vi "DL-SMART-MS-MOTOR-TEST.vi"() -> ()   [LabVIEW 2013]
uses:
  <userlib>/caLab/Private/Put_DBL-1D_PV.vi
  <resource>/objmgr/imaqdx.rc
  <vilib>/Utility/file.llb/Write To Spreadsheet File (DBL).vi
  <userlib>/caLab/Private/Put_I32_PV.vi
  <userlib>/caLab/Private/Get_PV.vi
  <vilib>/Analysis/NI_AALPro.lvlib
  cal_p.vi
  <vilib>/Utility/file.llb/Read From Spreadsheet File (DBL).vi
  <vilib>/Utility/config.llb/NI_LVConfig.lvlib
  <vilib>/Utility/config.llb/Write Key (Double).vi
  <vilib>/Utility/config.llb/Read Key (Double).vi
  <vilib>/Utility/config.llb/Write Key (U32).vi
  <vilib>/Utility/config.llb/Read Key (U32).vi
  <vilib>/Utility/config.llb/Config Data RefNum.ctl
panel:
  out "config":T1 caption="引用句柄"
  in  "stop":bool=TRUE
  out "idn status":string
  out "std sample":T2(array[cluster])
  out "Image":T3(plugin-control)
  out "selected id":i32
  out "selected row":i32
  out "currentNO":string
  out "commet":string
  out "sampleID":string
  in  "chamber in":bool caption="TakeMS"
  in  "chamber out":bool caption="TakeMS"
  in  "ShutDownSystem":bool
  in  "ADC reference":refnum<vi>
  out "Pul.HV-Real":dbl
  out "Identify Spcetrum":cluster{"ID1:X":dbl[], "ID1:Y":dbl[]}[](graph)
  in  "测试记录":i32(listbox)=6
  in  "Identification Results (单靶鉴定结果)":i32(listbox)=2
  in  "HVEnable":bool
  out "GateClose":bool
  out "LaserOK":bool
  out "HV-OK":bool
  out "Vacuum-OK":bool
  in  "Tab Control":T4(tab)
  in  "MCPHV-Set":dbl=1400.0 min=0.0 max=1600.0
  in  "LensHV-Set":dbl=8000.0 min=0.0 max=10000.0
  in  "Tar.HV-Set":dbl=18010.0 min=0.0 max=20000.0
  in  "Pul.HV-Set":dbl=1400.0 min=0.0 max=2000.0
  in  "PulseDelay":dbl
  in  "ADCFreq":dbl
  in  "CH1_Coupling":u64(ring)=2 items=["Volt DC"=1, "Volt AC"=2, "Ampere DC"=4, "Ampere AC"=8, "Ohm"=16]
  in  "Channel 1_Range":dbl(ring)=4.0 items=["80 V"=80.0, "40 V"=40.0, "20 V"=20.0, "8 V"=8.0, "4 V"=4.0, "2 V"=2.0, "800 mV"=0.8, "400 mV"=0.4, "200 mV"=0.2]
  in  "Anal. Setting File":string="High Mass"
  in  "SettingFileSave":bool caption="TakeMS"
  in  "SettingFileAppl":bool caption="TakeMS"
  in  "SettingDel":bool caption="TakeMS"
  in  "RunADC":bool caption="TakeMS"
  in  "Vac_Prot.":bool
  in  "Turbo_Fore":bool
  in  "Main_Samp":bool
  in  "Samp_Atmos":bool
  in  "Fore_Samp":bool
  in  "StartPump":bool
  in  "SopPump":bool
  in  "laser OFF":bool
  in  "laser ON":bool
  in  "laser Deactive":bool
  out "A1-position-Y":dbl=45.0 caption="Y" min=0.0 max=55.0
  out "A1-position-X":dbl=53.4 caption="X" min=0.0 max=55.0
  in  "GO":bool
  in  "Y":dbl min=0.0 max=55.0
  in  "X":dbl min=0.0 max=55.0
  in  "A1-Position":bool caption="X-"
  in  "Plat_To_Zero":bool caption="TakeMS"
  in  "Plat_Cal":bool caption="TakeMS"
  out "Y当前":dbl
  out "X当前":dbl
  out "移动":bool
  out "Y满":bool
  out "Y标":bool
  out "X满":bool
  out "Y0":bool
  out "X0":bool
  out "靶位In/Out":bool
  out "仓门":bool
  out "Y过热":bool
  out "X过热":bool
  out "通讯":bool
  in  "Operation Record":i32(listbox)
  in  "OptionRecordLoad 2":bool caption="TakeMS"
  in  "OptionRecordClear":bool caption="TakeMS"
  out "c:":dbl
  out "b:":dbl
  out "a:":dbl
  in  "cancel cal":bool
  in  "cal save":bool
  in  "peak cal":bool
  in  "peak detect":bool
  in  "标准样品":u16(ring) items=["肺炎克雷伯菌", "铜绿假单胞菌"]
  in  "定标参数":i32(listbox)
  out "Tar.HV-Real":dbl
  out "LensHV-Real":dbl
  out "MCPHV-Real":dbl
  out "Lvaccum":dbl=0.83 format="%#_2e"
  out "Hvaccum":dbl=3.4e-05 format="%#_2e"
  in  "H12":bool
  in  "G12":bool
  in  "F12":bool
  in  "E12":bool
  in  "D12":bool
  in  "C12":bool
  in  "B12":bool
  in  "A12":bool
  in  "H11":bool
  in  "G11":bool
  in  "F11":bool
  in  "E11":bool
  in  "D11":bool
  in  "C11":bool
  in  "B11":bool
  in  "A11":bool
  in  "H10":bool
  in  "G10":bool
  in  "F10":bool
  in  "E10":bool
  in  "D10":bool
  in  "C10":bool
  in  "B10":bool
  in  "A10":bool
  in  "H9":bool
  in  "G9":bool
  in  "F9":bool
  in  "E9":bool
  in  "D9":bool
  in  "C9":bool
  in  "B9":bool
  in  "A9":bool
  in  "H8":bool
  in  "G8":bool
  in  "F8":bool
  in  "E8":bool
  in  "D8":bool
  in  "C8":bool
  in  "B8":bool
  in  "A8":bool
  in  "H7":bool
  in  "G7":bool
  in  "F7":bool
  in  "E7":bool
  in  "D7":bool
  in  "C7":bool
  in  "B7":bool
  in  "A7":bool
  in  "H6":bool
  in  "G6":bool
  in  "F6":bool
  in  "E6":bool
  in  "D6":bool
  in  "C6":bool
  in  "B6":bool
  in  "A6":bool
  in  "H5":bool
  in  "G5":bool
  in  "F5":bool
  in  "E5":bool
  in  "D5":bool
  in  "C5":bool
  in  "B5":bool
  in  "A5":bool
  in  "H4":bool
  in  "G4":bool
  in  "F4":bool
  in  "E4":bool
  in  "D4":bool
  in  "C4":bool
  in  "B4":bool
  in  "A4":bool
  in  "H3":bool
  in  "G3":bool
  in  "F3":bool
  in  "E3":bool
  in  "D3":bool
  in  "C3":bool
  in  "B3":bool
  in  "A3":bool
  in  "H2":bool
  in  "G2":bool
  in  "F2":bool
  in  "E2":bool
  in  "D2":bool
  in  "C2":bool
  in  "B2":bool
  in  "A2":bool
  in  "H1":bool
  in  "G1":bool
  in  "F1":bool
  in  "E1":bool
  in  "D1":bool
  in  "C1":bool
  in  "B1":bool
  in  "A1":bool
  in  "Clear":bool caption="TakeMS"
  in  "Add":bool caption="TakeMS"
  in  "TakeMS-Stop":bool caption="TakeMS"
  in  "TakeMS-Run":bool caption="TakeMS"
  # "Laser (激光)"
  # "光栅"
  # "uJ"
  # "Acq.(采谱)"
  # "Vacuum(真空)"
  # "1"
  # "2"
  # "3"
  # "4"
  # "5"
  # "6"
  # "7"
  # "8"
  # "9"
  # "10"
  # "11"
  # "12"
  # "A"
  # "Pa"
  # "High"
  # "B"
  # "Low"
  # "Pa"
  # "C"
  # "H.V.(高压)"
  # "D"
  # "MCP"
  # "V"
  # "E"
  # "Tar."
  # "V"
  # "F"
  # "Pul."
  # "V"
  # "G"
  # "Lens"
  # "V"
  # "H"
  # "Vauum (真空)"
  # "H.V. (高压)"
  # "Laser (激光)"
  # "Gate (仓门)"
  # "mm"
  # "Radian"
  # "H.V. (高压参数)"
  # "ADC(采集卡设置)"
  # "ADCFreq(采样)"
  # "MCP (探测器)"
  # "V"
  # "Hz"
  # "Tar. (靶)"
  # "V"
  # "Setting File(设置文件)"
  # "Coupling"
  # "Pulse (脉冲)"
  # "V"
  # "IntRange"
  # "V"
  # "Lens (透镜)"
  # "Delay (延时)"
  # "ns"
  # "Sole. Valves"
  # "Turbo Pump"
  # "自锁保护"
  # "机械/分子"
  # "主仓/样仓"
  # "样仓/大气"
  # "机械/样仓"
  # "激光器状态"
  # "mm"
  # "mm"
  # "mm"
  # "mm"
  # "mm"
  # "mm"
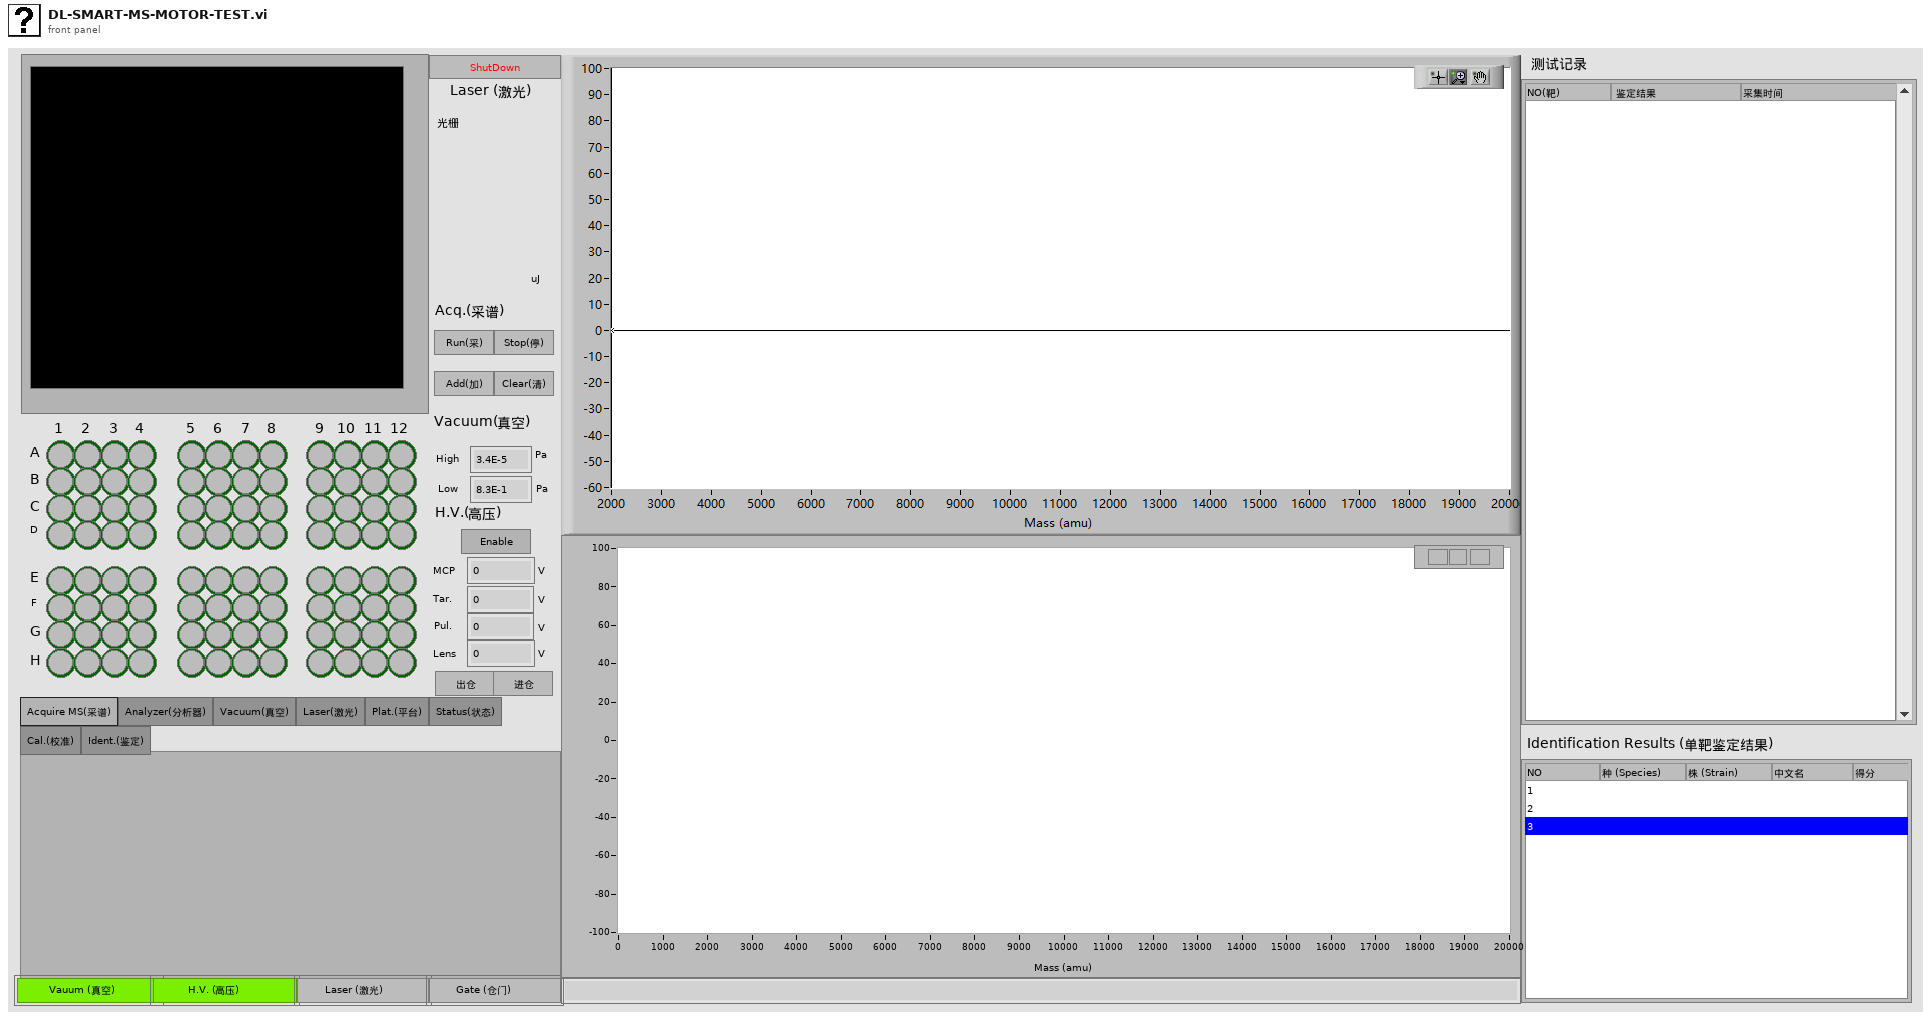
[diagram p1: front panel]
types:
  T1 = typedef "NI_LVConfig.lvlib/Config Data RefNum.ctl" = refnum<k1>
  T2 = cluster{"name":string, "mz":dbl[], "time":dbl[]}[]
  T3 = typedef "IMAQ Image.ctl" = refnum<image>
  T4 = enum32{"Acquire MS(采谱)", "Analyzer(分析器)", "Vacuum(真空)", "Laser(激光)", "Plat.(平台)", "Status(状态)", "Cal.(校准)", "Ident.(鉴定)"}
  T5 = cluster{"tag1":string, "tag2":string, "x":dbl[], "y":dbl[], "ID1:X":dbl[], "ID1:Y":dbl[], "ID1:REF:X":dbl[], "ID1:REF:Y":dbl[], "ID2:X":dbl[], "ID2:Y":dbl[], "ID2:REF:X":dbl[], "ID2:REF:Y":dbl[], "ID3:X":dbl[], "ID3:Y":dbl[], "ID3:REF:X":dbl[], "ID3:REF:Y":dbl[], "ID1:TAG1":string, "ID1:TAG2":string, "ID2:TAG1":string, "ID2:TAG2":string, "ID3:TAG1":string, "ID3:TAG2":string, "ID1:NAME":string, "ID2:NAME":string, "ID3:NAME":string, "ID1:SCORE":string, "ID2:SCORE":string, "ID3:SCORE":string, "NO":string}[]
  T6 = enum8{"Enabled", "Disabled", "Disabled and Grayed Out"}
  T7 = typedef "Semaphore RefNum" = refnum<k1>
  T8 = cluster{"monitor":refnum<user-event>, "motor status":refnum<user-event>, "motor":refnum<user-event>, "notifier out":refnum<notifier>, "queue out":refnum<queue>, "AI":T7, "DI":T7, "CX":T7, "CY":T7}
  T9 = cluster{"AI Task":refnum<k21>, "AO Task":refnum<k21>, "DO Task":refnum<k21>, "DI Task":refnum<k21>, "PWM x":refnum<k21>, "PWM y":refnum<k21>, "counter x":refnum<k21>, "counter y":refnum<k21>}
  T10 = cluster{"tasks":cluster{"AI Task":refnum<k21>, "AO Task":refnum<k21>, "DO Task":refnum<k21>, "DI Task":refnum<k21>, "PWM x":refnum<k21>, "PWM y":refnum<k21>, "counter x":refnum<k21>, "counter y":refnum<k21>}, "interface":cluster{"monitor":refnum<user-event>, "motor status":refnum<user-event>, "motor":refnum<user-event>, "notifier out":refnum<notifier>, "queue out":refnum<queue>, "AI":T7, "DI":T7, "CX":T7, "CY":T7}, "error out":errorcluster}
  T11 = typedef "LVPoint32TypeDef.ctl" = cluster{"Horizontal":i32, "Vertical":i32}
  T12 = cluster{"tag1":string, "tag2":string, "x":dbl[], "y":dbl[], "ID1:X":dbl[], "ID1:Y":dbl[], "ID1:REF:X":dbl[], "ID1:REF:Y":dbl[], "ID2:X":dbl[], "ID2:Y":dbl[], "ID2:REF:X":dbl[], "ID2:REF:Y":dbl[], "ID3:X":dbl[], "ID3:Y":dbl[], "ID3:REF:X":dbl[], "ID3:REF:Y":dbl[], "ID1:TAG1":string, "ID1:TAG2":string, "ID2:TAG1":string, "ID2:TAG2":string, "ID3:TAG1":string, "ID3:TAG2":string, "ID1:NAME":string, "ID2:NAME":string, "ID3:NAME":string, "ID1:SCORE":string, "ID2:SCORE":string, "ID3:SCORE":string, "NO":string}
  T13 = typedef "LVRowAndColumnTypeDef.ctl" = cluster{"Row":i32, "Column":i32}
  T14 = cluster{"Type":u32, "Version":u32, "Flags":u32, "SerialNumberHigh":u32, "SerialNumberLow":u32, "BusType":u32, "InterfaceName":string, "VendorName":string, "ModelName":string, "CameraFileName":string, "CameraAttributeURL":string}[]
  T15 = cluster{"Type":u32, "Version":u32, "Flags":u32, "SerialNumberHigh":u32, "SerialNumberLow":u32, "BusType":u32, "InterfaceName":string, "VendorName":string, "ModelName":string, "CameraFileName":string, "CameraAttributeURL":string}
  T16 = typedef "IMAQdx.ctl" = refnum<k21>
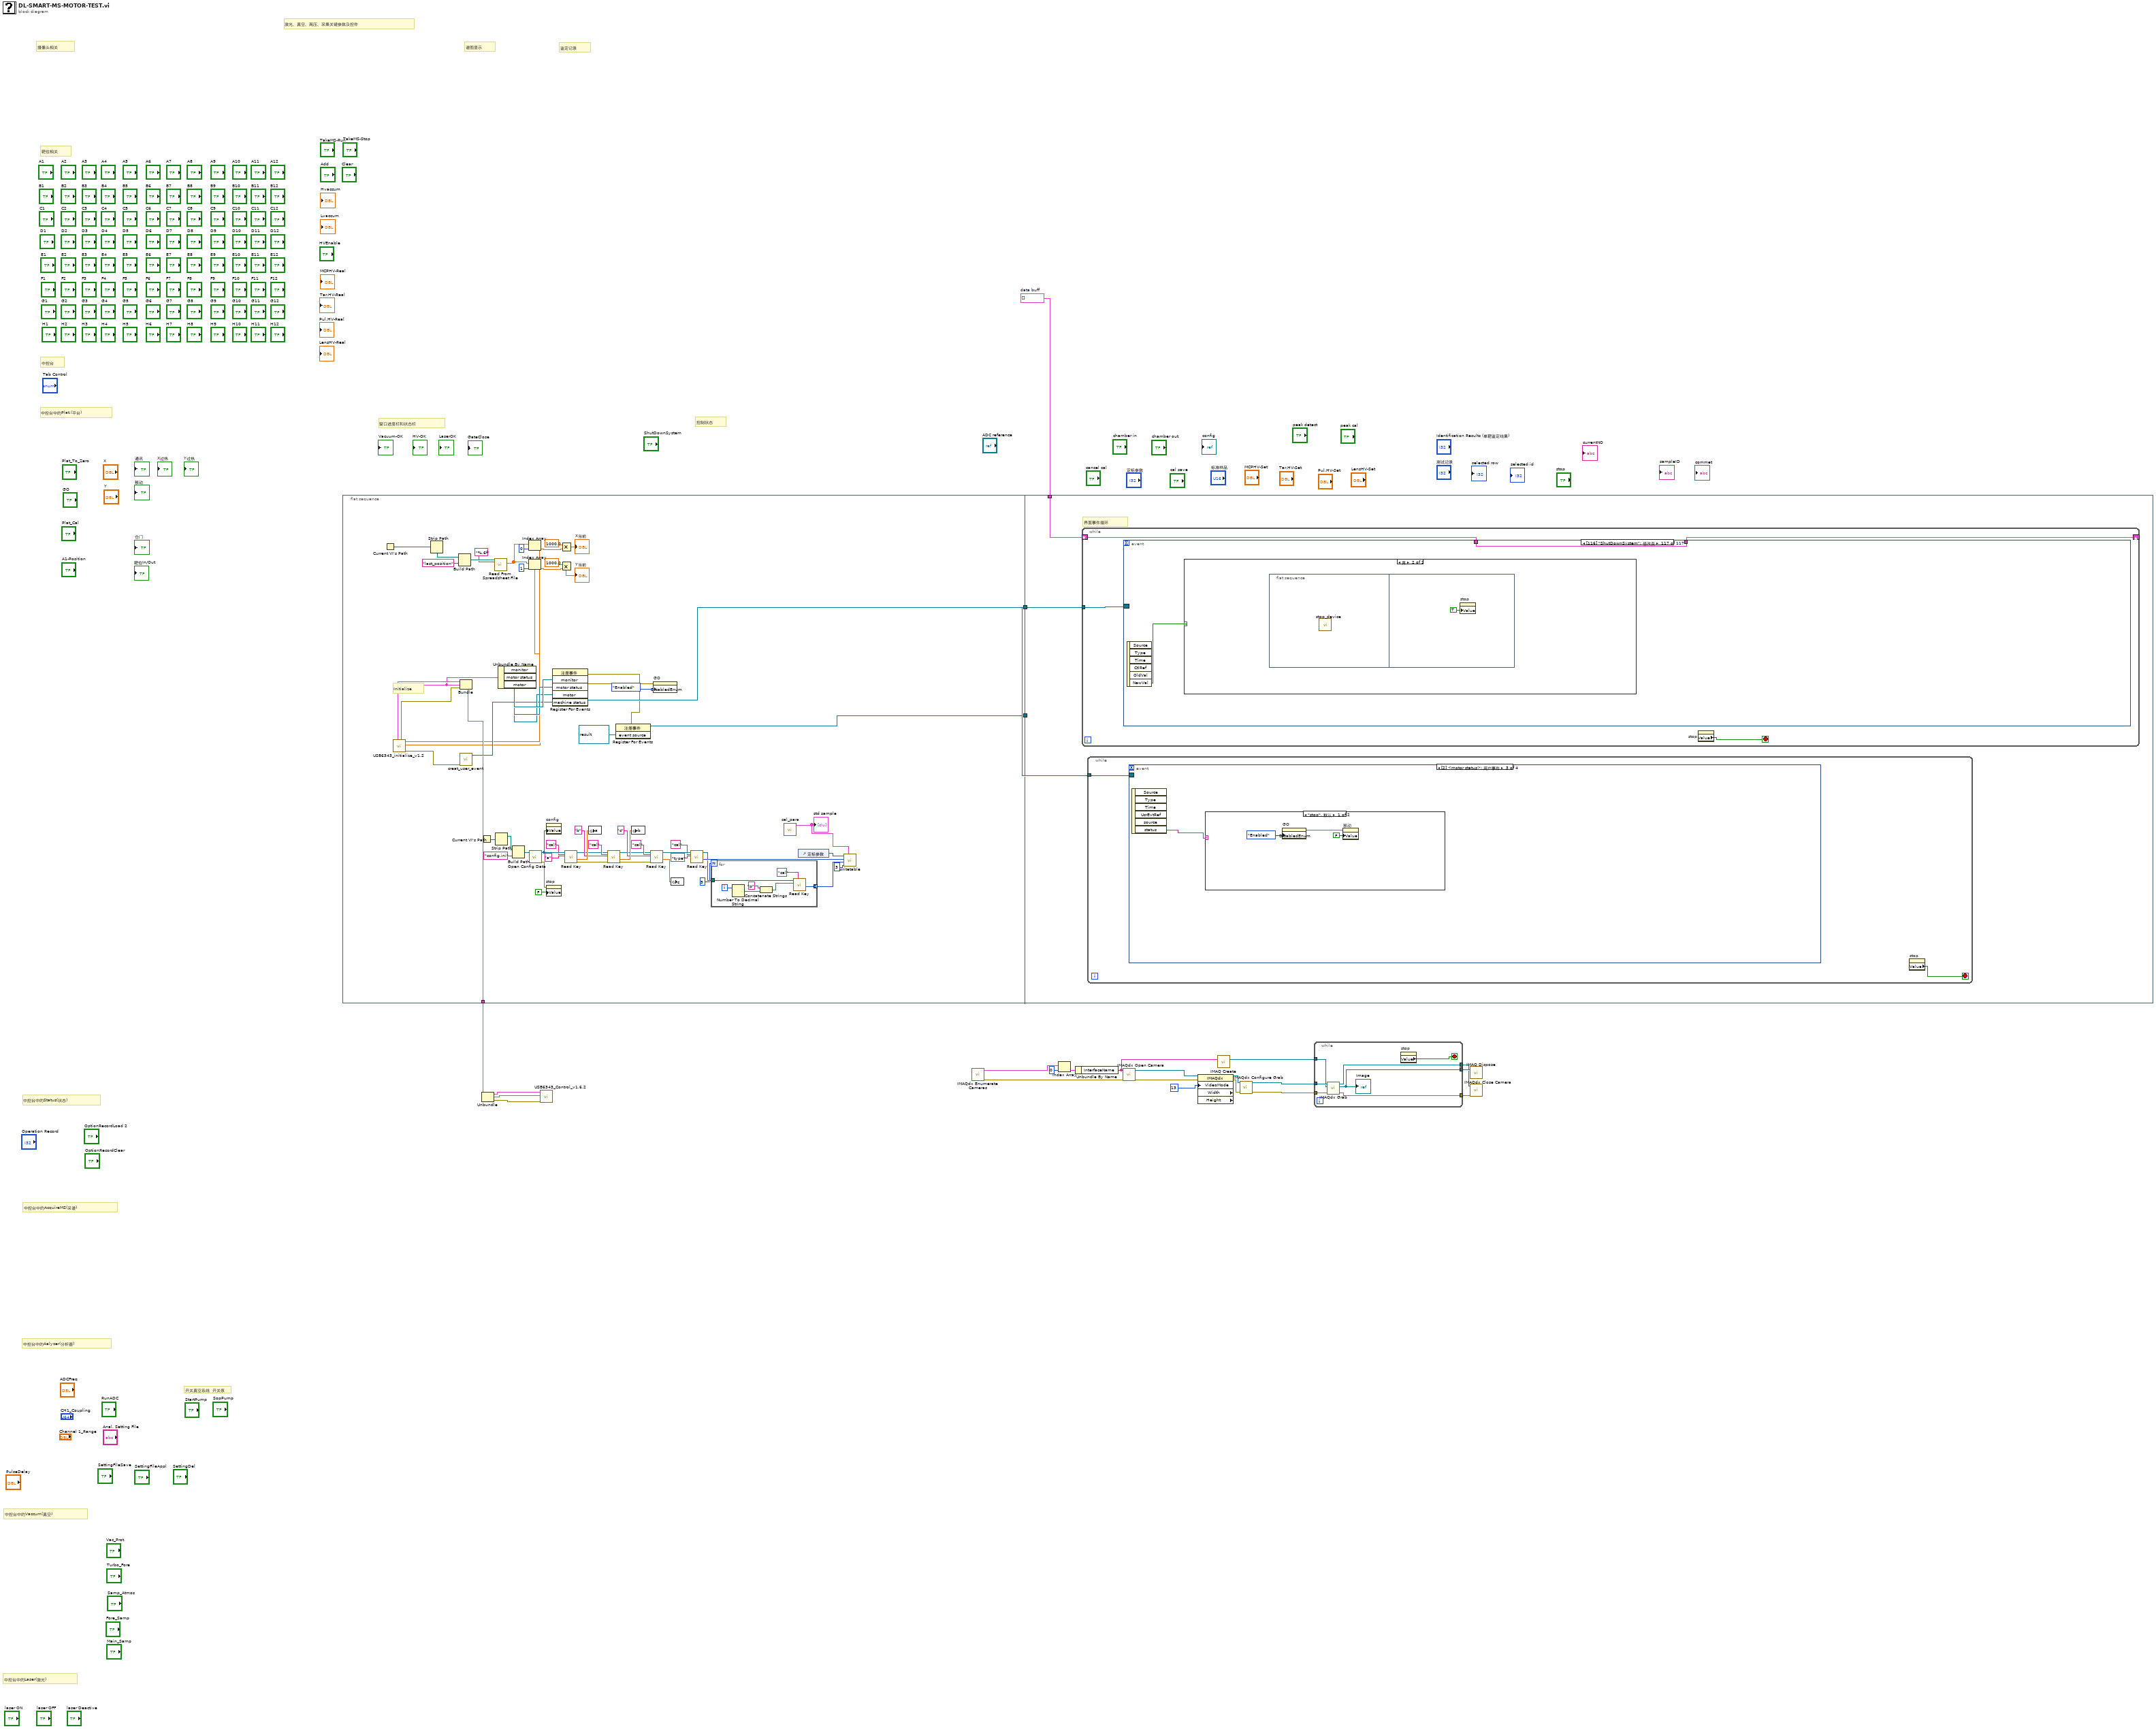
[diagram p0: block diagram]
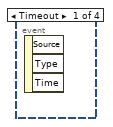
[diagram p2: hidden frame]
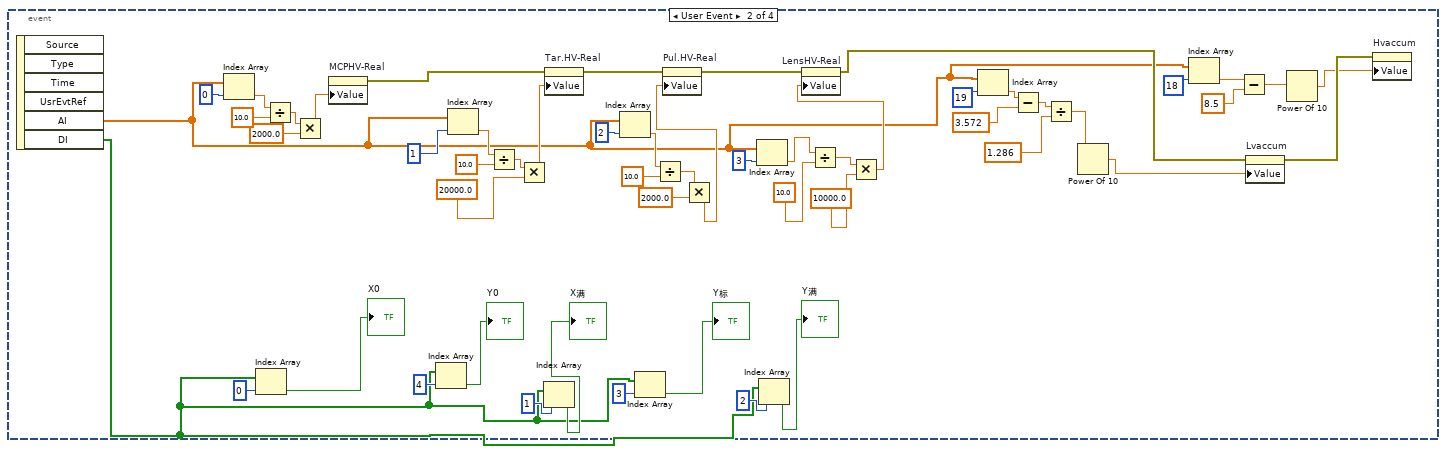
[diagram p3: hidden frame]
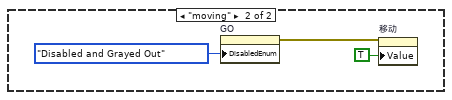
[diagram p4: hidden frame]
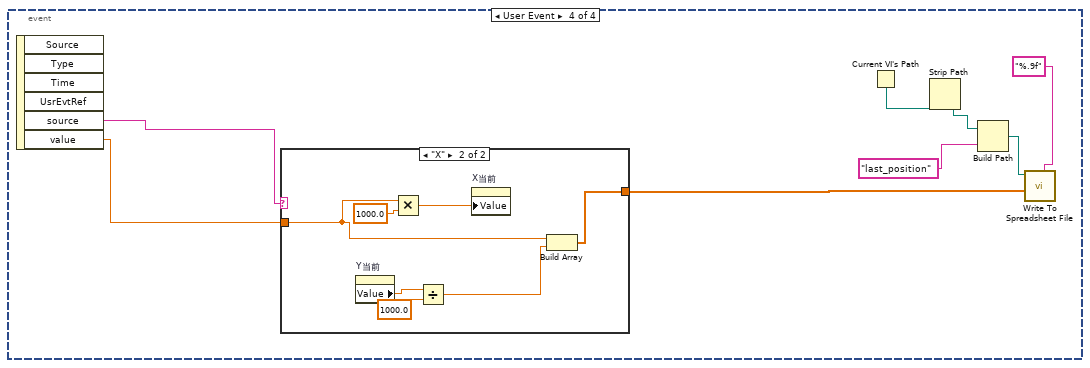
[diagram p5: hidden frame]
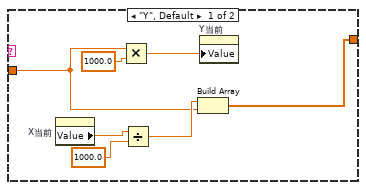
[diagram p6: hidden frame]
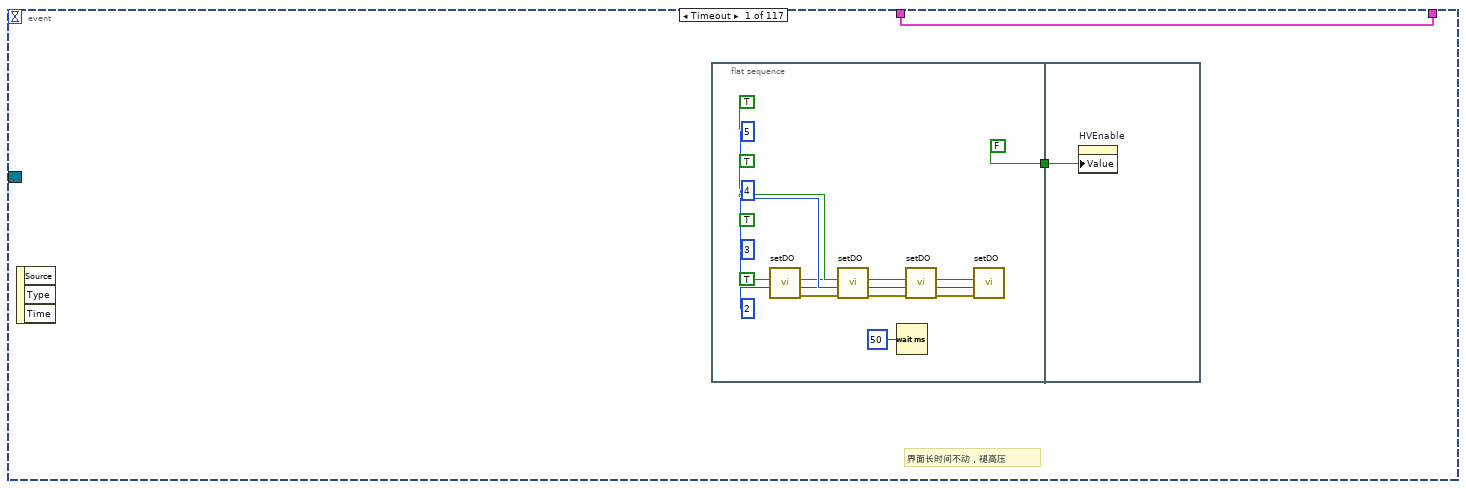
[diagram p7: hidden frame]
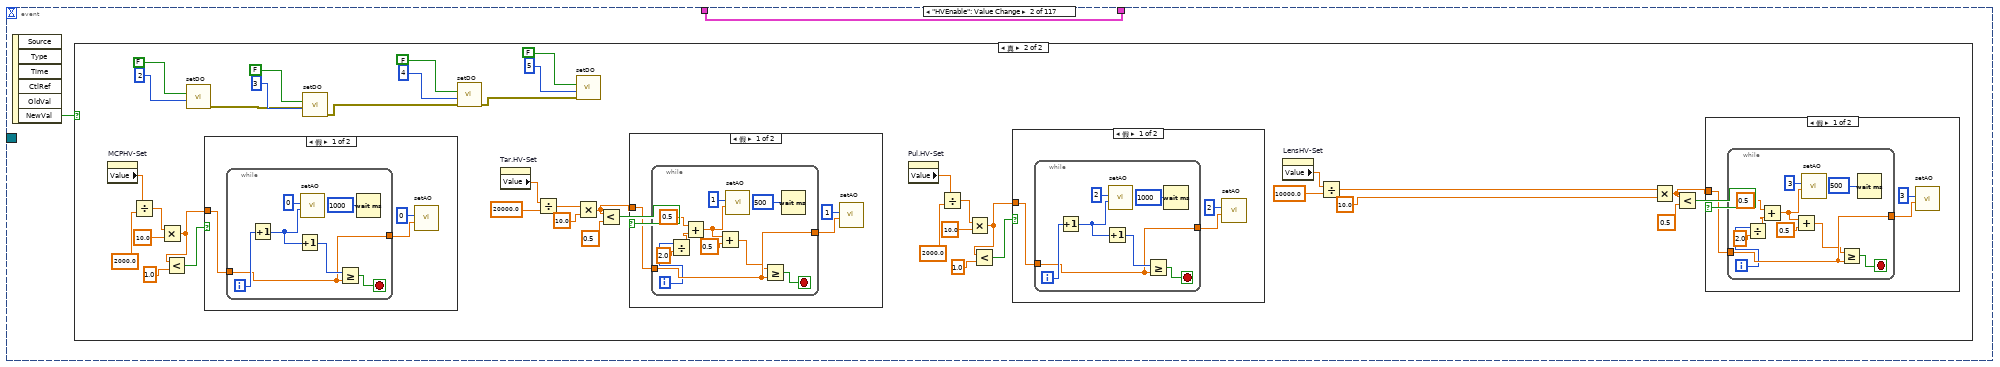
[diagram p8: hidden frame]
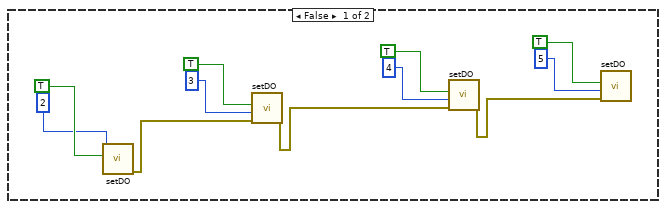
[diagram p9: hidden frame]
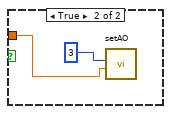
[diagram p10: hidden frame]
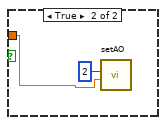
[diagram p11: hidden frame]
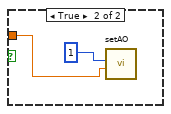
[diagram p12: hidden frame]
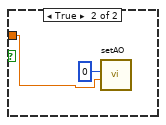
[diagram p13: hidden frame]
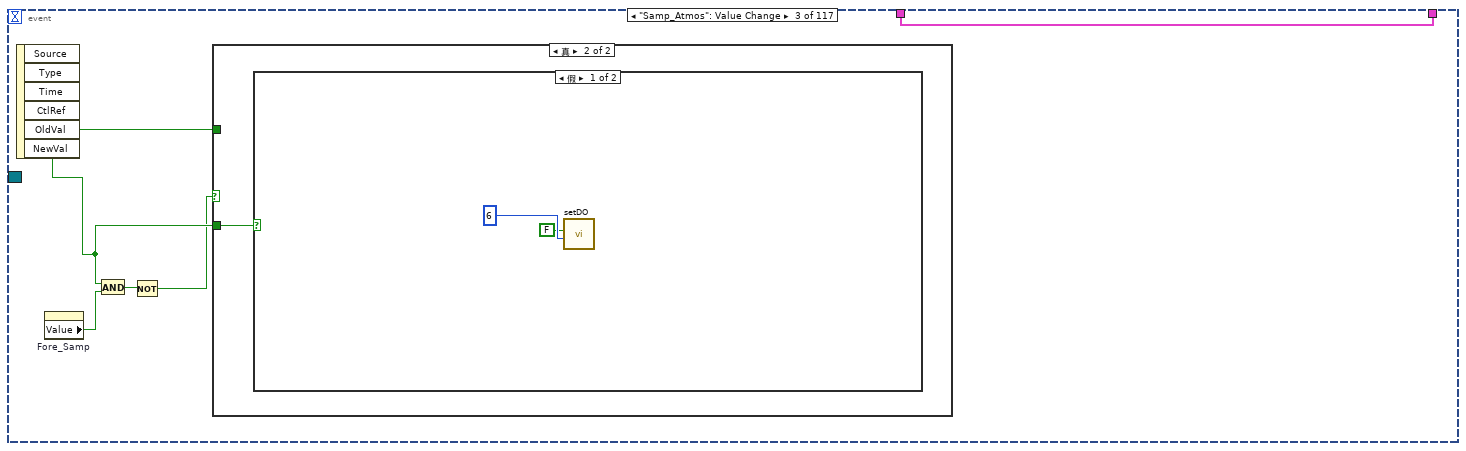
[diagram p14: hidden frame]
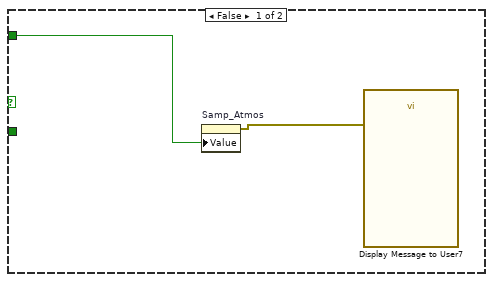
[diagram p15: hidden frame]
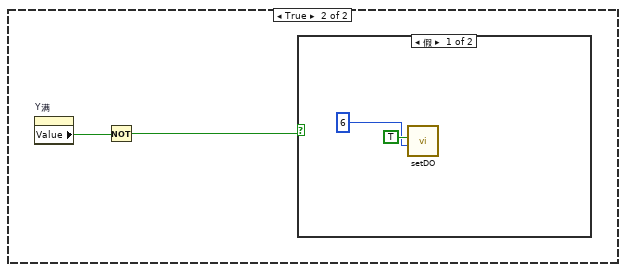
[diagram p16: hidden frame]
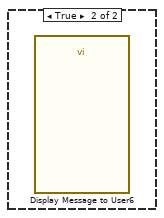
[diagram p17: hidden frame]
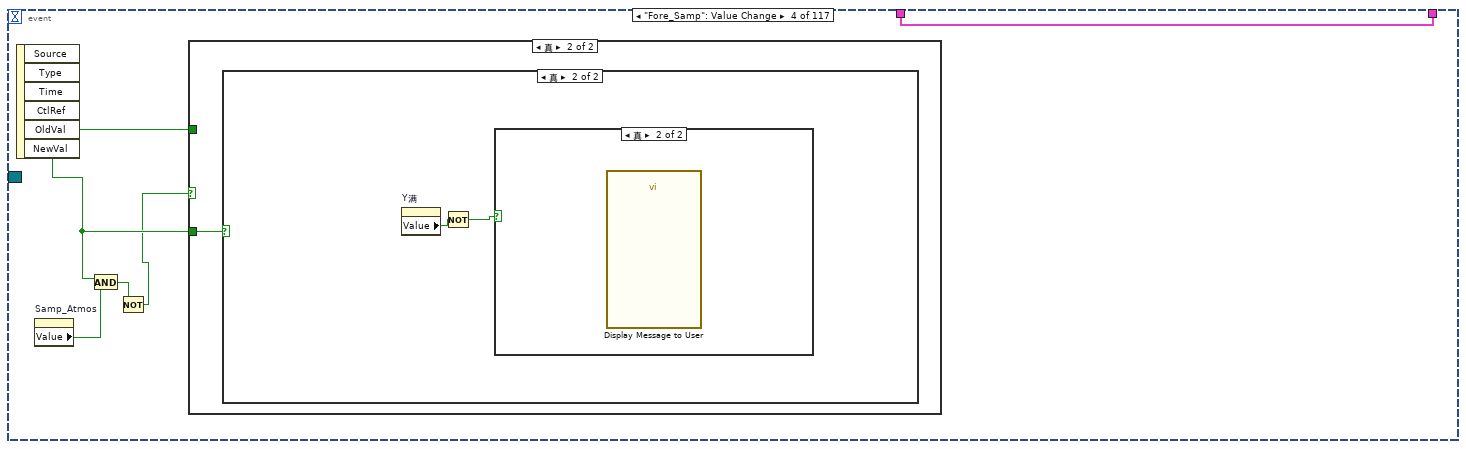
[diagram p18: hidden frame]
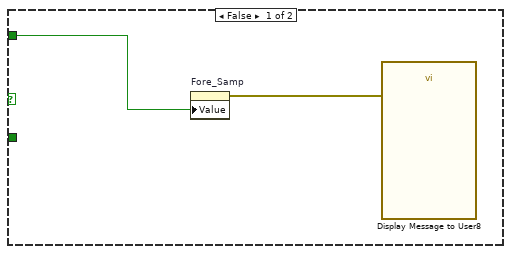
[diagram p19: hidden frame]
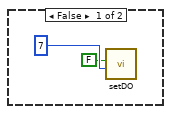
[diagram p20: hidden frame]
diagram:
  w21 = T5 []  # data buff
  # "开关真空系统  开关泵"
  # "控制状态"
  # "鉴定记录"
  # "谱图显示"
  # "激光、真空、高压、采集关键参数及控件"
  # "窗口进度栏和状态栏"
  # "中控台中的Laser(激光)"
  # "中控台中的Vaccum(真空)"
  # "中控台中的Aalyzer(分析器)"
  # "中控台中的AcquireMS(采谱)"
  # "中控台中的Status(状态)"
  # "中控台中的Plat.(平台)"
  # "中控台"
  # "靶位相关"
  # "摄像头相关"
  n1 = flat-sequence {
    tunnel: [w58] -> w23
    tunnel: [w73] -> w22
    tunnel: [w53] -> w1
    tunnel: w23 -> [w90]
    tunnel: w21 -> [w91]
    tunnel: w1 -> [w89]
    frame #0 {
      # "Initialize"
      n2 = Current VI's Path() -> (path=w72:path)
      n3 = Strip Path(path=w72) -> (stripped path=w71:path)  [unwired: 1 out]
      n4 = Build Path(base path=w71, name or relative path="last_position") -> (appended path=w69:path)
      n5 = Current VI's Path() -> (path=w50:path)
      n6 = call-poly <vilib>:"Read From Spreadsheet File.vi"("format (%.3f)"="%.6f", "file path (dialog if empty)"=w69) -> ("first row"=w67:dbl[])  [unwired: 5 in, 4 out]
      n7 = Strip Path(path=w50) -> (stripped path=w49:path)  [unwired: 1 out]
      n8 = Build Path(base path=w49, name or relative path="config.ini" ("名称或相对路径")) -> (appended path=w47:path)
      n9 = Index Array(array=w67, index=0) -> (element=w64:dbl)
      n10 = Index Array(array=w67, index=1) -> (element=w61:dbl)
      n11 = call "USB6343_initialize_v1.2.vi"("Y initial position"=w61, "X initial position"=w64) -> ("error out"=w74:errorcluster, "interface"=w75:T8, "tasks"=w76:T9)  [unwired: 7 in]
      n12 = Bundle("tasks"=w76, "interface"=w75, "error out"=w74) -> (w73:T10)  [unwired: 1 in]
      n13 = call "creat_user_event.vi"("error in (no error)"=w74) -> ("machine status"=w77:refnum<user-event>)  [unwired: 9 in, 1 out]
      n14 = Unbundle By Name(w75) -> ("monitor"=w81:refnum<user-event>, "motor status"=w80:refnum<user-event>, "motor"=w79:refnum<user-event>)
      n15 = call <vilib>:"Open Config Data.vi"("configuration file path"=w47) -> ("error out"=w46:errorcluster, "refnum"=w45:T1)  [unwired: 8 in, 1 out]
      n16 = property on="config" class="TypRef (严格)"("Value"=w45) -> ()  [unwired: 2 in, 2 out]
      n17 = property on="stop" class="Bool (严格)"(error in=w46, "Value"=FALSE ("ShutDownSystem")) -> ()  [unwired: 1 in, 2 out]
      n18 = Multiply(x=1000.0, y=w64) -> (x*y=→"X当前":dbl)
      n19 = Multiply(x=1000.0, y=w61) -> (x*y=→"Y当前":dbl)
      n20 = call-poly <vilib>:"Read Key.vi"("section"="cal", "key"="a", "refnum"=w45) -> ("error out"=w37:errorcluster, "value"=w42:dbl, "refnum out"=w38:T1)  [unwired: 5 in, 1 out]
      n21 = global write "cal_p.vi" "a"(w42) -> ()
      n22 = call-poly <vilib>:"Read Key.vi"("section"="cal", "error in (no error)"=w37, "key"="b", "refnum"=w38) -> ("error out"=w33:errorcluster, "value"=w39:dbl, "refnum out"=w32:T1)  [unwired: 4 in, 1 out]
      n23 = register-events(refnum<user-event> refnum ("event source")) -> (reference out=w53:refnum<event-registration>, error out=w52:errorcluster)  [unwired: 2 in]
      n24 = register-events(error in=w52, w81, w80, w79, w77) -> (reference out=w58:refnum<event-registration>, error out=w57:errorcluster)  [unwired: 1 in]
      n25 = global write "cal_p.vi" "b"(w39) -> ()
      n26 = call-poly <vilib>:"Read Key.vi"("section"="cal", "error in (no error)"=w33, "key"="c", "refnum"=w32) -> ("value"=w34:dbl, "refnum out"=w31:T1)  [unwired: 4 in, 2 out]
      n27 = property on="GO" class="Bool (严格)"(error in=w57, "DisabledEnum"=T6."Enabled" ("Disabled")) -> ()  [unwired: 1 in, 2 out]
      n28 = global write "cal_p.vi" "c"(w34) -> ()
      n29 = call-poly <vilib>:"Read Key.vi"("section"="cal", "key"="type", "refnum"=w31) -> ("value"=w28:u32, "refnum out"=w27:T1)  [unwired: 5 in, 2 out]
      n30 = for {
        N: 5 -> [_]
        tunnel: w27 -> [w88]
        tunnel: [w82] -> w25 mode=indexing
        i -> [w86]
        n31 = Number To Decimal String(number=w86) -> (decimal integer string=w85:string)  [unwired: 1 in]
        n32 = Concatenate Strings("p", w85) -> (w83:string)
        n33 = call-poly <vilib>:"Read Key.vi"("section"="cal", "key"=w83, "refnum"=w88) -> ("value"=w82:u32)  [unwired: 5 in, 3 out]
      }
      n34 = call "cal_para.vi"() -> ("std sample"=w55:T2)  [unwired: 11 in]
      "std sample" <- w55
      n35 = control-ref of="定标参数"() -> (w56:refnum<vi>)
      n36 = call "writetable.vi"("std sample"=w55, "col"=3, "Array in"=w25, "type"=w28, "reference"=w56) -> ()  [unwired: 7 in]
    }
    frame #1 {
      # "界面事件循环"
      n37 = while {
        tunnel: w89 -> [w179]
        shift-right: [w177] -> _
        shift-left: w91 -> [w178]
        stop <- w176 stop-if-true
        n38 = event shown="[116] \"ShutDownSystem\": 值改变" {
          selector: w179 -> [_ _ _ _ _ _ _ _ _ _ _ _ _ _ _ _ _ _ _ _ _ _ _ _ _ _ _ _ _ _ _ _ _ _ _ _ _ _ _ _ _ _ _ _ _ _ _ _ _ _ _ _ _ _ _ _ _ _ _ _ _ _ _ _ _ _ _ _ _ _ _ _ _ _ _ _ _ _ _ _ _ _ _ _ _ _ _ _ _ _ _ _ _ _ _ _ _ _ _ _ _ _ _ _ _ _ _ _ _ _ _ _ _ _ _ _ _]
          dyn-events: _ -> [_ _ _ _ _ _ _ _ _ _ _ _ _ _ _ _ _ _ _ _ _ _ _ _ _ _ _ _ _ _ _ _ _ _ _ _ _ _ _ _ _ _ _ _ _ _ _ _ _ _ _ _ _ _ _ _ _ _ _ _ _ _ _ _ _ _ _ _ _ _ _ _ _ _ _ _ _ _ _ _ _ _ _ _ _ _ _ _ _ _ _ _ _ _ _ _ _ _ _ _ _ _ _ _ _ _ _ _ _ _ _ _ _ _ _ _ _]
          timeout: _ -> [_ _ _ _ _ _ _ _ _ _ _ _ _ _ _ _ _ _ _ _ _ _ _ _ _ _ _ _ _ _ _ _ _ _ _ _ _ _ _ _ _ _ _ _ _ _ _ _ _ _ _ _ _ _ _ _ _ _ _ _ _ _ _ _ _ _ _ _ _ _ _ _ _ _ _ _ _ _ _ _ _ _ _ _ _ _ _ _ _ _ _ _ _ _ _ _ _ _ _ _ _ _ _ _ _ _ _ _ _ _ _ _ _ _ _ _ _]
          tunnel: w178 -> [w180 w196 w304 w319 w334 w341 w348 w355 w364 w380 w410 w445 w484 w486 w493 w528 w566 w568 w618 w623 w639 w657 w674 w691 w708 w725 w744 w769 w786 w803 w820 w837 w854 w873 w892 w911 w930 w949 w968 w987 w1006 w1025 w1044 w1063 w1082 w1101 w1120 w1139 w1158 w1177 w1196 w1215 w1234 w1253 w1272 w1291 w1310 w1329 w1348 w1367 w1386 w1405 w1424 w1447 w1466 w1485 w1504 w1523 w1542 w1561 w1580 w1599 w1618 w1637 w1656 w1675 w1694 w1713 w1732 w1751 w1770 w1789 w1808 w1827 w1846 w1865 w1884 w1903 w1922 w1941 w1960 w1979 w1998 w2017 w2036 w2055 w2074 w2093 w2112 w2131 w2150 w2169 w2188 w2207 w2226 w2245 w2264 w2283 w2302 w2321 w2340 w2359 w2378 w2397 w2416 w2435 w2449]
          tunnel: [w180 w196 w304 w319 w334 w341 w348 w355 w364 w379 w410 w445 w484 w486 w493 w528 w566 w568 w618 w623 w639 w657 w674 w691 w708 w725 w743 w769 w786 w803 w820 w837 w854 w873 w892 w911 w930 w949 w968 w987 w1006 w1025 w1044 w1063 w1082 w1101 w1120 w1139 w1158 w1177 w1196 w1215 w1234 w1253 w1272 w1291 w1310 w1329 w1348 w1367 w1386 w1405 w1424 w1447 w1466 w1485 w1504 w1523 w1542 w1561 w1580 w1599 w1618 w1637 w1656 w1675 w1694 w1713 w1732 w1751 w1770 w1789 w1808 w1827 w1846 w1865 w1884 w1903 w1922 w1941 w1960 w1979 w1998 w2017 w2036 w2055 w2074 w2093 w2112 w2131 w2150 w2169 w2188 w2207 w2226 w2245 w2264 w2283 w2302 w2321 w2340 w2359 w2378 w2397 w2416 w2435 w2449] -> w177
          event Timeout {
            # "界面长时间不动，褪高压"
            n39 = event-data() -> ()  [unwired: 1 in, 3 out]
            n40 = flat-sequence {
              tunnel: [FALSE ("HVEnable")] -> w181
              tunnel: w181 -> [w195]
              frame #0 {
                n41 = call "setDO.vi"("channel"=2, "on/off"=TRUE) -> ("错误输出"=w192:errorcluster)  [unwired: 9 in]
                n42 = call "setDO.vi"("错误输入（无错误）"=w192, "channel"=3, "on/off"=TRUE) -> ("错误输出"=w193:errorcluster)  [unwired: 8 in]
                n43 = Wait (ms)(milliseconds to wait=u32 50) -> ()  [unwired: 1 out]
                n44 = call "setDO.vi"("错误输入（无错误）"=w193, "channel"=4, "on/off"=TRUE) -> ("错误输出"=w194:errorcluster)  [unwired: 8 in]
                n45 = call "setDO.vi"("错误输入（无错误）"=w194, "channel"=5, "on/off"=TRUE) -> ()  [unwired: 8 in, 1 out]
              }
              frame #1 {
                n46 = property on="HVEnable" class="Bool (严格)"("Value"=w195) -> ()  [unwired: 2 in, 2 out]
              }
            }
          }
          event "HVEnable": Value Change {
            n47 = event-data() -> ("NewVal"=w197:bool)  [unwired: 1 in, 5 out]
            n48 = case shown="真" w197 {
              frame False {
                n49 = call "setDO.vi"("channel"=2, "on/off"=TRUE) -> ("错误输出"=w200:errorcluster)  [unwired: 9 in]
                n50 = call "setDO.vi"("错误输入（无错误）"=w200, "channel"=3, "on/off"=TRUE) -> ("错误输出"=w199:errorcluster)  [unwired: 8 in]
                n51 = call "setDO.vi"("错误输入（无错误）"=w199, "channel"=4, "on/off"=TRUE) -> ("错误输出"=w198:errorcluster)  [unwired: 8 in]
                n52 = call "setDO.vi"("错误输入（无错误）"=w198, "channel"=5, "on/off"=TRUE) -> ()  [unwired: 8 in, 1 out]
              }
              frame True {
                n53 = property on="MCPHV-Set" class="DigNum (严格)"() -> ("Value"=w233:dbl)  [unwired: 2 in, 2 out]
                n54 = Divide(x=w233, y=2000.0) -> (x/y=w235:dbl)
                n55 = Multiply(x=w235, y=10.0) -> (x*y=w226:dbl)
                n56 = Less?(x=w226, y=1.0) -> (x < y?=w227:bool)
                n57 = call "setDO.vi"("channel"=2, "on/off"=FALSE) -> ("错误输出"=w239:errorcluster)  [unwired: 9 in]
                n58 = case shown="假" w227 {
                  tunnel: w226 -> [w294 w302]
                  frame False {
                    n59 = while {
                      tunnel: w294 -> [w296]
                      tunnel: [w296] -> w292
                      i -> [w300]
                      stop <- w297 stop-if-true
                      n60 = Increment(x=w300) -> (x+1=w299:i32)
                      n61 = Increment(x=w299) -> (x+1=w298:i32)
                      n62 = call "setAO.vi"("value"=w299, "channel"=0) -> ()  [unwired: 9 in, 1 out]
                      n63 = Greater Or Equal?(x=w298, y=w296) -> (x >= y?=w297:bool)
                      n64 = Wait (ms)(milliseconds to wait=1000) -> ()  [unwired: 1 out]
                    }
                    n65 = call "setAO.vi"("value"=w292, "channel"=0) -> ()  [unwired: 9 in, 1 out]
                  }
                  frame True {
                    n66 = call "setAO.vi"("value"=w302, "channel"=0) -> ()  [unwired: 9 in, 1 out]
                  }
                }
                n67 = call "setDO.vi"("错误输入（无错误）"=w239, "channel"=3, "on/off"=FALSE) -> ("错误输出"=w238:errorcluster)  [unwired: 8 in]
                n68 = call "setDO.vi"("错误输入（无错误）"=w238, "channel"=4, "on/off"=FALSE) -> ("错误输出"=w237:errorcluster)  [unwired: 8 in]
                n69 = property on="Tar.HV-Set" class="DigNum (严格)"() -> ("Value"=w229:dbl)  [unwired: 2 in, 2 out]
                n70 = Divide(x=w229, y=20000.0) -> (x/y=w231:dbl)
                n71 = call "setDO.vi"("错误输入（无错误）"=w237, "channel"=5, "on/off"=FALSE) -> ()  [unwired: 8 in, 1 out]
                n72 = Multiply(x=w231, y=10.0) -> (x*y=w223:dbl)
                n73 = Less?(x=w223, y=0.5) -> (x < y?=w224:bool)
                n74 = case shown="假" w224 {
                  tunnel: w223 -> [w278 w290]
                  frame False {
                    n75 = while {
                      tunnel: w278 -> [w287]
                      tunnel: [w287] -> w276
                      i -> [w283]
                      stop <- w288 stop-if-true
                      n76 = Divide(x=w283, y=2.0) -> (x/y=w284:dbl)
                      n77 = Add(x=0.5, y=w284) -> (x+y=w281:dbl)
                      n78 = Add(x=w281, y=0.5) -> (x+y=w279:dbl)
                      n79 = call "setAO.vi"("value"=w281, "channel"=1) -> ()  [unwired: 9 in, 1 out]
                      n80 = Greater Or Equal?(x=w279, y=w287) -> (x >= y?=w288:bool)
                      n81 = Wait (ms)(milliseconds to wait=500) -> ()  [unwired: 1 out]
                    }
                    n82 = call "setAO.vi"("value"=w276, "channel"=1) -> ()  [unwired: 9 in, 1 out]
                  }
                  frame True {
                    n83 = call "setAO.vi"("value"=w290, "channel"=1) -> ()  [unwired: 9 in, 1 out]
                  }
                }
                n84 = property on="Pul.HV-Set" class="DigNum (严格)"() -> ("Value"=w222:dbl)  [unwired: 2 in, 2 out]
                n85 = Divide(x=w222, y=2000.0) -> (x/y=w217:dbl)
                n86 = Multiply(x=w217, y=10.0) -> (x*y=w221:dbl)
                n87 = Less?(x=w221, y=1.0) -> (x < y?=w220:bool)
                n88 = case shown="假" w220 {
                  tunnel: w221 -> [w266 w274]
                  frame False {
                    n89 = while {
                      tunnel: w266 -> [w268]
                      tunnel: [w268] -> w264
                      i -> [w272]
                      stop <- w269 stop-if-true
                      n90 = Increment(x=w272) -> (x+1=w271:i32)
                      n91 = Increment(x=w271) -> (x+1=w270:i32)
                      n92 = call "setAO.vi"("value"=w271, "channel"=2) -> ()  [unwired: 9 in, 1 out]
                      n93 = Greater Or Equal?(x=w270, y=w268) -> (x >= y?=w269:bool)
                      n94 = Wait (ms)(milliseconds to wait=1000) -> ()  [unwired: 1 out]
                    }
                    n95 = call "setAO.vi"("value"=w264, "channel"=2) -> ()  [unwired: 9 in, 1 out]
                  }
                  frame True {
                    n96 = call "setAO.vi"("value"=w274, "channel"=2) -> ()  [unwired: 9 in, 1 out]
                  }
                }
                n97 = property on="LensHV-Set" class="DigNum (严格)"() -> ("Value"=w215:dbl)  [unwired: 2 in, 2 out]
                n98 = Divide(x=w215, y=10000.0) -> (x/y=w210:dbl)
                n99 = Multiply(x=w210, y=10.0) -> (x*y=w214:dbl)
                n100 = Less?(x=w214, y=0.5) -> (x < y?=w213:bool)
                n101 = case shown="假" w213 {
                  tunnel: w214 -> [w250 w262]
                  frame False {
                    n102 = while {
                      tunnel: w250 -> [w259]
                      tunnel: [w259] -> w248
                      i -> [w255]
                      stop <- w260 stop-if-true
                      n103 = Divide(x=w255, y=2.0) -> (x/y=w256:dbl)
                      n104 = Add(x=0.5, y=w256) -> (x+y=w253:dbl)
                      n105 = Add(x=w253, y=0.5) -> (x+y=w251:dbl)
                      n106 = call "setAO.vi"("value"=w253, "channel"=3) -> ()  [unwired: 9 in, 1 out]
                      n107 = Greater Or Equal?(x=w251, y=w259) -> (x >= y?=w260:bool)
                      n108 = Wait (ms)(milliseconds to wait=500) -> ()  [unwired: 1 out]
                    }
                    n109 = call "setAO.vi"("value"=w248, "channel"=3) -> ()  [unwired: 9 in, 1 out]
                  }
                  frame True {
                    n110 = call "setAO.vi"("value"=w262, "channel"=3) -> ()  [unwired: 9 in, 1 out]
                  }
                }
              }
            }
          }
          event "Samp_Atmos": Value Change {
            n111 = event-data() -> ("OldVal"=w305:bool, "NewVal"=w309:bool)  [unwired: 1 in, 4 out]
            n112 = property on="Fore_Samp" class="Bool (严格)"() -> ("Value"=w308:bool)  [unwired: 2 in, 2 out]
            n113 = And(x=w309, y=w308) -> (x .and. y?=w307:bool)
            n114 = Not(x=w307) -> (.not. x?=w306:bool)
            n115 = case shown="真" w306 {
              tunnel: w309 -> [_ w312]
              tunnel: w305 -> [w311 _]
              frame False {
                n116 = property on="Samp_Atmos" class="Bool (严格)"("Value"=w311) -> (error out=w310:errorcluster)  [unwired: 2 in, 1 out]
                n117 = call "Display Message to User7"("error in (no error)"=w310) -> ()  [unwired: 9 in, 2 out]
              }
              frame True {
                n118 = case shown="假" w312 {
                  frame False {
                    n119 = call "setDO.vi"("channel"=6, "on/off"=FALSE) -> ()  [unwired: 9 in, 1 out]
                  }
                  frame True {
                    n120 = property on="Y满" class="Bool (严格)"() -> ("Value"=w316:bool)  [unwired: 2 in, 2 out]
                    n121 = Not(x=w316) -> (.not. x?=w315:bool)
                    n122 = case shown="假" w315 {
                      frame False {
                        n123 = call "setDO.vi"("channel"=6, "on/off"=TRUE) -> ()  [unwired: 9 in, 1 out]
                      }
                      frame True {
                        n124 = call "Display Message to User6"() -> ()  [unwired: 10 in, 2 out]
                      }
                    }
                  }
                }
              }
            }
          }
          event "Fore_Samp": Value Change {
            n125 = event-data() -> ("OldVal"=w320:bool, "NewVal"=w324:bool)  [unwired: 1 in, 4 out]
            n126 = property on="Samp_Atmos" class="Bool (严格)"() -> ("Value"=w323:bool)  [unwired: 2 in, 2 out]
            n127 = And(x=w324, y=w323) -> (x .and. y?=w322:bool)
            n128 = Not(x=w322) -> (.not. x?=w321:bool)
            n129 = case shown="真" w321 {
              tunnel: w324 -> [_ w327]
              tunnel: w320 -> [w326 _]
              frame False {
                n130 = property on="Fore_Samp" class="Bool (严格)"("Value"=w326) -> (error out=w325:errorcluster)  [unwired: 2 in, 1 out]
                n131 = call "Display Message to User8"("error in (no error)"=w325) -> ()  [unwired: 9 in, 2 out]
              }
              frame True {
                n132 = case shown="真" w327 {
                  frame False {
                    n133 = call "setDO.vi"("channel"=7, "on/off"=FALSE) -> ()  [unwired: 9 in, 1 out]
                  }
                  frame True {
                    n134 = property on="Y满" class="Bool (严格)"() -> ("Value"=w331:bool)  [unwired: 2 in, 2 out]
                    n135 = Not(x=w331) -> (.not. x?=w330:bool)
                    n136 = case shown="真" w330 {
                      frame False {
                        n137 = call "setDO.vi"("channel"=7, "on/off"=TRUE) -> ()  [unwired: 9 in, 1 out]
                      }
                      frame True {
                        n138 = call "Display Message to User"() -> ()  [unwired: 10 in, 2 out]
                      }
                    }
                  }
                }
              }
            }
          }
          event "MCPHV-Set": Value Change {
            n139 = event-data() -> ("NewVal"=w335:dbl)  [unwired: 1 in, 5 out]
            n140 = Divide(x=w335, y=2000.0) -> (x/y=w338:dbl)
            n141 = Multiply(x=w338, y=10.0) -> (x*y=w336:dbl)
            n142 = call "setAO.vi"("value"=w336, "channel"=0) -> ()  [unwired: 9 in, 1 out]
          }
          event "Tar.HV-Set": Value Change {
            n143 = event-data() -> ("NewVal"=w347:dbl)  [unwired: 1 in, 5 out]
            n144 = Divide(x=w347, y=20000.0) -> (x/y=w344:dbl)
            n145 = Multiply(x=w344, y=10.0) -> (x*y=w342:dbl)
            n146 = call "setAO.vi"("value"=w342, "channel"=1) -> ()  [unwired: 9 in, 1 out]
          }
          event "Pul.HV-Set": Value Change {
            n147 = event-data() -> ("NewVal"=w354:dbl)  [unwired: 1 in, 5 out]
            n148 = Divide(x=w354, y=2000.0) -> (x/y=w351:dbl)
            n149 = Multiply(x=w351, y=10.0) -> (x*y=w349:dbl)
            n150 = call "setAO.vi"("value"=w349, "channel"=2) -> ()  [unwired: 9 in, 1 out]
          }
          event "LensHV-Set": Value Change {
            n151 = event-data() -> ("NewVal"=w361:dbl)  [unwired: 1 in, 5 out]
            n152 = Divide(x=w361, y=10000.0) -> (x/y=w358:dbl)
            n153 = Multiply(x=w358, y=10.0) -> (x*y=w357:dbl)
            n154 = call "setAO.vi"("value"=w357, "channel"=3) -> ()  [unwired: 9 in, 1 out]
          }
          event "Image": Mouse Down {
            n155 = event-data() -> ("Coords"=w362:T11)  [unwired: 1 in, 7 out]
            n156 = property on="移动" class="Bool (严格)"() -> ("Value"=w363:bool)  [unwired: 2 in, 2 out]
            n157 = case shown="假" w363 {
              tunnel: w362 -> [w374 _]
              frame False {
                w371 = -0.005 ("x")
                n158 = Unbundle(w374) -> ("Horizontal"=w373:i32, "Vertical"=w372:i32)
                n159 = property on="X当前" class="DigNum (严格)"() -> ("Value"=w370:dbl)  [unwired: 2 in, 2 out]
                n160 = property on="Y当前" class="DigNum (严格)"() -> ("Value"=w366:dbl)  [unwired: 2 in, 2 out]
                n161 = Subtract(x=w373, y=252.0) -> (x-y=w376:dbl)
                n162 = Subtract(x=w372, y=191.0) -> (x-y=w375:dbl)
                n163 = Multiply(x=w371, y=w376) -> (x*y=w369:dbl)
                n164 = Multiply(x=w371, y=w375) -> (x*y=w367:dbl)
                n165 = Add(x=w370, y=w369) -> (x+y=w368:dbl)
                n166 = Add(x=w367, y=w366) -> (x+y=w365:dbl)
                n167 = call "goto.vi"("Y(mm)"=w365, "X(mm)"=w368) -> ()  [unwired: 9 in, 1 out]
              }
              frame True {
              }
            }
          }
          event "测试记录": Shortcut Menu Selection (User) {
            n168 = event-data() -> ("ItemTag"=w381:string)  [unwired: 1 in, 7 out]
            n169 = case shown="\"鉴定\"" w381 {
              tunnel: w380 -> [w382 w389 w396 w401]
              tunnel: [w382 w389 w396 w397] -> w379
              frame "假", Default {
              }
              frame "鉴定" {
                n170 = property on="selected row" class="DigNum (严格)"() -> ("Value"=w385:i32)  [unwired: 2 in, 2 out]
                n171 = Index Array(array=w389, index=w385) -> (element=w395:T12)
                n172 = Unbundle By Name(w395) -> ("x"=w394:dbl[], "y"=w390:dbl[])
                n173 = call-poly <userlib>:"CaLabPut.vi"("Values"=w394, "PV Names"="MS:X") -> ("Error out"=w392:errorcluster)  [unwired: 6 in, 3 out]
                n174 = call-poly <userlib>:"CaLabPut.vi"("Error in (no error)"=w392, "Values"=w390, "PV Names"="MS:Y") -> ("Error out"=w388:errorcluster)  [unwired: 5 in, 3 out]
                n175 = call-poly <userlib>:"CaLabPut.vi"("Error in (no error)"=w388, "Value"=w385, "PV Name"="MS:NUM") -> ("Error out"=w387:errorcluster)  [unwired: 5 in, 3 out]
                n176 = call-poly <userlib>:"CaLabPut.vi"("Error in (no error)"=w387, "Value"=1, "PV Name"="MS:START") -> ()  [unwired: 5 in, 4 out]
              }
              frame "参数" {
              }
              frame "删除" {
                n177 = property on="selected row" class="DigNum (严格)"() -> ("Value"=w400:i32)  [unwired: 2 in, 2 out]
                n178 = Delete From Array "Delete From Array"(array=w401, index=w400) -> (array with subset deleted=w397:T5)  [unwired: 1 in, 1 out]
                n179 = for {
                  tunnel: w397 -> [w409] mode=indexing
                  shift-right: [w402] -> w398
                  shift-left: string[][] [] ("Item Names") -> [w404]
                  i -> [w405]
                  n180 = Unbundle By Name(w409) -> ("NO"=w408:string, "tag1"=w407:string, "tag2"=w406:string)
                  n181 = Build Array(w408, w407, w406) -> (w403:string[])
                  n182 = Insert Into Array "Insert Into Array"(array=w404, index (row)=w405, new element=w403) -> (w402:string[][])  [unwired: 1 in]
                }
                n183 = property on="测试记录" class="MCListbox (严格)"("ItemNames"=w398) -> ()  [unwired: 2 in, 2 out]
              }
            }
          }
          event "测试记录": Mouse Down {
            n184 = event-data() -> ("Coords"=w415:T11)  [unwired: 1 in, 7 out]
            n185 = invoke on="测试记录" class="MCListbox (严格)" method="Point To Row Column"("Point"=w415) -> ("CellPosition"=w414:T13)  [unwired: 6 in, 6 out]
            n186 = Unbundle By Name(w414) -> ("Row"=w411:i32)
            n187 = Array Size(array=w410) -> (size(s)=w413:i32)
            n188 = Greater Or Equal?(x=w413, y=w411) -> (x >= y?=w412:bool)
            n189 = case shown="真" w412 {
              tunnel: w411 -> [_ w442]
              tunnel: w410 -> [_ w443]
              frame False {
              }
              frame True {
                n190 = property on="selected row" class="DigNum (严格)"("Value"=w442) -> ()  [unwired: 2 in, 2 out]
                n191 = Index Array(array=w443, index=w442) -> (element=w441:T12)
                n192 = Unbundle By Name(w441) -> ("ID1:TAG1"=w424:string, "ID1:TAG2"=w438:string, "ID1:NAME"=w437:string, "ID1:SCORE"=w428:string, "ID2:TAG1"=w422:string, "ID2:TAG2"=w435:string, "ID2:NAME"=w434:string, "ID2:SCORE"=w427:string, "ID3:TAG1"=w420:string, "ID3:TAG2"=w419:string, "ID3:NAME"=w418:string, "ID3:SCORE"=w417:string)
                n193 = Build Array("1" ("element"), w424, w438, w437, w428) -> (w436:string[])
                n194 = Build Array("2" ("element"), w422, w435, w434, w427) -> (w431:string[])
                n195 = Build Array("3" ("element"), w420, w419, w418, w417) -> (w426:string[])
                n196 = Insert Into Array(array=string[][] [] ("项名"), index (row)=0 ("索引 (行)"), new element=w436) -> (w433:string[][])  [unwired: 1 in]
                n197 = Insert Into Array(array=w433, index (row)=1 ("索引 (行)"), new element=w431) -> (w430:string[][])  [unwired: 1 in]
                n198 = Insert Into Array(array=w430, index (row)=2 ("索引 (行)"), new element=w426) -> (w425:string[][])  [unwired: 1 in]
                n199 = property on="Identification Results (单靶鉴定结果)" class="MCListbox (严格)"("ItemNames"=w425) -> ()  [unwired: 2 in, 2 out]
              }
            }
          }
          event "Identification Results (单靶鉴定结果)": Mouse Down {
            n200 = event-data() -> ("Coords"=w449:T11)  [unwired: 1 in, 7 out]
            n201 = invoke on="Identification Results (单靶鉴定结果)" class="MCListbox (严格)" method="Point To Row Column"("Point"=w449) -> ("CellPosition"=w448:T13)  [unwired: 6 in, 6 out]
            n202 = Unbundle By Name(w448) -> ("Row"=w444:i32)
            n203 = Less Or Equal?(x=w444, y=2) -> (x <= y?=w446:bool)
            n204 = case shown="真" w446 {
              tunnel: w445 -> [_ w456]
              tunnel: w444 -> [_ w450]
              frame False {
              }
              frame True {
                n205 = property on="selected row" class="DigNum (严格)"() -> ("Value"=w455:i32)  [unwired: 2 in, 2 out]
                n206 = Index Array(array=w456, index=w455) -> (element=w454:T12)
                n207 = case shown="2" w450 {
                  tunnel: w454 -> [w462 w474 w483]
                  tunnel: [w461 w470 w479] -> w453
                  tunnel: [w460 w469 w478] -> w451
                  frame 0, Default {
                    n208 = Unbundle By Name(w462) -> ("x"=w464:dbl[], "y"=w463:dbl[], "ID1:REF:X"=w465:dbl[], "ID1:REF:Y"=w459:dbl[])
                    n209 = Multiply(x=w459, y=-1.0) -> (x*y=w457:dbl[])
                    n210 = Bundle("x"=w464, "y"=w463) -> (w461:cluster{"x":dbl[], "y":dbl[]})  [unwired: 1 in]
                    n211 = Bundle("ID1:REF:X"=w465, w457) -> (w460:cluster{"ID1:REF:X":dbl[], dbl[]})  [unwired: 1 in]
                  }
                  frame 1 {
                    n212 = Unbundle By Name(w474) -> ("x"=w472:dbl[], "y"=w471:dbl[], "ID2:REF:X"=w473:dbl[], "ID2:REF:Y"=w468:dbl[])
                    n213 = Multiply(x=w468, y=-1.0) -> (x*y=w466:dbl[])
                    n214 = Bundle("x"=w472, "y"=w471) -> (w470:cluster{"x":dbl[], "y":dbl[]})  [unwired: 1 in]
                    n215 = Bundle("ID2:REF:X"=w473, w466) -> (w469:cluster{"ID2:REF:X":dbl[], dbl[]})  [unwired: 1 in]
                  }
                  frame 2 {
                    n216 = Unbundle By Name(w483) -> ("x"=w481:dbl[], "y"=w480:dbl[], "ID3:REF:X"=w482:dbl[], "ID3:REF:Y"=w477:dbl[])
                    n217 = Multiply(x=w477, y=-1.0) -> (x*y=w475:dbl[])
                    n218 = Bundle("x"=w481, "y"=w480) -> (w479:cluster{"x":dbl[], "y":dbl[]})  [unwired: 1 in]
                    n219 = Bundle("ID3:REF:X"=w482, w475) -> (w478:cluster{"ID3:REF:X":dbl[], dbl[]})  [unwired: 1 in]
                  }
                }
                n220 = Build Array(w453, w451) -> (→"Identify Spcetrum":cluster{"ID3:REF:X":dbl[], "y":dbl[]}[])
              }
            }
          }
          event "Plat_To_Zero": Value Change {
            n221 = event-data() -> ("NewVal"=w485:bool)  [unwired: 1 in, 5 out]
            n222 = case shown="假" w485 {
              frame False {
              }
              frame True {
                (unwired) TRUE ("plat zeroed")
                n223 = call "plate_cal.vi"() -> ()  [unwired: 11 in, 1 out]
              }
            }
          }
          event "GO": Value Change {
            n224 = event-data() -> ("NewVal"=w488:bool)  [unwired: 1 in, 5 out]
            n225 = property on="移动" class="Bool (严格)"() -> ("Value"=w490:bool)  [unwired: 2 in, 2 out]
            n226 = Not(x=w490) -> (.not. x?=w489:bool)
            n227 = And(x=w489, y=w488) -> (x .and. y?=w487:bool)
            n228 = case shown="真" w487 {
              frame False {
              }
              frame True {
                n229 = property on="X" class="DigNum (严格)"() -> ("Value"=w492:dbl)  [unwired: 2 in, 2 out]
                n230 = property on="Y" class="DigNum (严格)"() -> ("Value"=w491:dbl)  [unwired: 2 in, 2 out]
                n231 = call "goto.vi"("Y(mm)"=w491, "X(mm)"=w492) -> ()  [unwired: 9 in, 1 out]
              }
            }
          }
          event "chamber in": Value Change {
            n232 = event-data() -> ("NewVal"=w495:bool)  [unwired: 1 in, 5 out]
            n233 = property on="HVEnable" class="Bool (严格)"() -> ("Value"=w500:bool)  [unwired: 2 in, 2 out]
            n234 = property on="Y满" class="Bool (严格)"() -> ("Value"=w496:bool)  [unwired: 2 in, 2 out]
            n235 = property on="移动" class="Bool (严格)"() -> ("Value"=w499:bool)  [unwired: 2 in, 2 out]
            n236 = Not(x=w500) -> (.not. x?=w497:bool)
            n237 = Not(x=w499) -> (.not. x?=w498:bool)
            n238 = Compound Arithmetic op=AND(w497, w496, w498, w495) -> (w494:bool)
            n239 = case shown="真" w494 {
              frame False {
              }
              frame True {
                n240 = flat-sequence {
                  tunnel: [w505] -> w501
                  tunnel: w501 -> [w515]
                  frame #0 {
                    n241 = call "样品标识与备注"() -> ("备注"=w502:string, "样品名称"=w503:string)  [unwired: 16 in, 2 out]
                    n242 = property on="sampleID" class="Str"("Value"=w503) -> ()  [unwired: 2 in, 2 out]
                    n243 = property on="commet" class="Str"("Value"=w502) -> ()  [unwired: 2 in, 2 out]
                  }
                  frame #1 {
                    w506 = FALSE ("on/off")
                    # "关样仓/大气"
                    n244 = Wait (ms)(milliseconds to wait=1500) -> ()  [unwired: 1 out]
                    n245 = call "setDO.vi"("channel"=6, "on/off"=w506) -> ("错误输出"=w504:errorcluster)  [unwired: 9 in]
                    n246 = property on="Samp_Atmos" class="Bool (严格)"(error in=w504, "Value"=w506) -> (error out=w505:errorcluster)  [unwired: 1 in, 1 out]
                  }
                  frame #2 {
                    # "开前泵/样仓"
                    n247 = call "setDO.vi"("错误输入（无错误）"=w515, "channel"=7, "on/off"=TRUE) -> ("错误输出"=w514:errorcluster)  [unwired: 8 in]
                    n248 = flat-sequence {
                      tunnel: w514 -> [w525]
                      tunnel: [w525] -> w510
                      frame #0 {
                        n249 = Wait (ms)(milliseconds to wait=10000) -> ()  [unwired: 1 out]
                      }
                    }
                    n250 = property on="Lvaccum" class="DigNum (严格)"(error in=w510) -> (error out=w509:errorcluster, "Value"=w513:dbl)  [unwired: 1 in, 1 out]
                    n251 = Less?(x=w513, y=10) -> (x < y?=w511:bool)
                    n252 = case shown="假" w511 {
                      tunnel: w509 -> [w519 w521]
                      frame False {
                        (unwired) 7
                        n253 = call "setDO.vi"("错误输入（无错误）"=w519, "on/off"=FALSE) -> ("错误输出"=w518:errorcluster)  [unwired: 9 in]
                        n254 = call "Display Message to User4"("error in (no error)"=w518) -> ()  [unwired: 9 in, 2 out]
                      }
                      frame True {
                        n255 = flat-sequence {
                          tunnel: w521 -> [w522]
                          frame #0 {
                            n256 = call "setDO.vi"("错误输入（无错误）"=w522, "channel"=7, "on/off"=FALSE) -> ()  [unwired: 8 in, 1 out]
                          }
                          frame #1 {
                            n257 = call "chamber_in.vi"() -> ()  [unwired: 12 in]
                          }
                        }
                      }
                    }
                  }
                }
              }
            }
          }
          event "chamber out": Value Change {
            n258 = event-data() -> ("NewVal"=w527:bool)  [unwired: 1 in, 5 out]
            n259 = case shown="真" w527 {
              frame False {
              }
              frame True {
                n260 = property on="移动" class="Bool (严格)"() -> ("Value"=w533:bool)  [unwired: 2 in, 2 out]
                n261 = property on="Y满" class="Bool (严格)"() -> ("Value"=w534:bool)  [unwired: 2 in, 2 out]
                n262 = property on="HVEnable" class="Bool (严格)"() -> ("Value"=w535:bool)  [unwired: 2 in, 2 out]
                n263 = Not "非"(x=w533) -> (.not. x?=w531:bool)
                n264 = Not "非"(x=w534) -> (.not. x?=w532:bool)
                n265 = Not "非"(x=w535) -> (.not. x?=w529:bool)
                n266 = Compound Arithmetic op=AND "复合运算"(w529, w532, w531) -> (w530:bool)
                n267 = case shown="真" w530 {
                  frame False {
                    n268 = call "Display Message to User3"() -> ()  [unwired: 10 in, 2 out]
                  }
                  frame True {
                    n269 = flat-sequence {
                      tunnel: [w539] -> w537
                      tunnel: w537 -> [w545]
                      tunnel: [w546] -> w536
                      tunnel: w536 -> [w557]
                      frame #0 {
                        n270 = call "chamber_out.vi"() -> ()  [unwired: 12 in]
                      }
                      frame #1 {
                        w540 = FALSE ("on/off")
                        # "关前泵/样仓"
                        n271 = Wait (ms)(milliseconds to wait=1500) -> ()  [unwired: 1 out]
                        n272 = call "setDO.vi"("channel"=7, "on/off"=w540) -> ("错误输出"=w538:errorcluster)  [unwired: 9 in]
                        n273 = property on="Fore_Samp" class="Bool (严格)"(error in=w538, "Value"=w540) -> (error out=w539:errorcluster)  [unwired: 1 in, 1 out]
                      }
                      frame #2 {
                        # "开样仓/大气"
                        n274 = call "Time Delay4"("error in (no error)"=w545, "Delay Time (s)"=3.0) -> ("error out"=w544:errorcluster)  [unwired: 9 in]
                        n275 = property on="Y满" class="Bool (严格)"(error in=w544) -> (error out=w547:errorcluster, "Value"=w548:bool)  [unwired: 1 in, 1 out]
                        n276 = case shown="真" w548 {
                          tunnel: w547 -> [w550 w552]
                          tunnel: [w549 w551] -> w546
                          frame False {
                            n277 = call "Display Message to User2"("error in (no error)"=w550) -> ("error out"=w549:errorcluster)  [unwired: 9 in, 1 out]
                          }
                          frame True {
                            n278 = call "setDO.vi"("错误输入（无错误）"=w552, "channel"=6, "on/off"=TRUE) -> ("错误输出"=w551:errorcluster)  [unwired: 8 in]
                          }
                        }
                      }
                      frame #3 {
                        n279 = call "Time Delay5"("error in (no error)"=w557, "Delay Time (s)"=3.0) -> ("error out"=w556:errorcluster)  [unwired: 9 in]
                        n280 = call "setDO.vi"("错误输入（无错误）"=w556, "channel"=6, "on/off"=FALSE) -> ()  [unwired: 8 in, 1 out]
                      }
                    }
                  }
                }
              }
            }
          }
          event "标准样品": Value Change {
            n281 = event-data() -> ("NewVal"=w560:u16)  [unwired: 1 in, 5 out]
            n282 = local read "std sample"() -> (w564:T2)
            n283 = control-ref of="定标参数"() -> (w565:refnum<vi>)
            n284 = property on="config" class="TypRef (严格)"() -> ("Value"=w563:T1)  [unwired: 2 in, 2 out]
            n285 = call-poly <vilib>:"Write Key.vi"("section"="cal", "value"=w560, "key"="type", "refnum"=w563) -> ()  [unwired: 5 in, 3 out]
            n286 = call "writetable.vi"("std sample"=w564, "type"=w560, "reference"=w565) -> ()  [unwired: 9 in]
          }
          event "peak cal": Value Change {
            n287 = event-data() -> ("NewVal"=w567:bool)  [unwired: 1 in, 5 out]
            n288 = case shown="真" w567 {
              frame False {
              }
              frame True {
                w579 = "cal" ("section")
                n289 = property on="定标参数" class="MCListbox (严格)"() -> ("ItemNames"=w598:string[][])  [unwired: 2 in, 2 out]
                n290 = Index Array(array=w598, index (col)=1 ("disabled index (col)")) -> (element=w599:string[])  [unwired: 1 in]
                n291 = Index Array(array=w598, index (col)=3 ("disabled index (col)")) -> (element=w596:string[])  [unwired: 1 in]
                n292 = property on="config" class="TypRef (严格)"() -> ("Value"=w573:T1)  [unwired: 2 in, 2 out]
                n293 = Fract/Exp String To Number(string=w596) -> (number=w574:dbl[])  [unwired: 3 in, 1 out]
                n294 = Fract/Exp String To Number(string=w599) -> (number=w589:dbl[])  [unwired: 3 in, 1 out]
                n295 = call "write_peak_data.vi"("array in"=w574, "refnum"=w573) -> ("error out"=w571:errorcluster, "refnum out"=w572:T1)  [unwired: 8 in]
                n296 = call <vilib>:"General Polynomial Fit.vi"("Y"=w589, "polynomial order"=2, "X"=w574) -> ("Polynomial Coefficients"=w592:dbl[])  [unwired: 9 in, 3 out]
                n297 = Index Array(array=w592, index=2) -> (element=w582:dbl)
                "a:" <- w582
                n298 = Index Array(array=w592, index=1) -> (element=w577:dbl)
                "b:" <- w577
                n299 = Index Array(array=w592, index=0) -> (element=w576:dbl)
                "c:" <- w576
                n300 = global write "cal_p.vi" "a"(w582) -> ()
                n301 = global write "cal_p.vi" "b"(w577) -> ()
                n302 = for {
                  tunnel: w574 -> [w613] mode=indexing
                  tunnel: [w617] -> w590 mode=indexing
                  tunnel: w576 -> [w614]
                  tunnel: w577 -> [w615]
                  tunnel: w582 -> [w616]
                  n303 = formula code="m=a*x*x+b*x+c;"("a"=w616, "b"=w615, "c"=w614, "x"=w613) -> ("m"=w617:dbl)
                }
                n304 = global write "cal_p.vi" "c"(w576) -> ()
                n305 = call-poly <vilib>:"Write Key.vi"("section"=w579, "error in (no error)"=w571, "value"=w582, "key"="a", "refnum"=w572) -> ("error out"=w570:errorcluster, "refnum out"=w581:T1)  [unwired: 4 in, 1 out]
                n306 = for {
                  tunnel: w590 -> [w611] mode=indexing
                  tunnel: w589 -> [w612] mode=indexing
                  tunnel: [w610] -> w584 mode=indexing
                  n307 = formula code="delta=100*(m-m0)/m0;"("m0"=w612, "m"=w611) -> ("delta"=w610:dbl)
                }
                n308 = call-poly <vilib>:"Write Key.vi"("section"=w579, "error in (no error)"=w570, "value"=w577, "key"="b", "refnum"=w581) -> ("error out"=w569:errorcluster, "refnum out"=w575:T1)  [unwired: 4 in, 1 out]
                n309 = call-poly <vilib>:"Write Key.vi"("section"=w579, "error in (no error)"=w569, "value"=w576, "key"="c", "refnum"=w575) -> ()  [unwired: 4 in, 3 out]
                n310 = control-ref of="定标参数"() -> (w588:refnum<vi>)
                n311 = property on="Property Node" class="MCListbox (严格)"(reference=w588) -> (reference out=w587:refnum<vi>, "ItemNames"=w586:string[][])  [unwired: 1 in, 1 out]
                n312 = for {
                  shift-right: [w606] -> w585
                  shift-left: w586 -> [w609]
                  tunnel: w584 -> [w607] mode=indexing
                  i -> [w608]
                  n313 = Number To Fractional String(number=w607, precision (6)=i16 2) -> (F-format string=w604:string)  [unwired: 2 in]
                  n314 = Concatenate Strings(w604, "%" ("string")) -> (w602:string)
                  n315 = Replace Array Subset(array=w609, new element=w602, index (row)=w608, index (col)=4 ("disabled index (col)")) -> (w606:string[][])
                }
                n316 = property on="Property Node" class="MCListbox (严格)"(reference=w587, "ItemNames"=w585) -> ()  [unwired: 1 in, 2 out]
              }
            }
          }
          event "A1-Position": Value Change {
            n317 = event-data() -> ("NewVal"=w619:bool)  [unwired: 1 in, 5 out]
            n318 = case shown="真" w619 {
              frame False {
              }
              frame True {
                n319 = property on="X当前" class="DigNum (严格)"() -> ("Value"=→"A1-position-X":dbl)  [unwired: 2 in, 2 out]
                n320 = property on="Y当前" class="DigNum (严格)"() -> ("Value"=→"A1-position-Y":dbl)  [unwired: 2 in, 2 out]
              }
            }
          }
          event "A1": Value Change {
            n321 = event-data() -> ("NewVal"=w625:bool)  [unwired: 1 in, 5 out]
            n322 = property on="移动" class="Bool (严格)"() -> ("Value"=w627:bool)  [unwired: 2 in, 2 out]
            n323 = Not(x=w627) -> (.not. x?=w626:bool)
            n324 = And(x=w626, y=w625) -> (x .and. y?=w624:bool)
            n325 = case shown="真" w624 {
              frame False {
              }
              frame True {
                n326 = property on="A1-position-X" class="DigNum (严格)"() -> (error out=w632:errorcluster, "Value"=w630:dbl)  [unwired: 2 in, 1 out]
                n327 = property on="A1-position-Y" class="DigNum (严格)"(error in=w632) -> (error out=w631:errorcluster, "Value"=w629:dbl)  [unwired: 1 in, 1 out]
                n328 = vi-ref "goto.vi"() -> (w636:refnum<vi>)
                n329 = property class="VI"(reference=w636, error in=w631) -> ("Name"=w635:string)  [unwired: 2 out]
                n330 = Open VI Reference(type specifier VI Refnum (for type only)=refnum<vi> refnum, vi path=w635, options=128) -> (vi reference=w633:refnum<vi>)  [unwired: 3 in, 1 out]
                n331 = call-by-ref "Start Asynchronous Call"(reference=w633, "Y(mm)"=w629, "X(mm)"=w630) -> ()  [unwired: 10 in, 3 out]
              }
            }
            n332 = property on="currentNO" class="Str"("Value"="A1") -> ()  [unwired: 2 in, 2 out]
          }
          event "A2": Value Change {
            n333 = event-data() -> ("NewVal"=w640:bool)  [unwired: 1 in, 5 out]
            n334 = property on="移动" class="Bool (严格)"() -> ("Value"=w643:bool)  [unwired: 2 in, 2 out]
            n335 = Not(x=w643) -> (.not. x?=w642:bool)
            n336 = And(x=w642, y=w640) -> (x .and. y?=w641:bool)
            n337 = case shown="真" w641 {
              frame False {
              }
              frame True {
                n338 = property on="A1-position-X" class="DigNum (严格)"() -> (error out=w647:errorcluster, "Value"=w654:dbl)  [unwired: 2 in, 1 out]
                n339 = property on="A1-position-Y" class="DigNum (严格)"(error in=w647) -> (error out=w646:errorcluster, "Value"=w644:dbl)  [unwired: 1 in, 1 out]
                n340 = Subtract(x=w654, y=4.5) -> (x-y=w645:dbl)
                n341 = vi-ref "goto.vi"() -> (w652:refnum<vi>)
                n342 = property class="VI"(reference=w652, error in=w646) -> ("Name"=w651:string)  [unwired: 2 out]
                n343 = Open VI Reference(type specifier VI Refnum (for type only)=refnum<vi> refnum, vi path=w651, options=128) -> (vi reference=w649:refnum<vi>)  [unwired: 3 in, 1 out]
                n344 = call-by-ref "Start Asynchronous Call"(reference=w649, "Y(mm)"=w644, "X(mm)"=w645) -> ()  [unwired: 10 in, 3 out]
              }
            }
            n345 = control-ref of="currentNO"() -> (w637:refnum<vi>)
            n346 = property on="属性节点" class="Str"(reference=w637, "Value"="A2") -> ()  [unwired: 1 in, 2 out]
          }
          event "A3": Value Change {
            n347 = event-data() -> ("NewVal"=w658:bool)  [unwired: 1 in, 5 out]
            n348 = property on="移动" class="Bool (严格)"() -> ("Value"=w661:bool)  [unwired: 2 in, 2 out]
            n349 = Not(x=w661) -> (.not. x?=w660:bool)
            n350 = And(x=w660, y=w658) -> (x .and. y?=w659:bool)
            n351 = case shown="真" w659 {
              frame False {
              }
              frame True {
                n352 = property on="A1-position-X" class="DigNum (严格)"() -> (error out=w665:errorcluster, "Value"=w672:dbl)  [unwired: 2 in, 1 out]
                n353 = property on="A1-position-Y" class="DigNum (严格)"(error in=w665) -> (error out=w664:errorcluster, "Value"=w662:dbl)  [unwired: 1 in, 1 out]
                n354 = Subtract(x=w672, y=9.0) -> (x-y=w663:dbl)
                n355 = vi-ref "goto.vi"() -> (w670:refnum<vi>)
                n356 = property class="VI"(reference=w670, error in=w664) -> ("Name"=w669:string)  [unwired: 2 out]
                n357 = Open VI Reference(type specifier VI Refnum (for type only)=refnum<vi> refnum, vi path=w669, options=128) -> (vi reference=w667:refnum<vi>)  [unwired: 3 in, 1 out]
                n358 = call-by-ref "Start Asynchronous Call"(reference=w667, "Y(mm)"=w662, "X(mm)"=w663) -> ()  [unwired: 10 in, 3 out]
              }
            }
            n359 = control-ref of="currentNO"() -> (w655:refnum<vi>)
            n360 = property on="属性节点" class="Str"(reference=w655, "Value"="A3") -> ()  [unwired: 1 in, 2 out]
          }
          event "A4": Value Change {
            n361 = event-data() -> ("NewVal"=w675:bool)  [unwired: 1 in, 5 out]
            n362 = property on="移动" class="Bool (严格)"() -> ("Value"=w678:bool)  [unwired: 2 in, 2 out]
            n363 = Not(x=w678) -> (.not. x?=w677:bool)
            n364 = And(x=w677, y=w675) -> (x .and. y?=w676:bool)
            n365 = case shown="真" w676 {
              frame False {
              }
              frame True {
                n366 = property on="A1-position-X" class="DigNum (严格)"() -> (error out=w682:errorcluster, "Value"=w689:dbl)  [unwired: 2 in, 1 out]
                n367 = property on="A1-position-Y" class="DigNum (严格)"(error in=w682) -> (error out=w681:errorcluster, "Value"=w679:dbl)  [unwired: 1 in, 1 out]
                n368 = Subtract(x=w689, y=13.5) -> (x-y=w680:dbl)
                n369 = vi-ref "goto.vi"() -> (w687:refnum<vi>)
                n370 = property class="VI"(reference=w687, error in=w681) -> ("Name"=w686:string)  [unwired: 2 out]
                n371 = Open VI Reference(type specifier VI Refnum (for type only)=refnum<vi> refnum, vi path=w686, options=128) -> (vi reference=w684:refnum<vi>)  [unwired: 3 in, 1 out]
                n372 = call-by-ref "Start Asynchronous Call"(reference=w684, "Y(mm)"=w679, "X(mm)"=w680) -> ()  [unwired: 10 in, 3 out]
              }
            }
            n373 = property on="currentNO" class="Str"("Value"="A4") -> ()  [unwired: 2 in, 2 out]
          }
          event "A5": Value Change {
            n374 = event-data() -> ("NewVal"=w692:bool)  [unwired: 1 in, 5 out]
            n375 = property on="移动" class="Bool (严格)"() -> ("Value"=w695:bool)  [unwired: 2 in, 2 out]
            n376 = Not(x=w695) -> (.not. x?=w694:bool)
            n377 = And(x=w694, y=w692) -> (x .and. y?=w693:bool)
            n378 = case shown="真" w693 {
              frame False {
              }
              frame True {
                n379 = property on="A1-position-X" class="DigNum (严格)"() -> (error out=w699:errorcluster, "Value"=w706:dbl)  [unwired: 2 in, 1 out]
                n380 = property on="A1-position-Y" class="DigNum (严格)"(error in=w699) -> (error out=w698:errorcluster, "Value"=w696:dbl)  [unwired: 1 in, 1 out]
                n381 = Subtract(x=w706, y=18) -> (x-y=w697:dbl)
                n382 = vi-ref "goto.vi"() -> (w704:refnum<vi>)
                n383 = property class="VI"(reference=w704, error in=w698) -> ("Name"=w703:string)  [unwired: 2 out]
                n384 = Open VI Reference(type specifier VI Refnum (for type only)=refnum<vi> refnum, vi path=w703, options=128) -> (vi reference=w701:refnum<vi>)  [unwired: 3 in, 1 out]
                n385 = call-by-ref "Start Asynchronous Call"(reference=w701, "Y(mm)"=w696, "X(mm)"=w697) -> ()  [unwired: 10 in, 3 out]
              }
            }
            n386 = property on="currentNO" class="Str"("Value"="A5") -> ()  [unwired: 2 in, 2 out]
          }
          event "A6": Value Change {
            n387 = event-data() -> ("NewVal"=w709:bool)  [unwired: 1 in, 5 out]
            n388 = property on="移动" class="Bool (严格)"() -> ("Value"=w712:bool)  [unwired: 2 in, 2 out]
            n389 = Not(x=w712) -> (.not. x?=w711:bool)
            n390 = And(x=w711, y=w709) -> (x .and. y?=w710:bool)
            n391 = case shown="真" w710 {
              frame False {
              }
              frame True {
                n392 = property on="A1-position-X" class="DigNum (严格)"() -> (error out=w716:errorcluster, "Value"=w723:dbl)  [unwired: 2 in, 1 out]
                n393 = property on="A1-position-Y" class="DigNum (严格)"(error in=w716) -> (error out=w715:errorcluster, "Value"=w713:dbl)  [unwired: 1 in, 1 out]
                n394 = Subtract(x=w723, y=22.5) -> (x-y=w714:dbl)
                n395 = vi-ref "goto.vi"() -> (w721:refnum<vi>)
                n396 = property class="VI"(reference=w721, error in=w715) -> ("Name"=w720:string)  [unwired: 2 out]
                n397 = Open VI Reference(type specifier VI Refnum (for type only)=refnum<vi> refnum, vi path=w720, options=128) -> (vi reference=w718:refnum<vi>)  [unwired: 3 in, 1 out]
                n398 = call-by-ref "Start Asynchronous Call"(reference=w718, "Y(mm)"=w713, "X(mm)"=w714) -> ()  [unwired: 10 in, 3 out]
              }
            }
            n399 = property on="currentNO" class="Str"("Value"="A6") -> ()  [unwired: 2 in, 2 out]
          }
          event "A7": Value Change {
            n400 = event-data() -> ("NewVal"=w726:bool)  [unwired: 1 in, 5 out]
            n401 = property on="移动" class="Bool (严格)"() -> ("Value"=w729:bool)  [unwired: 2 in, 2 out]
            n402 = Not(x=w729) -> (.not. x?=w728:bool)
            n403 = And(x=w728, y=w726) -> (x .and. y?=w727:bool)
            n404 = case shown="真" w727 {
              frame False {
              }
              frame True {
                n405 = property on="A1-position-X" class="DigNum (严格)"() -> (error out=w733:errorcluster, "Value"=w740:dbl)  [unwired: 2 in, 1 out]
                n406 = property on="A1-position-Y" class="DigNum (严格)"(error in=w733) -> (error out=w732:errorcluster, "Value"=w730:dbl)  [unwired: 1 in, 1 out]
                n407 = Subtract(x=w740, y=27) -> (x-y=w731:dbl)
                n408 = vi-ref "goto.vi"() -> (w738:refnum<vi>)
                n409 = property class="VI"(reference=w738, error in=w732) -> ("Name"=w737:string)  [unwired: 2 out]
                n410 = Open VI Reference(type specifier VI Refnum (for type only)=refnum<vi> refnum, vi path=w737, options=128) -> (vi reference=w735:refnum<vi>)  [unwired: 3 in, 1 out]
                n411 = call-by-ref "Start Asynchronous Call"(reference=w735, "Y(mm)"=w730, "X(mm)"=w731) -> ()  [unwired: 10 in, 3 out]
              }
            }
            n412 = property on="currentNO" class="Str"("Value"="A7") -> ()  [unwired: 2 in, 2 out]
          }
          event User Event {
            n413 = event-data() -> ("PV name"=w742:string, "value array (string)"=w741:string[])  [unwired: 1 in, 9 out]
            n414 = case shown="\"ID:STATUS\"" w742 {
              tunnel: w744 -> [w748 w754]
              tunnel: [w748 w757] -> w743
              tunnel: w741 -> [w747 _]
              frame "ID:INFO", Default {
                n415 = Index Array(array=w747, index=0) -> (element=→"idn status":string)
              }
              frame "ID:STATUS" {
                n416 = call "getIOCdata.vi"() -> ("输出簇"=w755:T12)  [unwired: 11 in]
                n417 = call-poly <userlib>:"CaLabGet.vi"("PV Name"="MS:NUM") -> ("1rst Value (number)"=w753:dbl)  [unwired: 8 in, 6 out]
                n418 = Index Array(array=w754, index=w753) -> (element=w752:T12)
                n419 = Unbundle By Name(w752) -> ("NO"=w751:string, "tag2"=w750:string)
                n420 = Bundle By Name(cluster=w755, "NO"=w751, "tag2"=w750) -> (w749:T12)
                n421 = Replace Array Subset "Replace Array Subset"(array=w754, new element=w749, index=w753) -> (w757:T5)
                n422 = for {
                  tunnel: w757 -> [w767] mode=indexing
                  shift-right: [w760] -> w756
                  shift-left: string[][] [] ("Item Names") -> [w762]
                  i -> [w763]
                  n423 = Unbundle By Name(w767) -> ("NO"=w766:string, "tag1"=w765:string, "tag2"=w764:string)
                  n424 = Build Array(w766, w765, w764) -> (w761:string[])
                  n425 = Insert Into Array "Insert Into Array"(array=w762, index (row)=w763, new element=w761) -> (w760:string[][])  [unwired: 1 in]
                }
                n426 = property on="测试记录" class="MCListbox (严格)"("ItemNames"=w756) -> ()  [unwired: 2 in, 2 out]
              }
            }
          }
          event "A8": Value Change {
            n427 = event-data() -> ("NewVal"=w770:bool)  [unwired: 1 in, 5 out]
            n428 = property on="移动" class="Bool (严格)"() -> ("Value"=w773:bool)  [unwired: 2 in, 2 out]
            n429 = Not(x=w773) -> (.not. x?=w772:bool)
            n430 = And(x=w772, y=w770) -> (x .and. y?=w771:bool)
            n431 = case shown="假" w771 {
              frame False {
              }
              frame True {
                n432 = property on="A1-position-X" class="DigNum (严格)"() -> (error out=w777:errorcluster, "Value"=w784:dbl)  [unwired: 2 in, 1 out]
                n433 = property on="A1-position-Y" class="DigNum (严格)"(error in=w777) -> (error out=w776:errorcluster, "Value"=w774:dbl)  [unwired: 1 in, 1 out]
                n434 = Subtract(x=w784, y=31.5) -> (x-y=w775:dbl)
                n435 = vi-ref "goto.vi"() -> (w782:refnum<vi>)
                n436 = property class="VI"(reference=w782, error in=w776) -> ("Name"=w781:string)  [unwired: 2 out]
                n437 = Open VI Reference(type specifier VI Refnum (for type only)=refnum<vi> refnum, vi path=w781, options=128) -> (vi reference=w779:refnum<vi>)  [unwired: 3 in, 1 out]
                n438 = call-by-ref "Start Asynchronous Call"(reference=w779, "Y(mm)"=w774, "X(mm)"=w775) -> ()  [unwired: 10 in, 3 out]
              }
            }
            n439 = property on="currentNO" class="Str"("Value"="A8") -> ()  [unwired: 2 in, 2 out]
          }
          event "A9": Value Change {
            n440 = event-data() -> ("NewVal"=w787:bool)  [unwired: 1 in, 5 out]
            n441 = property on="移动" class="Bool (严格)"() -> ("Value"=w790:bool)  [unwired: 2 in, 2 out]
            n442 = Not(x=w790) -> (.not. x?=w789:bool)
            n443 = And(x=w789, y=w787) -> (x .and. y?=w788:bool)
            n444 = case shown="真" w788 {
              frame False {
              }
              frame True {
                n445 = property on="A1-position-X" class="DigNum (严格)"() -> (error out=w794:errorcluster, "Value"=w801:dbl)  [unwired: 2 in, 1 out]
                n446 = property on="A1-position-Y" class="DigNum (严格)"(error in=w794) -> (error out=w793:errorcluster, "Value"=w791:dbl)  [unwired: 1 in, 1 out]
                n447 = Subtract(x=w801, y=36) -> (x-y=w792:dbl)
                n448 = vi-ref "goto.vi"() -> (w799:refnum<vi>)
                n449 = property class="VI"(reference=w799, error in=w793) -> ("Name"=w798:string)  [unwired: 2 out]
                n450 = Open VI Reference(type specifier VI Refnum (for type only)=refnum<vi> refnum, vi path=w798, options=128) -> (vi reference=w796:refnum<vi>)  [unwired: 3 in, 1 out]
                n451 = call-by-ref "Start Asynchronous Call"(reference=w796, "Y(mm)"=w791, "X(mm)"=w792) -> ()  [unwired: 10 in, 3 out]
              }
            }
            n452 = property on="currentNO" class="Str"("Value"="A9") -> ()  [unwired: 2 in, 2 out]
          }
          event "A10": Value Change {
            n453 = event-data() -> ("NewVal"=w804:bool)  [unwired: 1 in, 5 out]
            n454 = property on="移动" class="Bool (严格)"() -> ("Value"=w807:bool)  [unwired: 2 in, 2 out]
            n455 = Not(x=w807) -> (.not. x?=w806:bool)
            n456 = And(x=w806, y=w804) -> (x .and. y?=w805:bool)
            n457 = case shown="真" w805 {
              frame False {
              }
              frame True {
                n458 = property on="A1-position-X" class="DigNum (严格)"() -> (error out=w811:errorcluster, "Value"=w818:dbl)  [unwired: 2 in, 1 out]
                n459 = property on="A1-position-Y" class="DigNum (严格)"(error in=w811) -> (error out=w810:errorcluster, "Value"=w808:dbl)  [unwired: 1 in, 1 out]
                n460 = Subtract(x=w818, y=40.5) -> (x-y=w809:dbl)
                n461 = vi-ref "goto.vi"() -> (w816:refnum<vi>)
                n462 = property class="VI"(reference=w816, error in=w810) -> ("Name"=w815:string)  [unwired: 2 out]
                n463 = Open VI Reference(type specifier VI Refnum (for type only)=refnum<vi> refnum, vi path=w815, options=128) -> (vi reference=w813:refnum<vi>)  [unwired: 3 in, 1 out]
                n464 = call-by-ref "Start Asynchronous Call"(reference=w813, "Y(mm)"=w808, "X(mm)"=w809) -> ()  [unwired: 10 in, 3 out]
              }
            }
            n465 = property on="currentNO" class="Str"("Value"="A10") -> ()  [unwired: 2 in, 2 out]
          }
          event "A11": Value Change {
            n466 = event-data() -> ("NewVal"=w821:bool)  [unwired: 1 in, 5 out]
            n467 = property on="移动" class="Bool (严格)"() -> ("Value"=w824:bool)  [unwired: 2 in, 2 out]
            n468 = Not(x=w824) -> (.not. x?=w823:bool)
            n469 = And(x=w823, y=w821) -> (x .and. y?=w822:bool)
            n470 = case shown="真" w822 {
              frame False {
              }
              frame True {
                n471 = property on="A1-position-X" class="DigNum (严格)"() -> (error out=w828:errorcluster, "Value"=w835:dbl)  [unwired: 2 in, 1 out]
                n472 = property on="A1-position-Y" class="DigNum (严格)"(error in=w828) -> (error out=w827:errorcluster, "Value"=w825:dbl)  [unwired: 1 in, 1 out]
                n473 = Subtract(x=w835, y=45) -> (x-y=w826:dbl)
                n474 = vi-ref "goto.vi"() -> (w833:refnum<vi>)
                n475 = property class="VI"(reference=w833, error in=w827) -> ("Name"=w832:string)  [unwired: 2 out]
                n476 = Open VI Reference(type specifier VI Refnum (for type only)=refnum<vi> refnum, vi path=w832, options=128) -> (vi reference=w830:refnum<vi>)  [unwired: 3 in, 1 out]
                n477 = call-by-ref "Start Asynchronous Call"(reference=w830, "Y(mm)"=w825, "X(mm)"=w826) -> ()  [unwired: 10 in, 3 out]
              }
            }
            n478 = property on="currentNO" class="Str"("Value"="A11") -> ()  [unwired: 2 in, 2 out]
          }
          event "A12": Value Change {
            n479 = event-data() -> ("NewVal"=w838:bool)  [unwired: 1 in, 5 out]
            n480 = property on="移动" class="Bool (严格)"() -> ("Value"=w841:bool)  [unwired: 2 in, 2 out]
            n481 = Not(x=w841) -> (.not. x?=w840:bool)
            n482 = And(x=w840, y=w838) -> (x .and. y?=w839:bool)
            n483 = case shown="真" w839 {
              frame False {
              }
              frame True {
                n484 = property on="A1-position-X" class="DigNum (严格)"() -> (error out=w845:errorcluster, "Value"=w852:dbl)  [unwired: 2 in, 1 out]
                n485 = property on="A1-position-Y" class="DigNum (严格)"(error in=w845) -> (error out=w844:errorcluster, "Value"=w842:dbl)  [unwired: 1 in, 1 out]
                n486 = Subtract(x=w852, y=49.5) -> (x-y=w843:dbl)
                n487 = vi-ref "goto.vi"() -> (w850:refnum<vi>)
                n488 = property class="VI"(reference=w850, error in=w844) -> ("Name"=w849:string)  [unwired: 2 out]
                n489 = Open VI Reference(type specifier VI Refnum (for type only)=refnum<vi> refnum, vi path=w849, options=128) -> (vi reference=w847:refnum<vi>)  [unwired: 3 in, 1 out]
                n490 = call-by-ref "Start Asynchronous Call"(reference=w847, "Y(mm)"=w842, "X(mm)"=w843) -> ()  [unwired: 10 in, 3 out]
              }
            }
            n491 = property on="currentNO" class="Str"("Value"="A12") -> ()  [unwired: 2 in, 2 out]
          }
          event "B1": Value Change {
            n492 = event-data() -> ("NewVal"=w855:bool)  [unwired: 1 in, 5 out]
            n493 = property on="移动" class="Bool (严格)"() -> ("Value"=w858:bool)  [unwired: 2 in, 2 out]
            n494 = Not(x=w858) -> (.not. x?=w857:bool)
            n495 = And(x=w857, y=w855) -> (x .and. y?=w856:bool)
            n496 = case shown="真" w856 {
              frame False {
              }
              frame True {
                n497 = property on="A1-position-X" class="DigNum (严格)"() -> (error out=w864:errorcluster, "Value"=w871:dbl)  [unwired: 2 in, 1 out]
                n498 = property on="A1-position-Y" class="DigNum (严格)"(error in=w864) -> (error out=w863:errorcluster, "Value"=w860:dbl)  [unwired: 1 in, 1 out]
                n499 = Subtract(x=w860, y=4.5) -> (x-y=w859:dbl)
                n500 = Subtract(x=w871, y=0) -> (x-y=w862:dbl)
                n501 = vi-ref "goto.vi"() -> (w869:refnum<vi>)
                n502 = property class="VI"(reference=w869, error in=w863) -> ("Name"=w868:string)  [unwired: 2 out]
                n503 = Open VI Reference(type specifier VI Refnum (for type only)=refnum<vi> refnum, vi path=w868, options=128) -> (vi reference=w866:refnum<vi>)  [unwired: 3 in, 1 out]
                n504 = call-by-ref "Start Asynchronous Call"(reference=w866, "Y(mm)"=w859, "X(mm)"=w862) -> ()  [unwired: 10 in, 3 out]
              }
            }
            n505 = property on="currentNO" class="Str"("Value"="B1") -> ()  [unwired: 2 in, 2 out]
          }
          event "B2": Value Change {
            n506 = event-data() -> ("NewVal"=w874:bool)  [unwired: 1 in, 5 out]
            n507 = property on="移动" class="Bool (严格)"() -> ("Value"=w877:bool)  [unwired: 2 in, 2 out]
            n508 = Not(x=w877) -> (.not. x?=w876:bool)
            n509 = And(x=w876, y=w874) -> (x .and. y?=w875:bool)
            n510 = case shown="真" w875 {
              frame False {
              }
              frame True {
                n511 = property on="A1-position-X" class="DigNum (严格)"() -> (error out=w883:errorcluster, "Value"=w890:dbl)  [unwired: 2 in, 1 out]
                n512 = property on="A1-position-Y" class="DigNum (严格)"(error in=w883) -> (error out=w882:errorcluster, "Value"=w879:dbl)  [unwired: 1 in, 1 out]
                n513 = Subtract(x=w879, y=4.5) -> (x-y=w878:dbl)
                n514 = Subtract(x=w890, y=4.5) -> (x-y=w881:dbl)
                n515 = vi-ref "goto.vi"() -> (w888:refnum<vi>)
                n516 = property class="VI"(reference=w888, error in=w882) -> ("Name"=w887:string)  [unwired: 2 out]
                n517 = Open VI Reference(type specifier VI Refnum (for type only)=refnum<vi> refnum, vi path=w887, options=128) -> (vi reference=w885:refnum<vi>)  [unwired: 3 in, 1 out]
                n518 = call-by-ref "Start Asynchronous Call"(reference=w885, "Y(mm)"=w878, "X(mm)"=w881) -> ()  [unwired: 10 in, 3 out]
              }
            }
            n519 = property on="currentNO" class="Str"("Value"="B2") -> ()  [unwired: 2 in, 2 out]
          }
          event "B3": Value Change {
            n520 = event-data() -> ("NewVal"=w893:bool)  [unwired: 1 in, 5 out]
            n521 = property on="移动" class="Bool (严格)"() -> ("Value"=w896:bool)  [unwired: 2 in, 2 out]
            n522 = Not(x=w896) -> (.not. x?=w895:bool)
            n523 = And(x=w895, y=w893) -> (x .and. y?=w894:bool)
            n524 = case shown="真" w894 {
              frame False {
              }
              frame True {
                n525 = property on="A1-position-X" class="DigNum (严格)"() -> (error out=w902:errorcluster, "Value"=w909:dbl)  [unwired: 2 in, 1 out]
                n526 = property on="A1-position-Y" class="DigNum (严格)"(error in=w902) -> (error out=w901:errorcluster, "Value"=w898:dbl)  [unwired: 1 in, 1 out]
                n527 = Subtract(x=w898, y=4.5) -> (x-y=w897:dbl)
                n528 = Subtract(x=w909, y=9) -> (x-y=w900:dbl)
                n529 = vi-ref "goto.vi"() -> (w907:refnum<vi>)
                n530 = property class="VI"(reference=w907, error in=w901) -> ("Name"=w906:string)  [unwired: 2 out]
                n531 = Open VI Reference(type specifier VI Refnum (for type only)=refnum<vi> refnum, vi path=w906, options=128) -> (vi reference=w904:refnum<vi>)  [unwired: 3 in, 1 out]
                n532 = call-by-ref "Start Asynchronous Call"(reference=w904, "Y(mm)"=w897, "X(mm)"=w900) -> ()  [unwired: 10 in, 3 out]
              }
            }
            n533 = property on="currentNO" class="Str"("Value"="B3") -> ()  [unwired: 2 in, 2 out]
          }
          event "B4": Value Change {
            n534 = event-data() -> ("NewVal"=w912:bool)  [unwired: 1 in, 5 out]
            n535 = property on="移动" class="Bool (严格)"() -> ("Value"=w915:bool)  [unwired: 2 in, 2 out]
            n536 = Not(x=w915) -> (.not. x?=w914:bool)
            n537 = And(x=w914, y=w912) -> (x .and. y?=w913:bool)
            n538 = case shown="真" w913 {
              frame False {
              }
              frame True {
                n539 = property on="A1-position-X" class="DigNum (严格)"() -> (error out=w921:errorcluster, "Value"=w928:dbl)  [unwired: 2 in, 1 out]
                n540 = property on="A1-position-Y" class="DigNum (严格)"(error in=w921) -> (error out=w920:errorcluster, "Value"=w917:dbl)  [unwired: 1 in, 1 out]
                n541 = Subtract(x=w917, y=4.5) -> (x-y=w916:dbl)
                n542 = Subtract(x=w928, y=13.5) -> (x-y=w919:dbl)
                n543 = vi-ref "goto.vi"() -> (w926:refnum<vi>)
                n544 = property class="VI"(reference=w926, error in=w920) -> ("Name"=w925:string)  [unwired: 2 out]
                n545 = Open VI Reference(type specifier VI Refnum (for type only)=refnum<vi> refnum, vi path=w925, options=128) -> (vi reference=w923:refnum<vi>)  [unwired: 3 in, 1 out]
                n546 = call-by-ref "Start Asynchronous Call"(reference=w923, "Y(mm)"=w916, "X(mm)"=w919) -> ()  [unwired: 10 in, 3 out]
              }
            }
            n547 = property on="currentNO" class="Str"("Value"="B4") -> ()  [unwired: 2 in, 2 out]
          }
          event "B5": Value Change {
            n548 = event-data() -> ("NewVal"=w931:bool)  [unwired: 1 in, 5 out]
            n549 = property on="移动" class="Bool (严格)"() -> ("Value"=w934:bool)  [unwired: 2 in, 2 out]
            n550 = Not(x=w934) -> (.not. x?=w933:bool)
            n551 = And(x=w933, y=w931) -> (x .and. y?=w932:bool)
            n552 = case shown="真" w932 {
              frame False {
              }
              frame True {
                n553 = property on="A1-position-X" class="DigNum (严格)"() -> (error out=w940:errorcluster, "Value"=w947:dbl)  [unwired: 2 in, 1 out]
                n554 = property on="A1-position-Y" class="DigNum (严格)"(error in=w940) -> (error out=w939:errorcluster, "Value"=w936:dbl)  [unwired: 1 in, 1 out]
                n555 = Subtract(x=w936, y=4.5) -> (x-y=w935:dbl)
                n556 = Subtract(x=w947, y=18) -> (x-y=w938:dbl)
                n557 = vi-ref "goto.vi"() -> (w945:refnum<vi>)
                n558 = property class="VI"(reference=w945, error in=w939) -> ("Name"=w944:string)  [unwired: 2 out]
                n559 = Open VI Reference(type specifier VI Refnum (for type only)=refnum<vi> refnum, vi path=w944, options=128) -> (vi reference=w942:refnum<vi>)  [unwired: 3 in, 1 out]
                n560 = call-by-ref "Start Asynchronous Call"(reference=w942, "Y(mm)"=w935, "X(mm)"=w938) -> ()  [unwired: 10 in, 3 out]
              }
            }
            n561 = property on="currentNO" class="Str"("Value"="B5") -> ()  [unwired: 2 in, 2 out]
          }
          event "B6": Value Change {
            n562 = event-data() -> ("NewVal"=w950:bool)  [unwired: 1 in, 5 out]
            n563 = property on="移动" class="Bool (严格)"() -> ("Value"=w953:bool)  [unwired: 2 in, 2 out]
            n564 = Not(x=w953) -> (.not. x?=w952:bool)
            n565 = And(x=w952, y=w950) -> (x .and. y?=w951:bool)
            n566 = case shown="真" w951 {
              frame False {
              }
              frame True {
                n567 = property on="A1-position-X" class="DigNum (严格)"() -> (error out=w959:errorcluster, "Value"=w966:dbl)  [unwired: 2 in, 1 out]
                n568 = property on="A1-position-Y" class="DigNum (严格)"(error in=w959) -> (error out=w958:errorcluster, "Value"=w955:dbl)  [unwired: 1 in, 1 out]
                n569 = Subtract(x=w955, y=4.5) -> (x-y=w954:dbl)
                n570 = Subtract(x=w966, y=22.5) -> (x-y=w957:dbl)
                n571 = vi-ref "goto.vi"() -> (w964:refnum<vi>)
                n572 = property class="VI"(reference=w964, error in=w958) -> ("Name"=w963:string)  [unwired: 2 out]
                n573 = Open VI Reference(type specifier VI Refnum (for type only)=refnum<vi> refnum, vi path=w963, options=128) -> (vi reference=w961:refnum<vi>)  [unwired: 3 in, 1 out]
                n574 = call-by-ref "Start Asynchronous Call"(reference=w961, "Y(mm)"=w954, "X(mm)"=w957) -> ()  [unwired: 10 in, 3 out]
              }
            }
            n575 = property on="currentNO" class="Str"("Value"="B6") -> ()  [unwired: 2 in, 2 out]
          }
          event "B7": Value Change {
            n576 = event-data() -> ("NewVal"=w969:bool)  [unwired: 1 in, 5 out]
            n577 = property on="移动" class="Bool (严格)"() -> ("Value"=w972:bool)  [unwired: 2 in, 2 out]
            n578 = Not(x=w972) -> (.not. x?=w971:bool)
            n579 = And(x=w971, y=w969) -> (x .and. y?=w970:bool)
            n580 = case shown="真" w970 {
              frame False {
              }
              frame True {
                n581 = property on="A1-position-X" class="DigNum (严格)"() -> (error out=w978:errorcluster, "Value"=w985:dbl)  [unwired: 2 in, 1 out]
                n582 = property on="A1-position-Y" class="DigNum (严格)"(error in=w978) -> (error out=w977:errorcluster, "Value"=w974:dbl)  [unwired: 1 in, 1 out]
                n583 = Subtract(x=w974, y=4.5) -> (x-y=w973:dbl)
                n584 = Subtract(x=w985, y=27) -> (x-y=w976:dbl)
                n585 = vi-ref "goto.vi"() -> (w983:refnum<vi>)
                n586 = property class="VI"(reference=w983, error in=w977) -> ("Name"=w982:string)  [unwired: 2 out]
                n587 = Open VI Reference(type specifier VI Refnum (for type only)=refnum<vi> refnum, vi path=w982, options=128) -> (vi reference=w980:refnum<vi>)  [unwired: 3 in, 1 out]
                n588 = call-by-ref "Start Asynchronous Call"(reference=w980, "Y(mm)"=w973, "X(mm)"=w976) -> ()  [unwired: 10 in, 3 out]
              }
            }
            n589 = property on="currentNO" class="Str"("Value"="B7") -> ()  [unwired: 2 in, 2 out]
          }
          event "B8": Value Change {
            n590 = event-data() -> ("NewVal"=w988:bool)  [unwired: 1 in, 5 out]
            n591 = property on="移动" class="Bool (严格)"() -> ("Value"=w991:bool)  [unwired: 2 in, 2 out]
            n592 = Not(x=w991) -> (.not. x?=w990:bool)
            n593 = And(x=w990, y=w988) -> (x .and. y?=w989:bool)
            n594 = case shown="真" w989 {
              frame False {
              }
              frame True {
                n595 = property on="A1-position-X" class="DigNum (严格)"() -> (error out=w997:errorcluster, "Value"=w1004:dbl)  [unwired: 2 in, 1 out]
                n596 = property on="A1-position-Y" class="DigNum (严格)"(error in=w997) -> (error out=w996:errorcluster, "Value"=w993:dbl)  [unwired: 1 in, 1 out]
                n597 = Subtract(x=w993, y=4.5) -> (x-y=w992:dbl)
                n598 = Subtract(x=w1004, y=31.5) -> (x-y=w995:dbl)
                n599 = vi-ref "goto.vi"() -> (w1002:refnum<vi>)
                n600 = property class="VI"(reference=w1002, error in=w996) -> ("Name"=w1001:string)  [unwired: 2 out]
                n601 = Open VI Reference(type specifier VI Refnum (for type only)=refnum<vi> refnum, vi path=w1001, options=128) -> (vi reference=w999:refnum<vi>)  [unwired: 3 in, 1 out]
                n602 = call-by-ref "Start Asynchronous Call"(reference=w999, "Y(mm)"=w992, "X(mm)"=w995) -> ()  [unwired: 10 in, 3 out]
              }
            }
            n603 = property on="currentNO" class="Str"("Value"="B8") -> ()  [unwired: 2 in, 2 out]
          }
          event "B9": Value Change {
            n604 = event-data() -> ("NewVal"=w1007:bool)  [unwired: 1 in, 5 out]
            n605 = property on="移动" class="Bool (严格)"() -> ("Value"=w1010:bool)  [unwired: 2 in, 2 out]
            n606 = Not(x=w1010) -> (.not. x?=w1009:bool)
            n607 = And(x=w1009, y=w1007) -> (x .and. y?=w1008:bool)
            n608 = case shown="真" w1008 {
              frame False {
              }
              frame True {
                n609 = property on="A1-position-X" class="DigNum (严格)"() -> (error out=w1016:errorcluster, "Value"=w1023:dbl)  [unwired: 2 in, 1 out]
                n610 = property on="A1-position-Y" class="DigNum (严格)"(error in=w1016) -> (error out=w1015:errorcluster, "Value"=w1012:dbl)  [unwired: 1 in, 1 out]
                n611 = Subtract(x=w1012, y=4.5) -> (x-y=w1011:dbl)
                n612 = Subtract(x=w1023, y=36) -> (x-y=w1014:dbl)
                n613 = vi-ref "goto.vi"() -> (w1021:refnum<vi>)
                n614 = property class="VI"(reference=w1021, error in=w1015) -> ("Name"=w1020:string)  [unwired: 2 out]
                n615 = Open VI Reference(type specifier VI Refnum (for type only)=refnum<vi> refnum, vi path=w1020, options=128) -> (vi reference=w1018:refnum<vi>)  [unwired: 3 in, 1 out]
                n616 = call-by-ref "Start Asynchronous Call"(reference=w1018, "Y(mm)"=w1011, "X(mm)"=w1014) -> ()  [unwired: 10 in, 3 out]
              }
            }
            n617 = property on="currentNO" class="Str"("Value"="B9") -> ()  [unwired: 2 in, 2 out]
          }
          event "B10": Value Change {
            n618 = event-data() -> ("NewVal"=w1026:bool)  [unwired: 1 in, 5 out]
            n619 = property on="移动" class="Bool (严格)"() -> ("Value"=w1029:bool)  [unwired: 2 in, 2 out]
            n620 = Not(x=w1029) -> (.not. x?=w1028:bool)
            n621 = And(x=w1028, y=w1026) -> (x .and. y?=w1027:bool)
            n622 = case shown="真" w1027 {
              frame False {
              }
              frame True {
                n623 = property on="A1-position-X" class="DigNum (严格)"() -> (error out=w1035:errorcluster, "Value"=w1042:dbl)  [unwired: 2 in, 1 out]
                n624 = property on="A1-position-Y" class="DigNum (严格)"(error in=w1035) -> (error out=w1034:errorcluster, "Value"=w1031:dbl)  [unwired: 1 in, 1 out]
                n625 = Subtract(x=w1031, y=4.5) -> (x-y=w1030:dbl)
                n626 = Subtract(x=w1042, y=40.5) -> (x-y=w1033:dbl)
                n627 = vi-ref "goto.vi"() -> (w1040:refnum<vi>)
                n628 = property class="VI"(reference=w1040, error in=w1034) -> ("Name"=w1039:string)  [unwired: 2 out]
                n629 = Open VI Reference(type specifier VI Refnum (for type only)=refnum<vi> refnum, vi path=w1039, options=128) -> (vi reference=w1037:refnum<vi>)  [unwired: 3 in, 1 out]
                n630 = call-by-ref "Start Asynchronous Call"(reference=w1037, "Y(mm)"=w1030, "X(mm)"=w1033) -> ()  [unwired: 10 in, 3 out]
              }
            }
            n631 = property on="currentNO" class="Str"("Value"="B10") -> ()  [unwired: 2 in, 2 out]
          }
          event "B11": Value Change {
            n632 = event-data() -> ("NewVal"=w1045:bool)  [unwired: 1 in, 5 out]
            n633 = property on="移动" class="Bool (严格)"() -> ("Value"=w1048:bool)  [unwired: 2 in, 2 out]
            n634 = Not(x=w1048) -> (.not. x?=w1047:bool)
            n635 = And(x=w1047, y=w1045) -> (x .and. y?=w1046:bool)
            n636 = case shown="真" w1046 {
              frame False {
              }
              frame True {
                n637 = property on="A1-position-X" class="DigNum (严格)"() -> (error out=w1054:errorcluster, "Value"=w1061:dbl)  [unwired: 2 in, 1 out]
                n638 = property on="A1-position-Y" class="DigNum (严格)"(error in=w1054) -> (error out=w1053:errorcluster, "Value"=w1050:dbl)  [unwired: 1 in, 1 out]
                n639 = Subtract(x=w1050, y=4.5) -> (x-y=w1049:dbl)
                n640 = Subtract(x=w1061, y=45) -> (x-y=w1052:dbl)
                n641 = vi-ref "goto.vi"() -> (w1059:refnum<vi>)
                n642 = property class="VI"(reference=w1059, error in=w1053) -> ("Name"=w1058:string)  [unwired: 2 out]
                n643 = Open VI Reference(type specifier VI Refnum (for type only)=refnum<vi> refnum, vi path=w1058, options=128) -> (vi reference=w1056:refnum<vi>)  [unwired: 3 in, 1 out]
                n644 = call-by-ref "Start Asynchronous Call"(reference=w1056, "Y(mm)"=w1049, "X(mm)"=w1052) -> ()  [unwired: 10 in, 3 out]
              }
            }
            n645 = property on="currentNO" class="Str"("Value"="B11") -> ()  [unwired: 2 in, 2 out]
          }
          event "B12": Value Change {
            n646 = event-data() -> ("NewVal"=w1064:bool)  [unwired: 1 in, 5 out]
            n647 = property on="移动" class="Bool (严格)"() -> ("Value"=w1067:bool)  [unwired: 2 in, 2 out]
            n648 = Not(x=w1067) -> (.not. x?=w1066:bool)
            n649 = And(x=w1066, y=w1064) -> (x .and. y?=w1065:bool)
            n650 = case shown="真" w1065 {
              frame False {
              }
              frame True {
                n651 = property on="A1-position-X" class="DigNum (严格)"() -> (error out=w1073:errorcluster, "Value"=w1080:dbl)  [unwired: 2 in, 1 out]
                n652 = property on="A1-position-Y" class="DigNum (严格)"(error in=w1073) -> (error out=w1072:errorcluster, "Value"=w1069:dbl)  [unwired: 1 in, 1 out]
                n653 = Subtract(x=w1069, y=4.5) -> (x-y=w1068:dbl)
                n654 = Subtract(x=w1080, y=49.5) -> (x-y=w1071:dbl)
                n655 = vi-ref "goto.vi"() -> (w1078:refnum<vi>)
                n656 = property class="VI"(reference=w1078, error in=w1072) -> ("Name"=w1077:string)  [unwired: 2 out]
                n657 = Open VI Reference(type specifier VI Refnum (for type only)=refnum<vi> refnum, vi path=w1077, options=128) -> (vi reference=w1075:refnum<vi>)  [unwired: 3 in, 1 out]
                n658 = call-by-ref "Start Asynchronous Call"(reference=w1075, "Y(mm)"=w1068, "X(mm)"=w1071) -> ()  [unwired: 10 in, 3 out]
              }
            }
            n659 = property on="currentNO" class="Str"("Value"="B12") -> ()  [unwired: 2 in, 2 out]
          }
          event "C1": Value Change {
            n660 = event-data() -> ("NewVal"=w1083:bool)  [unwired: 1 in, 5 out]
            n661 = property on="移动" class="Bool (严格)"() -> ("Value"=w1086:bool)  [unwired: 2 in, 2 out]
            n662 = Not(x=w1086) -> (.not. x?=w1085:bool)
            n663 = And(x=w1085, y=w1083) -> (x .and. y?=w1084:bool)
            n664 = case shown="真" w1084 {
              frame False {
              }
              frame True {
                n665 = property on="A1-position-X" class="DigNum (严格)"() -> (error out=w1092:errorcluster, "Value"=w1099:dbl)  [unwired: 2 in, 1 out]
                n666 = property on="A1-position-Y" class="DigNum (严格)"(error in=w1092) -> (error out=w1091:errorcluster, "Value"=w1088:dbl)  [unwired: 1 in, 1 out]
                n667 = Subtract(x=w1088, y=9) -> (x-y=w1087:dbl)
                n668 = Subtract(x=w1099, y=0) -> (x-y=w1090:dbl)
                n669 = vi-ref "goto.vi"() -> (w1097:refnum<vi>)
                n670 = property class="VI"(reference=w1097, error in=w1091) -> ("Name"=w1096:string)  [unwired: 2 out]
                n671 = Open VI Reference(type specifier VI Refnum (for type only)=refnum<vi> refnum, vi path=w1096, options=128) -> (vi reference=w1094:refnum<vi>)  [unwired: 3 in, 1 out]
                n672 = call-by-ref "Start Asynchronous Call"(reference=w1094, "Y(mm)"=w1087, "X(mm)"=w1090) -> ()  [unwired: 10 in, 3 out]
              }
            }
            n673 = property on="currentNO" class="Str"("Value"="C1") -> ()  [unwired: 2 in, 2 out]
          }
          event "C2": Value Change {
            n674 = event-data() -> ("NewVal"=w1102:bool)  [unwired: 1 in, 5 out]
            n675 = property on="移动" class="Bool (严格)"() -> ("Value"=w1105:bool)  [unwired: 2 in, 2 out]
            n676 = Not(x=w1105) -> (.not. x?=w1104:bool)
            n677 = And(x=w1104, y=w1102) -> (x .and. y?=w1103:bool)
            n678 = case shown="真" w1103 {
              frame False {
              }
              frame True {
                n679 = property on="A1-position-X" class="DigNum (严格)"() -> (error out=w1111:errorcluster, "Value"=w1118:dbl)  [unwired: 2 in, 1 out]
                n680 = property on="A1-position-Y" class="DigNum (严格)"(error in=w1111) -> (error out=w1110:errorcluster, "Value"=w1107:dbl)  [unwired: 1 in, 1 out]
                n681 = Subtract(x=w1107, y=9) -> (x-y=w1106:dbl)
                n682 = Subtract(x=w1118, y=4.5) -> (x-y=w1109:dbl)
                n683 = vi-ref "goto.vi"() -> (w1116:refnum<vi>)
                n684 = property class="VI"(reference=w1116, error in=w1110) -> ("Name"=w1115:string)  [unwired: 2 out]
                n685 = Open VI Reference(type specifier VI Refnum (for type only)=refnum<vi> refnum, vi path=w1115, options=128) -> (vi reference=w1113:refnum<vi>)  [unwired: 3 in, 1 out]
                n686 = call-by-ref "Start Asynchronous Call"(reference=w1113, "Y(mm)"=w1106, "X(mm)"=w1109) -> ()  [unwired: 10 in, 3 out]
              }
            }
            n687 = property on="currentNO" class="Str"("Value"="C2") -> ()  [unwired: 2 in, 2 out]
          }
          event "C3": Value Change {
            n688 = event-data() -> ("NewVal"=w1121:bool)  [unwired: 1 in, 5 out]
            n689 = property on="移动" class="Bool (严格)"() -> ("Value"=w1124:bool)  [unwired: 2 in, 2 out]
            n690 = Not(x=w1124) -> (.not. x?=w1123:bool)
            n691 = And(x=w1123, y=w1121) -> (x .and. y?=w1122:bool)
            n692 = case shown="真" w1122 {
              frame False {
              }
              frame True {
                n693 = property on="A1-position-X" class="DigNum (严格)"() -> (error out=w1130:errorcluster, "Value"=w1137:dbl)  [unwired: 2 in, 1 out]
                n694 = property on="A1-position-Y" class="DigNum (严格)"(error in=w1130) -> (error out=w1129:errorcluster, "Value"=w1126:dbl)  [unwired: 1 in, 1 out]
                n695 = Subtract(x=w1126, y=9) -> (x-y=w1125:dbl)
                n696 = Subtract(x=w1137, y=9) -> (x-y=w1128:dbl)
                n697 = vi-ref "goto.vi"() -> (w1135:refnum<vi>)
                n698 = property class="VI"(reference=w1135, error in=w1129) -> ("Name"=w1134:string)  [unwired: 2 out]
                n699 = Open VI Reference(type specifier VI Refnum (for type only)=refnum<vi> refnum, vi path=w1134, options=128) -> (vi reference=w1132:refnum<vi>)  [unwired: 3 in, 1 out]
                n700 = call-by-ref "Start Asynchronous Call"(reference=w1132, "Y(mm)"=w1125, "X(mm)"=w1128) -> ()  [unwired: 10 in, 3 out]
              }
            }
            n701 = property on="currentNO" class="Str"("Value"="C3") -> ()  [unwired: 2 in, 2 out]
          }
          event "C4": Value Change {
            n702 = event-data() -> ("NewVal"=w1140:bool)  [unwired: 1 in, 5 out]
            n703 = property on="移动" class="Bool (严格)"() -> ("Value"=w1143:bool)  [unwired: 2 in, 2 out]
            n704 = Not(x=w1143) -> (.not. x?=w1142:bool)
            n705 = And(x=w1142, y=w1140) -> (x .and. y?=w1141:bool)
            n706 = case shown="真" w1141 {
              frame False {
              }
              frame True {
                n707 = property on="A1-position-X" class="DigNum (严格)"() -> (error out=w1149:errorcluster, "Value"=w1156:dbl)  [unwired: 2 in, 1 out]
                n708 = property on="A1-position-Y" class="DigNum (严格)"(error in=w1149) -> (error out=w1148:errorcluster, "Value"=w1145:dbl)  [unwired: 1 in, 1 out]
                n709 = Subtract(x=w1145, y=9) -> (x-y=w1144:dbl)
                n710 = Subtract(x=w1156, y=13.5) -> (x-y=w1147:dbl)
                n711 = vi-ref "goto.vi"() -> (w1154:refnum<vi>)
                n712 = property class="VI"(reference=w1154, error in=w1148) -> ("Name"=w1153:string)  [unwired: 2 out]
                n713 = Open VI Reference(type specifier VI Refnum (for type only)=refnum<vi> refnum, vi path=w1153, options=128) -> (vi reference=w1151:refnum<vi>)  [unwired: 3 in, 1 out]
                n714 = call-by-ref "Start Asynchronous Call"(reference=w1151, "Y(mm)"=w1144, "X(mm)"=w1147) -> ()  [unwired: 10 in, 3 out]
              }
            }
            n715 = property on="currentNO" class="Str"("Value"="C4") -> ()  [unwired: 2 in, 2 out]
          }
          event "C5": Value Change {
            n716 = event-data() -> ("NewVal"=w1159:bool)  [unwired: 1 in, 5 out]
            n717 = property on="移动" class="Bool (严格)"() -> ("Value"=w1162:bool)  [unwired: 2 in, 2 out]
            n718 = Not(x=w1162) -> (.not. x?=w1161:bool)
            n719 = And(x=w1161, y=w1159) -> (x .and. y?=w1160:bool)
            n720 = case shown="真" w1160 {
              frame False {
              }
              frame True {
                n721 = property on="A1-position-X" class="DigNum (严格)"() -> (error out=w1168:errorcluster, "Value"=w1175:dbl)  [unwired: 2 in, 1 out]
                n722 = property on="A1-position-Y" class="DigNum (严格)"(error in=w1168) -> (error out=w1167:errorcluster, "Value"=w1164:dbl)  [unwired: 1 in, 1 out]
                n723 = Subtract(x=w1164, y=9) -> (x-y=w1163:dbl)
                n724 = Subtract(x=w1175, y=18) -> (x-y=w1166:dbl)
                n725 = vi-ref "goto.vi"() -> (w1173:refnum<vi>)
                n726 = property class="VI"(reference=w1173, error in=w1167) -> ("Name"=w1172:string)  [unwired: 2 out]
                n727 = Open VI Reference(type specifier VI Refnum (for type only)=refnum<vi> refnum, vi path=w1172, options=128) -> (vi reference=w1170:refnum<vi>)  [unwired: 3 in, 1 out]
                n728 = call-by-ref "Start Asynchronous Call"(reference=w1170, "Y(mm)"=w1163, "X(mm)"=w1166) -> ()  [unwired: 10 in, 3 out]
              }
            }
            n729 = property on="currentNO" class="Str"("Value"="C5") -> ()  [unwired: 2 in, 2 out]
          }
          event "C6": Value Change {
            n730 = event-data() -> ("NewVal"=w1178:bool)  [unwired: 1 in, 5 out]
            n731 = property on="移动" class="Bool (严格)"() -> ("Value"=w1181:bool)  [unwired: 2 in, 2 out]
            n732 = Not(x=w1181) -> (.not. x?=w1180:bool)
            n733 = And(x=w1180, y=w1178) -> (x .and. y?=w1179:bool)
            n734 = case shown="真" w1179 {
              frame False {
              }
              frame True {
                n735 = property on="A1-position-X" class="DigNum (严格)"() -> (error out=w1187:errorcluster, "Value"=w1194:dbl)  [unwired: 2 in, 1 out]
                n736 = property on="A1-position-Y" class="DigNum (严格)"(error in=w1187) -> (error out=w1186:errorcluster, "Value"=w1183:dbl)  [unwired: 1 in, 1 out]
                n737 = Subtract(x=w1183, y=9) -> (x-y=w1182:dbl)
                n738 = Subtract(x=w1194, y=22.5) -> (x-y=w1185:dbl)
                n739 = vi-ref "goto.vi"() -> (w1192:refnum<vi>)
                n740 = property class="VI"(reference=w1192, error in=w1186) -> ("Name"=w1191:string)  [unwired: 2 out]
                n741 = Open VI Reference(type specifier VI Refnum (for type only)=refnum<vi> refnum, vi path=w1191, options=128) -> (vi reference=w1189:refnum<vi>)  [unwired: 3 in, 1 out]
                n742 = call-by-ref "Start Asynchronous Call"(reference=w1189, "Y(mm)"=w1182, "X(mm)"=w1185) -> ()  [unwired: 10 in, 3 out]
              }
            }
            n743 = property on="currentNO" class="Str"("Value"="C6") -> ()  [unwired: 2 in, 2 out]
          }
          event "C7": Value Change {
            n744 = event-data() -> ("NewVal"=w1197:bool)  [unwired: 1 in, 5 out]
            n745 = property on="移动" class="Bool (严格)"() -> ("Value"=w1200:bool)  [unwired: 2 in, 2 out]
            n746 = Not(x=w1200) -> (.not. x?=w1199:bool)
            n747 = And(x=w1199, y=w1197) -> (x .and. y?=w1198:bool)
            n748 = case shown="真" w1198 {
              frame False {
              }
              frame True {
                n749 = property on="A1-position-X" class="DigNum (严格)"() -> (error out=w1206:errorcluster, "Value"=w1213:dbl)  [unwired: 2 in, 1 out]
                n750 = property on="A1-position-Y" class="DigNum (严格)"(error in=w1206) -> (error out=w1205:errorcluster, "Value"=w1202:dbl)  [unwired: 1 in, 1 out]
                n751 = Subtract(x=w1202, y=9) -> (x-y=w1201:dbl)
                n752 = Subtract(x=w1213, y=27) -> (x-y=w1204:dbl)
                n753 = vi-ref "goto.vi"() -> (w1211:refnum<vi>)
                n754 = property class="VI"(reference=w1211, error in=w1205) -> ("Name"=w1210:string)  [unwired: 2 out]
                n755 = Open VI Reference(type specifier VI Refnum (for type only)=refnum<vi> refnum, vi path=w1210, options=128) -> (vi reference=w1208:refnum<vi>)  [unwired: 3 in, 1 out]
                n756 = call-by-ref "Start Asynchronous Call"(reference=w1208, "Y(mm)"=w1201, "X(mm)"=w1204) -> ()  [unwired: 10 in, 3 out]
              }
            }
            n757 = property on="currentNO" class="Str"("Value"="C7") -> ()  [unwired: 2 in, 2 out]
          }
          event "C8": Value Change {
            n758 = event-data() -> ("NewVal"=w1216:bool)  [unwired: 1 in, 5 out]
            n759 = property on="移动" class="Bool (严格)"() -> ("Value"=w1219:bool)  [unwired: 2 in, 2 out]
            n760 = Not(x=w1219) -> (.not. x?=w1218:bool)
            n761 = And(x=w1218, y=w1216) -> (x .and. y?=w1217:bool)
            n762 = case shown="真" w1217 {
              frame False {
              }
              frame True {
                n763 = property on="A1-position-X" class="DigNum (严格)"() -> (error out=w1225:errorcluster, "Value"=w1232:dbl)  [unwired: 2 in, 1 out]
                n764 = property on="A1-position-Y" class="DigNum (严格)"(error in=w1225) -> (error out=w1224:errorcluster, "Value"=w1221:dbl)  [unwired: 1 in, 1 out]
                n765 = Subtract(x=w1221, y=9) -> (x-y=w1220:dbl)
                n766 = Subtract(x=w1232, y=31.5) -> (x-y=w1223:dbl)
                n767 = vi-ref "goto.vi"() -> (w1230:refnum<vi>)
                n768 = property class="VI"(reference=w1230, error in=w1224) -> ("Name"=w1229:string)  [unwired: 2 out]
                n769 = Open VI Reference(type specifier VI Refnum (for type only)=refnum<vi> refnum, vi path=w1229, options=128) -> (vi reference=w1227:refnum<vi>)  [unwired: 3 in, 1 out]
                n770 = call-by-ref "Start Asynchronous Call"(reference=w1227, "Y(mm)"=w1220, "X(mm)"=w1223) -> ()  [unwired: 10 in, 3 out]
              }
            }
            n771 = property on="currentNO" class="Str"("Value"="C8") -> ()  [unwired: 2 in, 2 out]
          }
          event "C9": Value Change {
            n772 = event-data() -> ("NewVal"=w1235:bool)  [unwired: 1 in, 5 out]
            n773 = property on="移动" class="Bool (严格)"() -> ("Value"=w1238:bool)  [unwired: 2 in, 2 out]
            n774 = Not(x=w1238) -> (.not. x?=w1237:bool)
            n775 = And(x=w1237, y=w1235) -> (x .and. y?=w1236:bool)
            n776 = case shown="真" w1236 {
              frame False {
              }
              frame True {
                n777 = property on="A1-position-X" class="DigNum (严格)"() -> (error out=w1244:errorcluster, "Value"=w1251:dbl)  [unwired: 2 in, 1 out]
                n778 = property on="A1-position-Y" class="DigNum (严格)"(error in=w1244) -> (error out=w1243:errorcluster, "Value"=w1240:dbl)  [unwired: 1 in, 1 out]
                n779 = Subtract(x=w1240, y=9) -> (x-y=w1239:dbl)
                n780 = Subtract(x=w1251, y=36) -> (x-y=w1242:dbl)
                n781 = vi-ref "goto.vi"() -> (w1249:refnum<vi>)
                n782 = property class="VI"(reference=w1249, error in=w1243) -> ("Name"=w1248:string)  [unwired: 2 out]
                n783 = Open VI Reference(type specifier VI Refnum (for type only)=refnum<vi> refnum, vi path=w1248, options=128) -> (vi reference=w1246:refnum<vi>)  [unwired: 3 in, 1 out]
                n784 = call-by-ref "Start Asynchronous Call"(reference=w1246, "Y(mm)"=w1239, "X(mm)"=w1242) -> ()  [unwired: 10 in, 3 out]
              }
            }
            n785 = property on="currentNO" class="Str"("Value"="C9") -> ()  [unwired: 2 in, 2 out]
          }
          event "C10": Value Change {
            n786 = event-data() -> ("NewVal"=w1254:bool)  [unwired: 1 in, 5 out]
            n787 = property on="移动" class="Bool (严格)"() -> ("Value"=w1257:bool)  [unwired: 2 in, 2 out]
            n788 = Not(x=w1257) -> (.not. x?=w1256:bool)
            n789 = And(x=w1256, y=w1254) -> (x .and. y?=w1255:bool)
            n790 = case shown="真" w1255 {
              frame False {
              }
              frame True {
                n791 = property on="A1-position-X" class="DigNum (严格)"() -> (error out=w1263:errorcluster, "Value"=w1270:dbl)  [unwired: 2 in, 1 out]
                n792 = property on="A1-position-Y" class="DigNum (严格)"(error in=w1263) -> (error out=w1262:errorcluster, "Value"=w1259:dbl)  [unwired: 1 in, 1 out]
                n793 = Subtract(x=w1259, y=9) -> (x-y=w1258:dbl)
                n794 = Subtract(x=w1270, y=40.5) -> (x-y=w1261:dbl)
                n795 = vi-ref "goto.vi"() -> (w1268:refnum<vi>)
                n796 = property class="VI"(reference=w1268, error in=w1262) -> ("Name"=w1267:string)  [unwired: 2 out]
                n797 = Open VI Reference(type specifier VI Refnum (for type only)=refnum<vi> refnum, vi path=w1267, options=128) -> (vi reference=w1265:refnum<vi>)  [unwired: 3 in, 1 out]
                n798 = call-by-ref "Start Asynchronous Call"(reference=w1265, "Y(mm)"=w1258, "X(mm)"=w1261) -> ()  [unwired: 10 in, 3 out]
              }
            }
            n799 = property on="currentNO" class="Str"("Value"="C10") -> ()  [unwired: 2 in, 2 out]
          }
          event "C11": Value Change {
            n800 = event-data() -> ("NewVal"=w1273:bool)  [unwired: 1 in, 5 out]
            n801 = property on="移动" class="Bool (严格)"() -> ("Value"=w1276:bool)  [unwired: 2 in, 2 out]
            n802 = Not(x=w1276) -> (.not. x?=w1275:bool)
            n803 = And(x=w1275, y=w1273) -> (x .and. y?=w1274:bool)
            n804 = case shown="真" w1274 {
              frame False {
              }
              frame True {
                n805 = property on="A1-position-X" class="DigNum (严格)"() -> (error out=w1282:errorcluster, "Value"=w1289:dbl)  [unwired: 2 in, 1 out]
                n806 = property on="A1-position-Y" class="DigNum (严格)"(error in=w1282) -> (error out=w1281:errorcluster, "Value"=w1278:dbl)  [unwired: 1 in, 1 out]
                n807 = Subtract(x=w1278, y=9) -> (x-y=w1277:dbl)
                n808 = Subtract(x=w1289, y=45) -> (x-y=w1280:dbl)
                n809 = vi-ref "goto.vi"() -> (w1287:refnum<vi>)
                n810 = property class="VI"(reference=w1287, error in=w1281) -> ("Name"=w1286:string)  [unwired: 2 out]
                n811 = Open VI Reference(type specifier VI Refnum (for type only)=refnum<vi> refnum, vi path=w1286, options=128) -> (vi reference=w1284:refnum<vi>)  [unwired: 3 in, 1 out]
                n812 = call-by-ref "Start Asynchronous Call"(reference=w1284, "Y(mm)"=w1277, "X(mm)"=w1280) -> ()  [unwired: 10 in, 3 out]
              }
            }
            n813 = property on="currentNO" class="Str"("Value"="C11") -> ()  [unwired: 2 in, 2 out]
          }
          event "C12": Value Change {
            n814 = event-data() -> ("NewVal"=w1292:bool)  [unwired: 1 in, 5 out]
            n815 = property on="移动" class="Bool (严格)"() -> ("Value"=w1295:bool)  [unwired: 2 in, 2 out]
            n816 = Not(x=w1295) -> (.not. x?=w1294:bool)
            n817 = And(x=w1294, y=w1292) -> (x .and. y?=w1293:bool)
            n818 = case shown="真" w1293 {
              frame False {
              }
              frame True {
                n819 = property on="A1-position-X" class="DigNum (严格)"() -> (error out=w1301:errorcluster, "Value"=w1308:dbl)  [unwired: 2 in, 1 out]
                n820 = property on="A1-position-Y" class="DigNum (严格)"(error in=w1301) -> (error out=w1300:errorcluster, "Value"=w1297:dbl)  [unwired: 1 in, 1 out]
                n821 = Subtract(x=w1297, y=9) -> (x-y=w1296:dbl)
                n822 = Subtract(x=w1308, y=49.5) -> (x-y=w1299:dbl)
                n823 = vi-ref "goto.vi"() -> (w1306:refnum<vi>)
                n824 = property class="VI"(reference=w1306, error in=w1300) -> ("Name"=w1305:string)  [unwired: 2 out]
                n825 = Open VI Reference(type specifier VI Refnum (for type only)=refnum<vi> refnum, vi path=w1305, options=128) -> (vi reference=w1303:refnum<vi>)  [unwired: 3 in, 1 out]
                n826 = call-by-ref "Start Asynchronous Call"(reference=w1303, "Y(mm)"=w1296, "X(mm)"=w1299) -> ()  [unwired: 10 in, 3 out]
              }
            }
            n827 = property on="currentNO" class="Str"("Value"="C12") -> ()  [unwired: 2 in, 2 out]
          }
          event "D1": Value Change {
            n828 = event-data() -> ("NewVal"=w1311:bool)  [unwired: 1 in, 5 out]
            n829 = property on="移动" class="Bool (严格)"() -> ("Value"=w1314:bool)  [unwired: 2 in, 2 out]
            n830 = Not(x=w1314) -> (.not. x?=w1313:bool)
            n831 = And(x=w1313, y=w1311) -> (x .and. y?=w1312:bool)
            n832 = case shown="真" w1312 {
              frame False {
              }
              frame True {
                n833 = property on="A1-position-X" class="DigNum (严格)"() -> (error out=w1320:errorcluster, "Value"=w1327:dbl)  [unwired: 2 in, 1 out]
                n834 = property on="A1-position-Y" class="DigNum (严格)"(error in=w1320) -> (error out=w1319:errorcluster, "Value"=w1316:dbl)  [unwired: 1 in, 1 out]
                n835 = Subtract(x=w1316, y=13.5) -> (x-y=w1315:dbl)
                n836 = Subtract(x=w1327, y=0) -> (x-y=w1318:dbl)
                n837 = vi-ref "goto.vi"() -> (w1325:refnum<vi>)
                n838 = property class="VI"(reference=w1325, error in=w1319) -> ("Name"=w1324:string)  [unwired: 2 out]
                n839 = Open VI Reference(type specifier VI Refnum (for type only)=refnum<vi> refnum, vi path=w1324, options=128) -> (vi reference=w1322:refnum<vi>)  [unwired: 3 in, 1 out]
                n840 = call-by-ref "Start Asynchronous Call"(reference=w1322, "Y(mm)"=w1315, "X(mm)"=w1318) -> ()  [unwired: 10 in, 3 out]
              }
            }
            n841 = property on="currentNO" class="Str"("Value"="D1") -> ()  [unwired: 2 in, 2 out]
          }
          event "D2": Value Change {
            n842 = event-data() -> ("NewVal"=w1330:bool)  [unwired: 1 in, 5 out]
            n843 = property on="移动" class="Bool (严格)"() -> ("Value"=w1333:bool)  [unwired: 2 in, 2 out]
            n844 = Not(x=w1333) -> (.not. x?=w1332:bool)
            n845 = And(x=w1332, y=w1330) -> (x .and. y?=w1331:bool)
            n846 = case shown="真" w1331 {
              frame False {
              }
              frame True {
                n847 = property on="A1-position-X" class="DigNum (严格)"() -> (error out=w1339:errorcluster, "Value"=w1346:dbl)  [unwired: 2 in, 1 out]
                n848 = property on="A1-position-Y" class="DigNum (严格)"(error in=w1339) -> (error out=w1338:errorcluster, "Value"=w1335:dbl)  [unwired: 1 in, 1 out]
                n849 = Subtract(x=w1335, y=13.5) -> (x-y=w1334:dbl)
                n850 = Subtract(x=w1346, y=4.5) -> (x-y=w1337:dbl)
                n851 = vi-ref "goto.vi"() -> (w1344:refnum<vi>)
                n852 = property class="VI"(reference=w1344, error in=w1338) -> ("Name"=w1343:string)  [unwired: 2 out]
                n853 = Open VI Reference(type specifier VI Refnum (for type only)=refnum<vi> refnum, vi path=w1343, options=128) -> (vi reference=w1341:refnum<vi>)  [unwired: 3 in, 1 out]
                n854 = call-by-ref "Start Asynchronous Call"(reference=w1341, "Y(mm)"=w1334, "X(mm)"=w1337) -> ()  [unwired: 10 in, 3 out]
              }
            }
            n855 = property on="currentNO" class="Str"("Value"="D2") -> ()  [unwired: 2 in, 2 out]
          }
          event "D3": Value Change {
            n856 = event-data() -> ("NewVal"=w1349:bool)  [unwired: 1 in, 5 out]
            n857 = property on="移动" class="Bool (严格)"() -> ("Value"=w1352:bool)  [unwired: 2 in, 2 out]
            n858 = Not(x=w1352) -> (.not. x?=w1351:bool)
            n859 = And(x=w1351, y=w1349) -> (x .and. y?=w1350:bool)
            n860 = case shown="真" w1350 {
              frame False {
              }
              frame True {
                n861 = property on="A1-position-X" class="DigNum (严格)"() -> (error out=w1358:errorcluster, "Value"=w1365:dbl)  [unwired: 2 in, 1 out]
                n862 = property on="A1-position-Y" class="DigNum (严格)"(error in=w1358) -> (error out=w1357:errorcluster, "Value"=w1354:dbl)  [unwired: 1 in, 1 out]
                n863 = Subtract(x=w1354, y=13.5) -> (x-y=w1353:dbl)
                n864 = Subtract(x=w1365, y=9) -> (x-y=w1356:dbl)
                n865 = vi-ref "goto.vi"() -> (w1363:refnum<vi>)
                n866 = property class="VI"(reference=w1363, error in=w1357) -> ("Name"=w1362:string)  [unwired: 2 out]
                n867 = Open VI Reference(type specifier VI Refnum (for type only)=refnum<vi> refnum, vi path=w1362, options=128) -> (vi reference=w1360:refnum<vi>)  [unwired: 3 in, 1 out]
                n868 = call-by-ref "Start Asynchronous Call"(reference=w1360, "Y(mm)"=w1353, "X(mm)"=w1356) -> ()  [unwired: 10 in, 3 out]
              }
            }
            n869 = property on="currentNO" class="Str"("Value"="D3") -> ()  [unwired: 2 in, 2 out]
          }
          event "D4": Value Change {
            n870 = event-data() -> ("NewVal"=w1368:bool)  [unwired: 1 in, 5 out]
            n871 = property on="移动" class="Bool (严格)"() -> ("Value"=w1371:bool)  [unwired: 2 in, 2 out]
            n872 = Not(x=w1371) -> (.not. x?=w1370:bool)
            n873 = And(x=w1370, y=w1368) -> (x .and. y?=w1369:bool)
            n874 = case shown="真" w1369 {
              frame False {
              }
              frame True {
                n875 = property on="A1-position-X" class="DigNum (严格)"() -> (error out=w1377:errorcluster, "Value"=w1384:dbl)  [unwired: 2 in, 1 out]
                n876 = property on="A1-position-Y" class="DigNum (严格)"(error in=w1377) -> (error out=w1376:errorcluster, "Value"=w1373:dbl)  [unwired: 1 in, 1 out]
                n877 = Subtract(x=w1373, y=13.5) -> (x-y=w1372:dbl)
                n878 = Subtract(x=w1384, y=13.5) -> (x-y=w1375:dbl)
                n879 = vi-ref "goto.vi"() -> (w1382:refnum<vi>)
                n880 = property class="VI"(reference=w1382, error in=w1376) -> ("Name"=w1381:string)  [unwired: 2 out]
                n881 = Open VI Reference(type specifier VI Refnum (for type only)=refnum<vi> refnum, vi path=w1381, options=128) -> (vi reference=w1379:refnum<vi>)  [unwired: 3 in, 1 out]
                n882 = call-by-ref "Start Asynchronous Call"(reference=w1379, "Y(mm)"=w1372, "X(mm)"=w1375) -> ()  [unwired: 10 in, 3 out]
              }
            }
            n883 = property on="currentNO" class="Str"("Value"="D4") -> ()  [unwired: 2 in, 2 out]
          }
          event "D5": Value Change {
            n884 = event-data() -> ("NewVal"=w1387:bool)  [unwired: 1 in, 5 out]
            n885 = property on="移动" class="Bool (严格)"() -> ("Value"=w1390:bool)  [unwired: 2 in, 2 out]
            n886 = Not(x=w1390) -> (.not. x?=w1389:bool)
            n887 = And(x=w1389, y=w1387) -> (x .and. y?=w1388:bool)
            n888 = case shown="真" w1388 {
              frame False {
              }
              frame True {
                n889 = property on="A1-position-X" class="DigNum (严格)"() -> (error out=w1396:errorcluster, "Value"=w1403:dbl)  [unwired: 2 in, 1 out]
                n890 = property on="A1-position-Y" class="DigNum (严格)"(error in=w1396) -> (error out=w1395:errorcluster, "Value"=w1392:dbl)  [unwired: 1 in, 1 out]
                n891 = Subtract(x=w1392, y=13.5) -> (x-y=w1391:dbl)
                n892 = Subtract(x=w1403, y=18) -> (x-y=w1394:dbl)
                n893 = vi-ref "goto.vi"() -> (w1401:refnum<vi>)
                n894 = property class="VI"(reference=w1401, error in=w1395) -> ("Name"=w1400:string)  [unwired: 2 out]
                n895 = Open VI Reference(type specifier VI Refnum (for type only)=refnum<vi> refnum, vi path=w1400, options=128) -> (vi reference=w1398:refnum<vi>)  [unwired: 3 in, 1 out]
                n896 = call-by-ref "Start Asynchronous Call"(reference=w1398, "Y(mm)"=w1391, "X(mm)"=w1394) -> ()  [unwired: 10 in, 3 out]
              }
            }
            n897 = property on="currentNO" class="Str"("Value"="D5") -> ()  [unwired: 2 in, 2 out]
          }
          event "D6": Value Change {
            n898 = event-data() -> ("NewVal"=w1406:bool)  [unwired: 1 in, 5 out]
            n899 = property on="移动" class="Bool (严格)"() -> ("Value"=w1409:bool)  [unwired: 2 in, 2 out]
            n900 = Not(x=w1409) -> (.not. x?=w1408:bool)
            n901 = And(x=w1408, y=w1406) -> (x .and. y?=w1407:bool)
            n902 = case shown="真" w1407 {
              frame False {
              }
              frame True {
                n903 = property on="A1-position-X" class="DigNum (严格)"() -> (error out=w1415:errorcluster, "Value"=w1422:dbl)  [unwired: 2 in, 1 out]
                n904 = property on="A1-position-Y" class="DigNum (严格)"(error in=w1415) -> (error out=w1414:errorcluster, "Value"=w1411:dbl)  [unwired: 1 in, 1 out]
                n905 = Subtract(x=w1411, y=13.5) -> (x-y=w1410:dbl)
                n906 = Subtract(x=w1422, y=22.5) -> (x-y=w1413:dbl)
                n907 = vi-ref "goto.vi"() -> (w1420:refnum<vi>)
                n908 = property class="VI"(reference=w1420, error in=w1414) -> ("Name"=w1419:string)  [unwired: 2 out]
                n909 = Open VI Reference(type specifier VI Refnum (for type only)=refnum<vi> refnum, vi path=w1419, options=128) -> (vi reference=w1417:refnum<vi>)  [unwired: 3 in, 1 out]
                n910 = call-by-ref "Start Asynchronous Call"(reference=w1417, "Y(mm)"=w1410, "X(mm)"=w1413) -> ()  [unwired: 10 in, 3 out]
              }
            }
            n911 = property on="currentNO" class="Str"("Value"="D6") -> ()  [unwired: 2 in, 2 out]
          }
          event "D7": Value Change {
            n912 = event-data() -> ("NewVal"=w1425:bool)  [unwired: 1 in, 5 out]
            n913 = property on="移动" class="Bool (严格)"() -> ("Value"=w1428:bool)  [unwired: 2 in, 2 out]
            n914 = Not(x=w1428) -> (.not. x?=w1427:bool)
            n915 = And(x=w1427, y=w1425) -> (x .and. y?=w1426:bool)
            n916 = case shown="真" w1426 {
              frame False {
              }
              frame True {
                n917 = property on="A1-position-X" class="DigNum (严格)"() -> (error out=w1434:errorcluster, "Value"=w1441:dbl)  [unwired: 2 in, 1 out]
                n918 = property on="A1-position-Y" class="DigNum (严格)"(error in=w1434) -> (error out=w1433:errorcluster, "Value"=w1430:dbl)  [unwired: 1 in, 1 out]
                n919 = Subtract(x=w1430, y=13.5) -> (x-y=w1429:dbl)
                n920 = Subtract(x=w1441, y=27) -> (x-y=w1432:dbl)
                n921 = vi-ref "goto.vi"() -> (w1439:refnum<vi>)
                n922 = property class="VI"(reference=w1439, error in=w1433) -> ("Name"=w1438:string)  [unwired: 2 out]
                n923 = Open VI Reference(type specifier VI Refnum (for type only)=refnum<vi> refnum, vi path=w1438, options=128) -> (vi reference=w1436:refnum<vi>)  [unwired: 3 in, 1 out]
                n924 = call-by-ref "Start Asynchronous Call"(reference=w1436, "Y(mm)"=w1429, "X(mm)"=w1432) -> ()  [unwired: 10 in, 3 out]
              }
            }
            n925 = property on="currentNO" class="Str"("Value"="D7") -> ()  [unwired: 2 in, 2 out]
          }
          event "D8": Value Change {
            n926 = event-data() -> ("NewVal"=w1443:bool)  [unwired: 1 in, 5 out]
            n927 = property on="移动" class="Bool (严格)"() -> ("Value"=w1446:bool)  [unwired: 2 in, 2 out]
            n928 = Not(x=w1446) -> (.not. x?=w1445:bool)
            n929 = And(x=w1445, y=w1443) -> (x .and. y?=w1444:bool)
            n930 = case shown="真" w1444 {
              frame False {
              }
              frame True {
                n931 = property on="A1-position-X" class="DigNum (严格)"() -> (error out=w1453:errorcluster, "Value"=w1460:dbl)  [unwired: 2 in, 1 out]
                n932 = property on="A1-position-Y" class="DigNum (严格)"(error in=w1453) -> (error out=w1452:errorcluster, "Value"=w1449:dbl)  [unwired: 1 in, 1 out]
                n933 = Subtract(x=w1449, y=13.5) -> (x-y=w1448:dbl)
                n934 = Subtract(x=w1460, y=31.5) -> (x-y=w1451:dbl)
                n935 = vi-ref "goto.vi"() -> (w1458:refnum<vi>)
                n936 = property class="VI"(reference=w1458, error in=w1452) -> ("Name"=w1457:string)  [unwired: 2 out]
                n937 = Open VI Reference(type specifier VI Refnum (for type only)=refnum<vi> refnum, vi path=w1457, options=128) -> (vi reference=w1455:refnum<vi>)  [unwired: 3 in, 1 out]
                n938 = call-by-ref "Start Asynchronous Call"(reference=w1455, "Y(mm)"=w1448, "X(mm)"=w1451) -> ()  [unwired: 10 in, 3 out]
              }
            }
            n939 = property on="currentNO" class="Str"("Value"="D8") -> ()  [unwired: 2 in, 2 out]
          }
          event "D9": Value Change {
            n940 = event-data() -> ("NewVal"=w1462:bool)  [unwired: 1 in, 5 out]
            n941 = property on="移动" class="Bool (严格)"() -> ("Value"=w1465:bool)  [unwired: 2 in, 2 out]
            n942 = Not(x=w1465) -> (.not. x?=w1464:bool)
            n943 = And(x=w1464, y=w1462) -> (x .and. y?=w1463:bool)
            n944 = case shown="真" w1463 {
              frame False {
              }
              frame True {
                n945 = property on="A1-position-X" class="DigNum (严格)"() -> (error out=w1472:errorcluster, "Value"=w1479:dbl)  [unwired: 2 in, 1 out]
                n946 = property on="A1-position-Y" class="DigNum (严格)"(error in=w1472) -> (error out=w1471:errorcluster, "Value"=w1468:dbl)  [unwired: 1 in, 1 out]
                n947 = Subtract(x=w1468, y=13.5) -> (x-y=w1467:dbl)
                n948 = Subtract(x=w1479, y=36) -> (x-y=w1470:dbl)
                n949 = vi-ref "goto.vi"() -> (w1477:refnum<vi>)
                n950 = property class="VI"(reference=w1477, error in=w1471) -> ("Name"=w1476:string)  [unwired: 2 out]
                n951 = Open VI Reference(type specifier VI Refnum (for type only)=refnum<vi> refnum, vi path=w1476, options=128) -> (vi reference=w1474:refnum<vi>)  [unwired: 3 in, 1 out]
                n952 = call-by-ref "Start Asynchronous Call"(reference=w1474, "Y(mm)"=w1467, "X(mm)"=w1470) -> ()  [unwired: 10 in, 3 out]
              }
            }
            n953 = property on="currentNO" class="Str"("Value"="D9") -> ()  [unwired: 2 in, 2 out]
          }
          event "D10": Value Change {
            n954 = event-data() -> ("NewVal"=w1481:bool)  [unwired: 1 in, 5 out]
            n955 = property on="移动" class="Bool (严格)"() -> ("Value"=w1484:bool)  [unwired: 2 in, 2 out]
            n956 = Not(x=w1484) -> (.not. x?=w1483:bool)
            n957 = And(x=w1483, y=w1481) -> (x .and. y?=w1482:bool)
            n958 = case shown="真" w1482 {
              frame False {
              }
              frame True {
                n959 = property on="A1-position-X" class="DigNum (严格)"() -> (error out=w1491:errorcluster, "Value"=w1498:dbl)  [unwired: 2 in, 1 out]
                n960 = property on="A1-position-Y" class="DigNum (严格)"(error in=w1491) -> (error out=w1490:errorcluster, "Value"=w1487:dbl)  [unwired: 1 in, 1 out]
                n961 = Subtract(x=w1487, y=13.5) -> (x-y=w1486:dbl)
                n962 = Subtract(x=w1498, y=40.5) -> (x-y=w1489:dbl)
                n963 = vi-ref "goto.vi"() -> (w1496:refnum<vi>)
                n964 = property class="VI"(reference=w1496, error in=w1490) -> ("Name"=w1495:string)  [unwired: 2 out]
                n965 = Open VI Reference(type specifier VI Refnum (for type only)=refnum<vi> refnum, vi path=w1495, options=128) -> (vi reference=w1493:refnum<vi>)  [unwired: 3 in, 1 out]
                n966 = call-by-ref "Start Asynchronous Call"(reference=w1493, "Y(mm)"=w1486, "X(mm)"=w1489) -> ()  [unwired: 10 in, 3 out]
              }
            }
            n967 = property on="currentNO" class="Str"("Value"="D10") -> ()  [unwired: 2 in, 2 out]
          }
          event "D11": Value Change {
            n968 = event-data() -> ("NewVal"=w1500:bool)  [unwired: 1 in, 5 out]
            n969 = property on="移动" class="Bool (严格)"() -> ("Value"=w1503:bool)  [unwired: 2 in, 2 out]
            n970 = Not(x=w1503) -> (.not. x?=w1502:bool)
            n971 = And(x=w1502, y=w1500) -> (x .and. y?=w1501:bool)
            n972 = case shown="真" w1501 {
              frame False {
              }
              frame True {
                n973 = property on="A1-position-X" class="DigNum (严格)"() -> (error out=w1510:errorcluster, "Value"=w1517:dbl)  [unwired: 2 in, 1 out]
                n974 = property on="A1-position-Y" class="DigNum (严格)"(error in=w1510) -> (error out=w1509:errorcluster, "Value"=w1506:dbl)  [unwired: 1 in, 1 out]
                n975 = Subtract(x=w1506, y=13.5) -> (x-y=w1505:dbl)
                n976 = Subtract(x=w1517, y=45) -> (x-y=w1508:dbl)
                n977 = vi-ref "goto.vi"() -> (w1515:refnum<vi>)
                n978 = property class="VI"(reference=w1515, error in=w1509) -> ("Name"=w1514:string)  [unwired: 2 out]
                n979 = Open VI Reference(type specifier VI Refnum (for type only)=refnum<vi> refnum, vi path=w1514, options=128) -> (vi reference=w1512:refnum<vi>)  [unwired: 3 in, 1 out]
                n980 = call-by-ref "Start Asynchronous Call"(reference=w1512, "Y(mm)"=w1505, "X(mm)"=w1508) -> ()  [unwired: 10 in, 3 out]
              }
            }
            n981 = property on="currentNO" class="Str"("Value"="D11") -> ()  [unwired: 2 in, 2 out]
          }
          event "D12": Value Change {
            n982 = event-data() -> ("NewVal"=w1519:bool)  [unwired: 1 in, 5 out]
            n983 = property on="移动" class="Bool (严格)"() -> ("Value"=w1522:bool)  [unwired: 2 in, 2 out]
            n984 = Not(x=w1522) -> (.not. x?=w1521:bool)
            n985 = And(x=w1521, y=w1519) -> (x .and. y?=w1520:bool)
            n986 = case shown="真" w1520 {
              frame False {
              }
              frame True {
                n987 = property on="A1-position-X" class="DigNum (严格)"() -> (error out=w1529:errorcluster, "Value"=w1536:dbl)  [unwired: 2 in, 1 out]
                n988 = property on="A1-position-Y" class="DigNum (严格)"(error in=w1529) -> (error out=w1528:errorcluster, "Value"=w1525:dbl)  [unwired: 1 in, 1 out]
                n989 = Subtract(x=w1525, y=13.5) -> (x-y=w1524:dbl)
                n990 = Subtract(x=w1536, y=49.5) -> (x-y=w1527:dbl)
                n991 = vi-ref "goto.vi"() -> (w1534:refnum<vi>)
                n992 = property class="VI"(reference=w1534, error in=w1528) -> ("Name"=w1533:string)  [unwired: 2 out]
                n993 = Open VI Reference(type specifier VI Refnum (for type only)=refnum<vi> refnum, vi path=w1533, options=128) -> (vi reference=w1531:refnum<vi>)  [unwired: 3 in, 1 out]
                n994 = call-by-ref "Start Asynchronous Call"(reference=w1531, "Y(mm)"=w1524, "X(mm)"=w1527) -> ()  [unwired: 10 in, 3 out]
              }
            }
            n995 = property on="currentNO" class="Str"("Value"="D12") -> ()  [unwired: 2 in, 2 out]
          }
          event "E1": Value Change {
            n996 = event-data() -> ("NewVal"=w1538:bool)  [unwired: 1 in, 5 out]
            n997 = property on="移动" class="Bool (严格)"() -> ("Value"=w1541:bool)  [unwired: 2 in, 2 out]
            n998 = Not(x=w1541) -> (.not. x?=w1540:bool)
            n999 = And(x=w1540, y=w1538) -> (x .and. y?=w1539:bool)
            n1000 = case shown="真" w1539 {
              frame False {
              }
              frame True {
                n1001 = property on="A1-position-X" class="DigNum (严格)"() -> (error out=w1548:errorcluster, "Value"=w1555:dbl)  [unwired: 2 in, 1 out]
                n1002 = property on="A1-position-Y" class="DigNum (严格)"(error in=w1548) -> (error out=w1547:errorcluster, "Value"=w1544:dbl)  [unwired: 1 in, 1 out]
                n1003 = Subtract(x=w1544, y=18.0) -> (x-y=w1543:dbl)
                n1004 = Subtract(x=w1555, y=0) -> (x-y=w1546:dbl)
                n1005 = vi-ref "goto.vi"() -> (w1553:refnum<vi>)
                n1006 = property class="VI"(reference=w1553, error in=w1547) -> ("Name"=w1552:string)  [unwired: 2 out]
                n1007 = Open VI Reference(type specifier VI Refnum (for type only)=refnum<vi> refnum, vi path=w1552, options=128) -> (vi reference=w1550:refnum<vi>)  [unwired: 3 in, 1 out]
                n1008 = call-by-ref "Start Asynchronous Call"(reference=w1550, "Y(mm)"=w1543, "X(mm)"=w1546) -> ()  [unwired: 10 in, 3 out]
              }
            }
            n1009 = property on="currentNO" class="Str"("Value"="E1") -> ()  [unwired: 2 in, 2 out]
          }
          event "E2": Value Change {
            n1010 = event-data() -> ("NewVal"=w1557:bool)  [unwired: 1 in, 5 out]
            n1011 = property on="移动" class="Bool (严格)"() -> ("Value"=w1560:bool)  [unwired: 2 in, 2 out]
            n1012 = Not(x=w1560) -> (.not. x?=w1559:bool)
            n1013 = And(x=w1559, y=w1557) -> (x .and. y?=w1558:bool)
            n1014 = case shown="真" w1558 {
              frame False {
              }
              frame True {
                n1015 = property on="A1-position-X" class="DigNum (严格)"() -> (error out=w1567:errorcluster, "Value"=w1574:dbl)  [unwired: 2 in, 1 out]
                n1016 = property on="A1-position-Y" class="DigNum (严格)"(error in=w1567) -> (error out=w1566:errorcluster, "Value"=w1563:dbl)  [unwired: 1 in, 1 out]
                n1017 = Subtract(x=w1563, y=18.0) -> (x-y=w1562:dbl)
                n1018 = Subtract(x=w1574, y=4.5) -> (x-y=w1565:dbl)
                n1019 = vi-ref "goto.vi"() -> (w1572:refnum<vi>)
                n1020 = property class="VI"(reference=w1572, error in=w1566) -> ("Name"=w1571:string)  [unwired: 2 out]
                n1021 = Open VI Reference(type specifier VI Refnum (for type only)=refnum<vi> refnum, vi path=w1571, options=128) -> (vi reference=w1569:refnum<vi>)  [unwired: 3 in, 1 out]
                n1022 = call-by-ref "Start Asynchronous Call"(reference=w1569, "Y(mm)"=w1562, "X(mm)"=w1565) -> ()  [unwired: 10 in, 3 out]
              }
            }
            n1023 = property on="currentNO" class="Str"("Value"="E2") -> ()  [unwired: 2 in, 2 out]
          }
          event "E3": Value Change {
            n1024 = event-data() -> ("NewVal"=w1576:bool)  [unwired: 1 in, 5 out]
            n1025 = property on="移动" class="Bool (严格)"() -> ("Value"=w1579:bool)  [unwired: 2 in, 2 out]
            n1026 = Not(x=w1579) -> (.not. x?=w1578:bool)
            n1027 = And(x=w1578, y=w1576) -> (x .and. y?=w1577:bool)
            n1028 = case shown="真" w1577 {
              frame False {
              }
              frame True {
                n1029 = property on="A1-position-X" class="DigNum (严格)"() -> (error out=w1586:errorcluster, "Value"=w1593:dbl)  [unwired: 2 in, 1 out]
                n1030 = property on="A1-position-Y" class="DigNum (严格)"(error in=w1586) -> (error out=w1585:errorcluster, "Value"=w1582:dbl)  [unwired: 1 in, 1 out]
                n1031 = Subtract(x=w1582, y=18.0) -> (x-y=w1581:dbl)
                n1032 = Subtract(x=w1593, y=9) -> (x-y=w1584:dbl)
                n1033 = vi-ref "goto.vi"() -> (w1591:refnum<vi>)
                n1034 = property class="VI"(reference=w1591, error in=w1585) -> ("Name"=w1590:string)  [unwired: 2 out]
                n1035 = Open VI Reference(type specifier VI Refnum (for type only)=refnum<vi> refnum, vi path=w1590, options=128) -> (vi reference=w1588:refnum<vi>)  [unwired: 3 in, 1 out]
                n1036 = call-by-ref "Start Asynchronous Call"(reference=w1588, "Y(mm)"=w1581, "X(mm)"=w1584) -> ()  [unwired: 10 in, 3 out]
              }
            }
            n1037 = property on="currentNO" class="Str"("Value"="E3") -> ()  [unwired: 2 in, 2 out]
          }
          event "E4": Value Change {
            n1038 = event-data() -> ("NewVal"=w1595:bool)  [unwired: 1 in, 5 out]
            n1039 = property on="移动" class="Bool (严格)"() -> ("Value"=w1598:bool)  [unwired: 2 in, 2 out]
            n1040 = Not(x=w1598) -> (.not. x?=w1597:bool)
            n1041 = And(x=w1597, y=w1595) -> (x .and. y?=w1596:bool)
            n1042 = case shown="真" w1596 {
              frame False {
              }
              frame True {
                n1043 = property on="A1-position-X" class="DigNum (严格)"() -> (error out=w1605:errorcluster, "Value"=w1612:dbl)  [unwired: 2 in, 1 out]
                n1044 = property on="A1-position-Y" class="DigNum (严格)"(error in=w1605) -> (error out=w1604:errorcluster, "Value"=w1601:dbl)  [unwired: 1 in, 1 out]
                n1045 = Subtract(x=w1601, y=18.0) -> (x-y=w1600:dbl)
                n1046 = Subtract(x=w1612, y=13.5) -> (x-y=w1603:dbl)
                n1047 = vi-ref "goto.vi"() -> (w1610:refnum<vi>)
                n1048 = property class="VI"(reference=w1610, error in=w1604) -> ("Name"=w1609:string)  [unwired: 2 out]
                n1049 = Open VI Reference(type specifier VI Refnum (for type only)=refnum<vi> refnum, vi path=w1609, options=128) -> (vi reference=w1607:refnum<vi>)  [unwired: 3 in, 1 out]
                n1050 = call-by-ref "Start Asynchronous Call"(reference=w1607, "Y(mm)"=w1600, "X(mm)"=w1603) -> ()  [unwired: 10 in, 3 out]
              }
            }
            n1051 = property on="currentNO" class="Str"("Value"="E4") -> ()  [unwired: 2 in, 2 out]
          }
          event "E5": Value Change {
            n1052 = event-data() -> ("NewVal"=w1614:bool)  [unwired: 1 in, 5 out]
            n1053 = property on="移动" class="Bool (严格)"() -> ("Value"=w1617:bool)  [unwired: 2 in, 2 out]
            n1054 = Not(x=w1617) -> (.not. x?=w1616:bool)
            n1055 = And(x=w1616, y=w1614) -> (x .and. y?=w1615:bool)
            n1056 = case shown="真" w1615 {
              frame False {
              }
              frame True {
                n1057 = property on="A1-position-X" class="DigNum (严格)"() -> (error out=w1624:errorcluster, "Value"=w1631:dbl)  [unwired: 2 in, 1 out]
                n1058 = property on="A1-position-Y" class="DigNum (严格)"(error in=w1624) -> (error out=w1623:errorcluster, "Value"=w1620:dbl)  [unwired: 1 in, 1 out]
                n1059 = Subtract(x=w1620, y=18.0) -> (x-y=w1619:dbl)
                n1060 = Subtract(x=w1631, y=18) -> (x-y=w1622:dbl)
                n1061 = vi-ref "goto.vi"() -> (w1629:refnum<vi>)
                n1062 = property class="VI"(reference=w1629, error in=w1623) -> ("Name"=w1628:string)  [unwired: 2 out]
                n1063 = Open VI Reference(type specifier VI Refnum (for type only)=refnum<vi> refnum, vi path=w1628, options=128) -> (vi reference=w1626:refnum<vi>)  [unwired: 3 in, 1 out]
                n1064 = call-by-ref "Start Asynchronous Call"(reference=w1626, "Y(mm)"=w1619, "X(mm)"=w1622) -> ()  [unwired: 10 in, 3 out]
              }
            }
            n1065 = property on="currentNO" class="Str"("Value"="E5") -> ()  [unwired: 2 in, 2 out]
          }
          event "E6": Value Change {
            n1066 = event-data() -> ("NewVal"=w1633:bool)  [unwired: 1 in, 5 out]
            n1067 = property on="移动" class="Bool (严格)"() -> ("Value"=w1636:bool)  [unwired: 2 in, 2 out]
            n1068 = Not(x=w1636) -> (.not. x?=w1635:bool)
            n1069 = And(x=w1635, y=w1633) -> (x .and. y?=w1634:bool)
            n1070 = case shown="真" w1634 {
              frame False {
              }
              frame True {
                n1071 = property on="A1-position-X" class="DigNum (严格)"() -> (error out=w1643:errorcluster, "Value"=w1650:dbl)  [unwired: 2 in, 1 out]
                n1072 = property on="A1-position-Y" class="DigNum (严格)"(error in=w1643) -> (error out=w1642:errorcluster, "Value"=w1639:dbl)  [unwired: 1 in, 1 out]
                n1073 = Subtract(x=w1639, y=18.0) -> (x-y=w1638:dbl)
                n1074 = Subtract(x=w1650, y=22.5) -> (x-y=w1641:dbl)
                n1075 = vi-ref "goto.vi"() -> (w1648:refnum<vi>)
                n1076 = property class="VI"(reference=w1648, error in=w1642) -> ("Name"=w1647:string)  [unwired: 2 out]
                n1077 = Open VI Reference(type specifier VI Refnum (for type only)=refnum<vi> refnum, vi path=w1647, options=128) -> (vi reference=w1645:refnum<vi>)  [unwired: 3 in, 1 out]
                n1078 = call-by-ref "Start Asynchronous Call"(reference=w1645, "Y(mm)"=w1638, "X(mm)"=w1641) -> ()  [unwired: 10 in, 3 out]
              }
            }
            n1079 = property on="currentNO" class="Str"("Value"="E6") -> ()  [unwired: 2 in, 2 out]
          }
          event "E7": Value Change {
            n1080 = event-data() -> ("NewVal"=w1652:bool)  [unwired: 1 in, 5 out]
            n1081 = property on="移动" class="Bool (严格)"() -> ("Value"=w1655:bool)  [unwired: 2 in, 2 out]
            n1082 = Not(x=w1655) -> (.not. x?=w1654:bool)
            n1083 = And(x=w1654, y=w1652) -> (x .and. y?=w1653:bool)
            n1084 = case shown="真" w1653 {
              frame False {
              }
              frame True {
                n1085 = property on="A1-position-X" class="DigNum (严格)"() -> (error out=w1662:errorcluster, "Value"=w1669:dbl)  [unwired: 2 in, 1 out]
                n1086 = property on="A1-position-Y" class="DigNum (严格)"(error in=w1662) -> (error out=w1661:errorcluster, "Value"=w1658:dbl)  [unwired: 1 in, 1 out]
                n1087 = Subtract(x=w1658, y=18.0) -> (x-y=w1657:dbl)
                n1088 = Subtract(x=w1669, y=27) -> (x-y=w1660:dbl)
                n1089 = vi-ref "goto.vi"() -> (w1667:refnum<vi>)
                n1090 = property class="VI"(reference=w1667, error in=w1661) -> ("Name"=w1666:string)  [unwired: 2 out]
                n1091 = Open VI Reference(type specifier VI Refnum (for type only)=refnum<vi> refnum, vi path=w1666, options=128) -> (vi reference=w1664:refnum<vi>)  [unwired: 3 in, 1 out]
                n1092 = call-by-ref "Start Asynchronous Call"(reference=w1664, "Y(mm)"=w1657, "X(mm)"=w1660) -> ()  [unwired: 10 in, 3 out]
              }
            }
            n1093 = property on="currentNO" class="Str"("Value"="E7") -> ()  [unwired: 2 in, 2 out]
          }
          event "E8": Value Change {
            n1094 = event-data() -> ("NewVal"=w1671:bool)  [unwired: 1 in, 5 out]
            n1095 = property on="移动" class="Bool (严格)"() -> ("Value"=w1674:bool)  [unwired: 2 in, 2 out]
            n1096 = Not(x=w1674) -> (.not. x?=w1673:bool)
            n1097 = And(x=w1673, y=w1671) -> (x .and. y?=w1672:bool)
            n1098 = case shown="真" w1672 {
              frame False {
              }
              frame True {
                n1099 = property on="A1-position-X" class="DigNum (严格)"() -> (error out=w1681:errorcluster, "Value"=w1688:dbl)  [unwired: 2 in, 1 out]
                n1100 = property on="A1-position-Y" class="DigNum (严格)"(error in=w1681) -> (error out=w1680:errorcluster, "Value"=w1677:dbl)  [unwired: 1 in, 1 out]
                n1101 = Subtract(x=w1677, y=18.0) -> (x-y=w1676:dbl)
                n1102 = Subtract(x=w1688, y=31.5) -> (x-y=w1679:dbl)
                n1103 = vi-ref "goto.vi"() -> (w1686:refnum<vi>)
                n1104 = property class="VI"(reference=w1686, error in=w1680) -> ("Name"=w1685:string)  [unwired: 2 out]
                n1105 = Open VI Reference(type specifier VI Refnum (for type only)=refnum<vi> refnum, vi path=w1685, options=128) -> (vi reference=w1683:refnum<vi>)  [unwired: 3 in, 1 out]
                n1106 = call-by-ref "Start Asynchronous Call"(reference=w1683, "Y(mm)"=w1676, "X(mm)"=w1679) -> ()  [unwired: 10 in, 3 out]
              }
            }
            n1107 = property on="currentNO" class="Str"("Value"="E8") -> ()  [unwired: 2 in, 2 out]
          }
          event "E9": Value Change {
            n1108 = event-data() -> ("NewVal"=w1690:bool)  [unwired: 1 in, 5 out]
            n1109 = property on="移动" class="Bool (严格)"() -> ("Value"=w1693:bool)  [unwired: 2 in, 2 out]
            n1110 = Not(x=w1693) -> (.not. x?=w1692:bool)
            n1111 = And(x=w1692, y=w1690) -> (x .and. y?=w1691:bool)
            n1112 = case shown="真" w1691 {
              frame False {
              }
              frame True {
                n1113 = property on="A1-position-X" class="DigNum (严格)"() -> (error out=w1700:errorcluster, "Value"=w1707:dbl)  [unwired: 2 in, 1 out]
                n1114 = property on="A1-position-Y" class="DigNum (严格)"(error in=w1700) -> (error out=w1699:errorcluster, "Value"=w1696:dbl)  [unwired: 1 in, 1 out]
                n1115 = Subtract(x=w1696, y=18.0) -> (x-y=w1695:dbl)
                n1116 = Subtract(x=w1707, y=36.0) -> (x-y=w1698:dbl)
                n1117 = vi-ref "goto.vi"() -> (w1705:refnum<vi>)
                n1118 = property class="VI"(reference=w1705, error in=w1699) -> ("Name"=w1704:string)  [unwired: 2 out]
                n1119 = Open VI Reference(type specifier VI Refnum (for type only)=refnum<vi> refnum, vi path=w1704, options=128) -> (vi reference=w1702:refnum<vi>)  [unwired: 3 in, 1 out]
                n1120 = call-by-ref "Start Asynchronous Call"(reference=w1702, "Y(mm)"=w1695, "X(mm)"=w1698) -> ()  [unwired: 10 in, 3 out]
              }
            }
            n1121 = property on="currentNO" class="Str"("Value"="E9") -> ()  [unwired: 2 in, 2 out]
          }
          event "E10": Value Change {
            n1122 = event-data() -> ("NewVal"=w1709:bool)  [unwired: 1 in, 5 out]
            n1123 = property on="移动" class="Bool (严格)"() -> ("Value"=w1710:bool)  [unwired: 2 in, 2 out]
            n1124 = Not(x=w1710) -> (.not. x?=w1711:bool)
            n1125 = And(x=w1711, y=w1709) -> (x .and. y?=w1712:bool)
            n1126 = case shown="真" w1712 {
              frame False {
              }
              frame True {
                n1127 = property on="A1-position-X" class="DigNum (严格)"() -> (error out=w1719:errorcluster, "Value"=w1726:dbl)  [unwired: 2 in, 1 out]
                n1128 = property on="A1-position-Y" class="DigNum (严格)"(error in=w1719) -> (error out=w1718:errorcluster, "Value"=w1715:dbl)  [unwired: 1 in, 1 out]
                n1129 = Subtract(x=w1715, y=18.0) -> (x-y=w1714:dbl)
                n1130 = Subtract(x=w1726, y=40.5) -> (x-y=w1717:dbl)
                n1131 = vi-ref "goto.vi"() -> (w1724:refnum<vi>)
                n1132 = property class="VI"(reference=w1724, error in=w1718) -> ("Name"=w1723:string)  [unwired: 2 out]
                n1133 = Open VI Reference(type specifier VI Refnum (for type only)=refnum<vi> refnum, vi path=w1723, options=128) -> (vi reference=w1721:refnum<vi>)  [unwired: 3 in, 1 out]
                n1134 = call-by-ref "Start Asynchronous Call"(reference=w1721, "Y(mm)"=w1714, "X(mm)"=w1717) -> ()  [unwired: 10 in, 3 out]
              }
            }
            n1135 = property on="currentNO" class="Str"("Value"="E10") -> ()  [unwired: 2 in, 2 out]
          }
          event "E11": Value Change {
            n1136 = event-data() -> ("NewVal"=w1728:bool)  [unwired: 1 in, 5 out]
            n1137 = property on="移动" class="Bool (严格)"() -> ("Value"=w1731:bool)  [unwired: 2 in, 2 out]
            n1138 = Not(x=w1731) -> (.not. x?=w1730:bool)
            n1139 = And(x=w1730, y=w1728) -> (x .and. y?=w1729:bool)
            n1140 = case shown="真" w1729 {
              frame False {
              }
              frame True {
                n1141 = property on="A1-position-X" class="DigNum (严格)"() -> (error out=w1738:errorcluster, "Value"=w1745:dbl)  [unwired: 2 in, 1 out]
                n1142 = property on="A1-position-Y" class="DigNum (严格)"(error in=w1738) -> (error out=w1737:errorcluster, "Value"=w1734:dbl)  [unwired: 1 in, 1 out]
                n1143 = Subtract(x=w1734, y=18.0) -> (x-y=w1733:dbl)
                n1144 = Subtract(x=w1745, y=45.0) -> (x-y=w1736:dbl)
                n1145 = vi-ref "goto.vi"() -> (w1743:refnum<vi>)
                n1146 = property class="VI"(reference=w1743, error in=w1737) -> ("Name"=w1742:string)  [unwired: 2 out]
                n1147 = Open VI Reference(type specifier VI Refnum (for type only)=refnum<vi> refnum, vi path=w1742, options=128) -> (vi reference=w1740:refnum<vi>)  [unwired: 3 in, 1 out]
                n1148 = call-by-ref "Start Asynchronous Call"(reference=w1740, "Y(mm)"=w1733, "X(mm)"=w1736) -> ()  [unwired: 10 in, 3 out]
              }
            }
            n1149 = property on="currentNO" class="Str"("Value"="E11") -> ()  [unwired: 2 in, 2 out]
          }
          event "E12": Value Change {
            n1150 = event-data() -> ("NewVal"=w1747:bool)  [unwired: 1 in, 5 out]
            n1151 = property on="移动" class="Bool (严格)"() -> ("Value"=w1750:bool)  [unwired: 2 in, 2 out]
            n1152 = Not(x=w1750) -> (.not. x?=w1749:bool)
            n1153 = And(x=w1749, y=w1747) -> (x .and. y?=w1748:bool)
            n1154 = case shown="真" w1748 {
              frame False {
              }
              frame True {
                n1155 = property on="A1-position-X" class="DigNum (严格)"() -> (error out=w1757:errorcluster, "Value"=w1764:dbl)  [unwired: 2 in, 1 out]
                n1156 = property on="A1-position-Y" class="DigNum (严格)"(error in=w1757) -> (error out=w1756:errorcluster, "Value"=w1753:dbl)  [unwired: 1 in, 1 out]
                n1157 = Subtract(x=w1753, y=18.0) -> (x-y=w1752:dbl)
                n1158 = Subtract(x=w1764, y=49.5) -> (x-y=w1755:dbl)
                n1159 = vi-ref "goto.vi"() -> (w1762:refnum<vi>)
                n1160 = property class="VI"(reference=w1762, error in=w1756) -> ("Name"=w1761:string)  [unwired: 2 out]
                n1161 = Open VI Reference(type specifier VI Refnum (for type only)=refnum<vi> refnum, vi path=w1761, options=128) -> (vi reference=w1759:refnum<vi>)  [unwired: 3 in, 1 out]
                n1162 = call-by-ref "Start Asynchronous Call"(reference=w1759, "Y(mm)"=w1752, "X(mm)"=w1755) -> ()  [unwired: 10 in, 3 out]
              }
            }
            n1163 = property on="currentNO" class="Str"("Value"="E12") -> ()  [unwired: 2 in, 2 out]
          }
          event "F1": Value Change {
            n1164 = event-data() -> ("NewVal"=w1766:bool)  [unwired: 1 in, 5 out]
            n1165 = property on="移动" class="Bool (严格)"() -> ("Value"=w1769:bool)  [unwired: 2 in, 2 out]
            n1166 = Not(x=w1769) -> (.not. x?=w1768:bool)
            n1167 = And(x=w1768, y=w1766) -> (x .and. y?=w1767:bool)
            n1168 = case shown="真" w1767 {
              frame False {
              }
              frame True {
                n1169 = property on="A1-position-X" class="DigNum (严格)"() -> (error out=w1776:errorcluster, "Value"=w1783:dbl)  [unwired: 2 in, 1 out]
                n1170 = property on="A1-position-Y" class="DigNum (严格)"(error in=w1776) -> (error out=w1775:errorcluster, "Value"=w1772:dbl)  [unwired: 1 in, 1 out]
                n1171 = Subtract(x=w1772, y=22.5) -> (x-y=w1771:dbl)
                n1172 = Subtract(x=w1783, y=0) -> (x-y=w1774:dbl)
                n1173 = vi-ref "goto.vi"() -> (w1781:refnum<vi>)
                n1174 = property class="VI"(reference=w1781, error in=w1775) -> ("Name"=w1780:string)  [unwired: 2 out]
                n1175 = Open VI Reference(type specifier VI Refnum (for type only)=refnum<vi> refnum, vi path=w1780, options=128) -> (vi reference=w1778:refnum<vi>)  [unwired: 3 in, 1 out]
                n1176 = call-by-ref "Start Asynchronous Call"(reference=w1778, "Y(mm)"=w1771, "X(mm)"=w1774) -> ()  [unwired: 10 in, 3 out]
              }
            }
            n1177 = property on="currentNO" class="Str"("Value"="F1") -> ()  [unwired: 2 in, 2 out]
          }
          event "F2": Value Change {
            n1178 = event-data() -> ("NewVal"=w1785:bool)  [unwired: 1 in, 5 out]
            n1179 = property on="移动" class="Bool (严格)"() -> ("Value"=w1786:bool)  [unwired: 2 in, 2 out]
            n1180 = Not(x=w1786) -> (.not. x?=w1787:bool)
            n1181 = And(x=w1787, y=w1785) -> (x .and. y?=w1788:bool)
            n1182 = case shown="真" w1788 {
              frame False {
              }
              frame True {
                n1183 = property on="A1-position-X" class="DigNum (严格)"() -> (error out=w1795:errorcluster, "Value"=w1802:dbl)  [unwired: 2 in, 1 out]
                n1184 = property on="A1-position-Y" class="DigNum (严格)"(error in=w1795) -> (error out=w1794:errorcluster, "Value"=w1791:dbl)  [unwired: 1 in, 1 out]
                n1185 = Subtract(x=w1791, y=22.5) -> (x-y=w1790:dbl)
                n1186 = Subtract(x=w1802, y=4.5) -> (x-y=w1793:dbl)
                n1187 = vi-ref "goto.vi"() -> (w1800:refnum<vi>)
                n1188 = property class="VI"(reference=w1800, error in=w1794) -> ("Name"=w1799:string)  [unwired: 2 out]
                n1189 = Open VI Reference(type specifier VI Refnum (for type only)=refnum<vi> refnum, vi path=w1799, options=128) -> (vi reference=w1797:refnum<vi>)  [unwired: 3 in, 1 out]
                n1190 = call-by-ref "Start Asynchronous Call"(reference=w1797, "Y(mm)"=w1790, "X(mm)"=w1793) -> ()  [unwired: 10 in, 3 out]
              }
            }
            n1191 = property on="currentNO" class="Str"("Value"="F2") -> ()  [unwired: 2 in, 2 out]
          }
          event "F3": Value Change {
            n1192 = event-data() -> ("NewVal"=w1804:bool)  [unwired: 1 in, 5 out]
            n1193 = property on="移动" class="Bool (严格)"() -> ("Value"=w1805:bool)  [unwired: 2 in, 2 out]
            n1194 = Not(x=w1805) -> (.not. x?=w1806:bool)
            n1195 = And(x=w1806, y=w1804) -> (x .and. y?=w1807:bool)
            n1196 = case shown="真" w1807 {
              frame False {
              }
              frame True {
                n1197 = property on="A1-position-X" class="DigNum (严格)"() -> (error out=w1814:errorcluster, "Value"=w1821:dbl)  [unwired: 2 in, 1 out]
                n1198 = property on="A1-position-Y" class="DigNum (严格)"(error in=w1814) -> (error out=w1813:errorcluster, "Value"=w1810:dbl)  [unwired: 1 in, 1 out]
                n1199 = Subtract(x=w1810, y=22.5) -> (x-y=w1809:dbl)
                n1200 = Subtract(x=w1821, y=9) -> (x-y=w1812:dbl)
                n1201 = vi-ref "goto.vi"() -> (w1819:refnum<vi>)
                n1202 = property class="VI"(reference=w1819, error in=w1813) -> ("Name"=w1818:string)  [unwired: 2 out]
                n1203 = Open VI Reference(type specifier VI Refnum (for type only)=refnum<vi> refnum, vi path=w1818, options=128) -> (vi reference=w1816:refnum<vi>)  [unwired: 3 in, 1 out]
                n1204 = call-by-ref "Start Asynchronous Call"(reference=w1816, "Y(mm)"=w1809, "X(mm)"=w1812) -> ()  [unwired: 10 in, 3 out]
              }
            }
            n1205 = property on="currentNO" class="Str"("Value"="F3") -> ()  [unwired: 2 in, 2 out]
          }
          event "F4": Value Change {
            n1206 = event-data() -> ("NewVal"=w1823:bool)  [unwired: 1 in, 5 out]
            n1207 = property on="移动" class="Bool (严格)"() -> ("Value"=w1826:bool)  [unwired: 2 in, 2 out]
            n1208 = Not(x=w1826) -> (.not. x?=w1825:bool)
            n1209 = And(x=w1825, y=w1823) -> (x .and. y?=w1824:bool)
            n1210 = case shown="真" w1824 {
              frame False {
              }
              frame True {
                n1211 = property on="A1-position-X" class="DigNum (严格)"() -> (error out=w1833:errorcluster, "Value"=w1840:dbl)  [unwired: 2 in, 1 out]
                n1212 = property on="A1-position-Y" class="DigNum (严格)"(error in=w1833) -> (error out=w1832:errorcluster, "Value"=w1829:dbl)  [unwired: 1 in, 1 out]
                n1213 = Subtract(x=w1829, y=22.5) -> (x-y=w1828:dbl)
                n1214 = Subtract(x=w1840, y=13.5) -> (x-y=w1831:dbl)
                n1215 = vi-ref "goto.vi"() -> (w1838:refnum<vi>)
                n1216 = property class="VI"(reference=w1838, error in=w1832) -> ("Name"=w1837:string)  [unwired: 2 out]
                n1217 = Open VI Reference(type specifier VI Refnum (for type only)=refnum<vi> refnum, vi path=w1837, options=128) -> (vi reference=w1835:refnum<vi>)  [unwired: 3 in, 1 out]
                n1218 = call-by-ref "Start Asynchronous Call"(reference=w1835, "Y(mm)"=w1828, "X(mm)"=w1831) -> ()  [unwired: 10 in, 3 out]
              }
            }
            n1219 = property on="currentNO" class="Str"("Value"="F4") -> ()  [unwired: 2 in, 2 out]
          }
          event "F5": Value Change {
            n1220 = event-data() -> ("NewVal"=w1842:bool)  [unwired: 1 in, 5 out]
            n1221 = property on="移动" class="Bool (严格)"() -> ("Value"=w1845:bool)  [unwired: 2 in, 2 out]
            n1222 = Not(x=w1845) -> (.not. x?=w1844:bool)
            n1223 = And(x=w1844, y=w1842) -> (x .and. y?=w1843:bool)
            n1224 = case shown="真" w1843 {
              frame False {
              }
              frame True {
                n1225 = property on="A1-position-X" class="DigNum (严格)"() -> (error out=w1852:errorcluster, "Value"=w1859:dbl)  [unwired: 2 in, 1 out]
                n1226 = property on="A1-position-Y" class="DigNum (严格)"(error in=w1852) -> (error out=w1851:errorcluster, "Value"=w1848:dbl)  [unwired: 1 in, 1 out]
                n1227 = Subtract(x=w1848, y=22.5) -> (x-y=w1847:dbl)
                n1228 = Subtract(x=w1859, y=18.0) -> (x-y=w1850:dbl)
                n1229 = vi-ref "goto.vi"() -> (w1857:refnum<vi>)
                n1230 = property class="VI"(reference=w1857, error in=w1851) -> ("Name"=w1856:string)  [unwired: 2 out]
                n1231 = Open VI Reference(type specifier VI Refnum (for type only)=refnum<vi> refnum, vi path=w1856, options=128) -> (vi reference=w1854:refnum<vi>)  [unwired: 3 in, 1 out]
                n1232 = call-by-ref "Start Asynchronous Call"(reference=w1854, "Y(mm)"=w1847, "X(mm)"=w1850) -> ()  [unwired: 10 in, 3 out]
              }
            }
            n1233 = property on="currentNO" class="Str"("Value"="F5") -> ()  [unwired: 2 in, 2 out]
          }
          event "F6": Value Change {
            n1234 = event-data() -> ("NewVal"=w1861:bool)  [unwired: 1 in, 5 out]
            n1235 = property on="移动" class="Bool (严格)"() -> ("Value"=w1864:bool)  [unwired: 2 in, 2 out]
            n1236 = Not(x=w1864) -> (.not. x?=w1863:bool)
            n1237 = And(x=w1863, y=w1861) -> (x .and. y?=w1862:bool)
            n1238 = case shown="真" w1862 {
              frame False {
              }
              frame True {
                n1239 = property on="A1-position-X" class="DigNum (严格)"() -> (error out=w1871:errorcluster, "Value"=w1878:dbl)  [unwired: 2 in, 1 out]
                n1240 = property on="A1-position-Y" class="DigNum (严格)"(error in=w1871) -> (error out=w1870:errorcluster, "Value"=w1867:dbl)  [unwired: 1 in, 1 out]
                n1241 = Subtract(x=w1867, y=22.5) -> (x-y=w1866:dbl)
                n1242 = Subtract(x=w1878, y=22.5) -> (x-y=w1869:dbl)
                n1243 = vi-ref "goto.vi"() -> (w1876:refnum<vi>)
                n1244 = property class="VI"(reference=w1876, error in=w1870) -> ("Name"=w1875:string)  [unwired: 2 out]
                n1245 = Open VI Reference(type specifier VI Refnum (for type only)=refnum<vi> refnum, vi path=w1875, options=128) -> (vi reference=w1873:refnum<vi>)  [unwired: 3 in, 1 out]
                n1246 = call-by-ref "Start Asynchronous Call"(reference=w1873, "Y(mm)"=w1866, "X(mm)"=w1869) -> ()  [unwired: 10 in, 3 out]
              }
            }
            n1247 = property on="currentNO" class="Str"("Value"="F6") -> ()  [unwired: 2 in, 2 out]
          }
          event "F7": Value Change {
            n1248 = event-data() -> ("NewVal"=w1880:bool)  [unwired: 1 in, 5 out]
            n1249 = property on="移动" class="Bool (严格)"() -> ("Value"=w1883:bool)  [unwired: 2 in, 2 out]
            n1250 = Not(x=w1883) -> (.not. x?=w1882:bool)
            n1251 = And(x=w1882, y=w1880) -> (x .and. y?=w1881:bool)
            n1252 = case shown="真" w1881 {
              frame False {
              }
              frame True {
                n1253 = property on="A1-position-X" class="DigNum (严格)"() -> (error out=w1890:errorcluster, "Value"=w1897:dbl)  [unwired: 2 in, 1 out]
                n1254 = property on="A1-position-Y" class="DigNum (严格)"(error in=w1890) -> (error out=w1889:errorcluster, "Value"=w1886:dbl)  [unwired: 1 in, 1 out]
                n1255 = Subtract(x=w1886, y=22.5) -> (x-y=w1885:dbl)
                n1256 = Subtract(x=w1897, y=27) -> (x-y=w1888:dbl)
                n1257 = vi-ref "goto.vi"() -> (w1895:refnum<vi>)
                n1258 = property class="VI"(reference=w1895, error in=w1889) -> ("Name"=w1894:string)  [unwired: 2 out]
                n1259 = Open VI Reference(type specifier VI Refnum (for type only)=refnum<vi> refnum, vi path=w1894, options=128) -> (vi reference=w1892:refnum<vi>)  [unwired: 3 in, 1 out]
                n1260 = call-by-ref "Start Asynchronous Call"(reference=w1892, "Y(mm)"=w1885, "X(mm)"=w1888) -> ()  [unwired: 10 in, 3 out]
              }
            }
            n1261 = property on="currentNO" class="Str"("Value"="F7") -> ()  [unwired: 2 in, 2 out]
          }
          event "F8": Value Change {
            n1262 = event-data() -> ("NewVal"=w1899:bool)  [unwired: 1 in, 5 out]
            n1263 = property on="移动" class="Bool (严格)"() -> ("Value"=w1902:bool)  [unwired: 2 in, 2 out]
            n1264 = Not(x=w1902) -> (.not. x?=w1901:bool)
            n1265 = And(x=w1901, y=w1899) -> (x .and. y?=w1900:bool)
            n1266 = case shown="真" w1900 {
              frame False {
              }
              frame True {
                n1267 = property on="A1-position-X" class="DigNum (严格)"() -> (error out=w1909:errorcluster, "Value"=w1916:dbl)  [unwired: 2 in, 1 out]
                n1268 = property on="A1-position-Y" class="DigNum (严格)"(error in=w1909) -> (error out=w1908:errorcluster, "Value"=w1905:dbl)  [unwired: 1 in, 1 out]
                n1269 = Subtract(x=w1905, y=22.5) -> (x-y=w1904:dbl)
                n1270 = Subtract(x=w1916, y=31.5) -> (x-y=w1907:dbl)
                n1271 = vi-ref "goto.vi"() -> (w1914:refnum<vi>)
                n1272 = property class="VI"(reference=w1914, error in=w1908) -> ("Name"=w1913:string)  [unwired: 2 out]
                n1273 = Open VI Reference(type specifier VI Refnum (for type only)=refnum<vi> refnum, vi path=w1913, options=128) -> (vi reference=w1911:refnum<vi>)  [unwired: 3 in, 1 out]
                n1274 = call-by-ref "Start Asynchronous Call"(reference=w1911, "Y(mm)"=w1904, "X(mm)"=w1907) -> ()  [unwired: 10 in, 3 out]
              }
            }
            n1275 = property on="currentNO" class="Str"("Value"="F8") -> ()  [unwired: 2 in, 2 out]
          }
          event "F9": Value Change {
            n1276 = event-data() -> ("NewVal"=w1918:bool)  [unwired: 1 in, 5 out]
            n1277 = property on="移动" class="Bool (严格)"() -> ("Value"=w1921:bool)  [unwired: 2 in, 2 out]
            n1278 = Not(x=w1921) -> (.not. x?=w1920:bool)
            n1279 = And(x=w1920, y=w1918) -> (x .and. y?=w1919:bool)
            n1280 = case shown="真" w1919 {
              frame False {
              }
              frame True {
                n1281 = property on="A1-position-X" class="DigNum (严格)"() -> (error out=w1928:errorcluster, "Value"=w1935:dbl)  [unwired: 2 in, 1 out]
                n1282 = property on="A1-position-Y" class="DigNum (严格)"(error in=w1928) -> (error out=w1927:errorcluster, "Value"=w1924:dbl)  [unwired: 1 in, 1 out]
                n1283 = Subtract(x=w1924, y=22.5) -> (x-y=w1923:dbl)
                n1284 = Subtract(x=w1935, y=36) -> (x-y=w1926:dbl)
                n1285 = vi-ref "goto.vi"() -> (w1933:refnum<vi>)
                n1286 = property class="VI"(reference=w1933, error in=w1927) -> ("Name"=w1932:string)  [unwired: 2 out]
                n1287 = Open VI Reference(type specifier VI Refnum (for type only)=refnum<vi> refnum, vi path=w1932, options=128) -> (vi reference=w1930:refnum<vi>)  [unwired: 3 in, 1 out]
                n1288 = call-by-ref "Start Asynchronous Call"(reference=w1930, "Y(mm)"=w1923, "X(mm)"=w1926) -> ()  [unwired: 10 in, 3 out]
              }
            }
            n1289 = property on="currentNO" class="Str"("Value"="F9") -> ()  [unwired: 2 in, 2 out]
          }
          event "F10": Value Change {
            n1290 = event-data() -> ("NewVal"=w1937:bool)  [unwired: 1 in, 5 out]
            n1291 = property on="移动" class="Bool (严格)"() -> ("Value"=w1940:bool)  [unwired: 2 in, 2 out]
            n1292 = Not(x=w1940) -> (.not. x?=w1939:bool)
            n1293 = And(x=w1939, y=w1937) -> (x .and. y?=w1938:bool)
            n1294 = case shown="真" w1938 {
              frame False {
              }
              frame True {
                n1295 = property on="A1-position-X" class="DigNum (严格)"() -> (error out=w1947:errorcluster, "Value"=w1954:dbl)  [unwired: 2 in, 1 out]
                n1296 = property on="A1-position-Y" class="DigNum (严格)"(error in=w1947) -> (error out=w1946:errorcluster, "Value"=w1943:dbl)  [unwired: 1 in, 1 out]
                n1297 = Subtract(x=w1943, y=22.5) -> (x-y=w1942:dbl)
                n1298 = Subtract(x=w1954, y=40.5) -> (x-y=w1945:dbl)
                n1299 = vi-ref "goto.vi"() -> (w1952:refnum<vi>)
                n1300 = property class="VI"(reference=w1952, error in=w1946) -> ("Name"=w1951:string)  [unwired: 2 out]
                n1301 = Open VI Reference(type specifier VI Refnum (for type only)=refnum<vi> refnum, vi path=w1951, options=128) -> (vi reference=w1949:refnum<vi>)  [unwired: 3 in, 1 out]
                n1302 = call-by-ref "Start Asynchronous Call"(reference=w1949, "Y(mm)"=w1942, "X(mm)"=w1945) -> ()  [unwired: 10 in, 3 out]
              }
            }
            n1303 = property on="currentNO" class="Str"("Value"="F10") -> ()  [unwired: 2 in, 2 out]
          }
          event "F11": Value Change {
            n1304 = event-data() -> ("NewVal"=w1956:bool)  [unwired: 1 in, 5 out]
            n1305 = property on="移动" class="Bool (严格)"() -> ("Value"=w1959:bool)  [unwired: 2 in, 2 out]
            n1306 = Not(x=w1959) -> (.not. x?=w1958:bool)
            n1307 = And(x=w1958, y=w1956) -> (x .and. y?=w1957:bool)
            n1308 = case shown="真" w1957 {
              frame False {
              }
              frame True {
                n1309 = property on="A1-position-X" class="DigNum (严格)"() -> (error out=w1966:errorcluster, "Value"=w1973:dbl)  [unwired: 2 in, 1 out]
                n1310 = property on="A1-position-Y" class="DigNum (严格)"(error in=w1966) -> (error out=w1965:errorcluster, "Value"=w1962:dbl)  [unwired: 1 in, 1 out]
                n1311 = Subtract(x=w1962, y=22.5) -> (x-y=w1961:dbl)
                n1312 = Subtract(x=w1973, y=45) -> (x-y=w1964:dbl)
                n1313 = vi-ref "goto.vi"() -> (w1971:refnum<vi>)
                n1314 = property class="VI"(reference=w1971, error in=w1965) -> ("Name"=w1970:string)  [unwired: 2 out]
                n1315 = Open VI Reference(type specifier VI Refnum (for type only)=refnum<vi> refnum, vi path=w1970, options=128) -> (vi reference=w1968:refnum<vi>)  [unwired: 3 in, 1 out]
                n1316 = call-by-ref "Start Asynchronous Call"(reference=w1968, "Y(mm)"=w1961, "X(mm)"=w1964) -> ()  [unwired: 10 in, 3 out]
              }
            }
            n1317 = property on="currentNO" class="Str"("Value"="F11") -> ()  [unwired: 2 in, 2 out]
          }
          event "F12": Value Change {
            n1318 = event-data() -> ("NewVal"=w1975:bool)  [unwired: 1 in, 5 out]
            n1319 = property on="移动" class="Bool (严格)"() -> ("Value"=w1978:bool)  [unwired: 2 in, 2 out]
            n1320 = Not(x=w1978) -> (.not. x?=w1977:bool)
            n1321 = And(x=w1977, y=w1975) -> (x .and. y?=w1976:bool)
            n1322 = case shown="真" w1976 {
              frame False {
              }
              frame True {
                n1323 = property on="A1-position-X" class="DigNum (严格)"() -> (error out=w1985:errorcluster, "Value"=w1992:dbl)  [unwired: 2 in, 1 out]
                n1324 = property on="A1-position-Y" class="DigNum (严格)"(error in=w1985) -> (error out=w1984:errorcluster, "Value"=w1981:dbl)  [unwired: 1 in, 1 out]
                n1325 = Subtract(x=w1981, y=22.5) -> (x-y=w1980:dbl)
                n1326 = Subtract(x=w1992, y=49.5) -> (x-y=w1983:dbl)
                n1327 = vi-ref "goto.vi"() -> (w1990:refnum<vi>)
                n1328 = property class="VI"(reference=w1990, error in=w1984) -> ("Name"=w1989:string)  [unwired: 2 out]
                n1329 = Open VI Reference(type specifier VI Refnum (for type only)=refnum<vi> refnum, vi path=w1989, options=128) -> (vi reference=w1987:refnum<vi>)  [unwired: 3 in, 1 out]
                n1330 = call-by-ref "Start Asynchronous Call"(reference=w1987, "Y(mm)"=w1980, "X(mm)"=w1983) -> ()  [unwired: 10 in, 3 out]
              }
            }
            n1331 = property on="currentNO" class="Str"("Value"="F12") -> ()  [unwired: 2 in, 2 out]
          }
          event "G1": Value Change {
            n1332 = event-data() -> ("NewVal"=w1994:bool)  [unwired: 1 in, 5 out]
            n1333 = property on="移动" class="Bool (严格)"() -> ("Value"=w1997:bool)  [unwired: 2 in, 2 out]
            n1334 = Not(x=w1997) -> (.not. x?=w1996:bool)
            n1335 = And(x=w1996, y=w1994) -> (x .and. y?=w1995:bool)
            n1336 = case shown="真" w1995 {
              frame False {
              }
              frame True {
                n1337 = property on="A1-position-X" class="DigNum (严格)"() -> (error out=w2004:errorcluster, "Value"=w2011:dbl)  [unwired: 2 in, 1 out]
                n1338 = property on="A1-position-Y" class="DigNum (严格)"(error in=w2004) -> (error out=w2003:errorcluster, "Value"=w2000:dbl)  [unwired: 1 in, 1 out]
                n1339 = Subtract(x=w2000, y=27.0) -> (x-y=w1999:dbl)
                n1340 = Subtract(x=w2011, y=0) -> (x-y=w2002:dbl)
                n1341 = vi-ref "goto.vi"() -> (w2009:refnum<vi>)
                n1342 = property class="VI"(reference=w2009, error in=w2003) -> ("Name"=w2008:string)  [unwired: 2 out]
                n1343 = Open VI Reference(type specifier VI Refnum (for type only)=refnum<vi> refnum, vi path=w2008, options=128) -> (vi reference=w2006:refnum<vi>)  [unwired: 3 in, 1 out]
                n1344 = call-by-ref "Start Asynchronous Call"(reference=w2006, "Y(mm)"=w1999, "X(mm)"=w2002) -> ()  [unwired: 10 in, 3 out]
              }
            }
            n1345 = property on="currentNO" class="Str"("Value"="G1") -> ()  [unwired: 2 in, 2 out]
          }
          event "G2": Value Change {
            n1346 = event-data() -> ("NewVal"=w2013:bool)  [unwired: 1 in, 5 out]
            n1347 = property on="移动" class="Bool (严格)"() -> ("Value"=w2016:bool)  [unwired: 2 in, 2 out]
            n1348 = Not(x=w2016) -> (.not. x?=w2015:bool)
            n1349 = And(x=w2015, y=w2013) -> (x .and. y?=w2014:bool)
            n1350 = case shown="真" w2014 {
              frame False {
              }
              frame True {
                n1351 = property on="A1-position-X" class="DigNum (严格)"() -> (error out=w2023:errorcluster, "Value"=w2030:dbl)  [unwired: 2 in, 1 out]
                n1352 = property on="A1-position-Y" class="DigNum (严格)"(error in=w2023) -> (error out=w2022:errorcluster, "Value"=w2019:dbl)  [unwired: 1 in, 1 out]
                n1353 = Subtract(x=w2019, y=27.0) -> (x-y=w2018:dbl)
                n1354 = Subtract(x=w2030, y=4.5) -> (x-y=w2021:dbl)
                n1355 = vi-ref "goto.vi"() -> (w2028:refnum<vi>)
                n1356 = property class="VI"(reference=w2028, error in=w2022) -> ("Name"=w2027:string)  [unwired: 2 out]
                n1357 = Open VI Reference(type specifier VI Refnum (for type only)=refnum<vi> refnum, vi path=w2027, options=128) -> (vi reference=w2025:refnum<vi>)  [unwired: 3 in, 1 out]
                n1358 = call-by-ref "Start Asynchronous Call"(reference=w2025, "Y(mm)"=w2018, "X(mm)"=w2021) -> ()  [unwired: 10 in, 3 out]
              }
            }
            n1359 = property on="currentNO" class="Str"("Value"="G2") -> ()  [unwired: 2 in, 2 out]
          }
          event "G3": Value Change {
            n1360 = event-data() -> ("NewVal"=w2032:bool)  [unwired: 1 in, 5 out]
            n1361 = property on="移动" class="Bool (严格)"() -> ("Value"=w2035:bool)  [unwired: 2 in, 2 out]
            n1362 = Not(x=w2035) -> (.not. x?=w2034:bool)
            n1363 = And(x=w2034, y=w2032) -> (x .and. y?=w2033:bool)
            n1364 = case shown="真" w2033 {
              frame False {
              }
              frame True {
                n1365 = property on="A1-position-X" class="DigNum (严格)"() -> (error out=w2042:errorcluster, "Value"=w2049:dbl)  [unwired: 2 in, 1 out]
                n1366 = property on="A1-position-Y" class="DigNum (严格)"(error in=w2042) -> (error out=w2041:errorcluster, "Value"=w2038:dbl)  [unwired: 1 in, 1 out]
                n1367 = Subtract(x=w2038, y=27.0) -> (x-y=w2037:dbl)
                n1368 = Subtract(x=w2049, y=9.0) -> (x-y=w2040:dbl)
                n1369 = vi-ref "goto.vi"() -> (w2047:refnum<vi>)
                n1370 = property class="VI"(reference=w2047, error in=w2041) -> ("Name"=w2046:string)  [unwired: 2 out]
                n1371 = Open VI Reference(type specifier VI Refnum (for type only)=refnum<vi> refnum, vi path=w2046, options=128) -> (vi reference=w2044:refnum<vi>)  [unwired: 3 in, 1 out]
                n1372 = call-by-ref "Start Asynchronous Call"(reference=w2044, "Y(mm)"=w2037, "X(mm)"=w2040) -> ()  [unwired: 10 in, 3 out]
              }
            }
            n1373 = property on="currentNO" class="Str"("Value"="G3") -> ()  [unwired: 2 in, 2 out]
          }
          event "G4": Value Change {
            n1374 = event-data() -> ("NewVal"=w2051:bool)  [unwired: 1 in, 5 out]
            n1375 = property on="移动" class="Bool (严格)"() -> ("Value"=w2054:bool)  [unwired: 2 in, 2 out]
            n1376 = Not(x=w2054) -> (.not. x?=w2053:bool)
            n1377 = And(x=w2053, y=w2051) -> (x .and. y?=w2052:bool)
            n1378 = case shown="真" w2052 {
              frame False {
              }
              frame True {
                n1379 = property on="A1-position-X" class="DigNum (严格)"() -> (error out=w2061:errorcluster, "Value"=w2068:dbl)  [unwired: 2 in, 1 out]
                n1380 = property on="A1-position-Y" class="DigNum (严格)"(error in=w2061) -> (error out=w2060:errorcluster, "Value"=w2057:dbl)  [unwired: 1 in, 1 out]
                n1381 = Subtract(x=w2057, y=27.0) -> (x-y=w2056:dbl)
                n1382 = Subtract(x=w2068, y=13.5) -> (x-y=w2059:dbl)
                n1383 = vi-ref "goto.vi"() -> (w2066:refnum<vi>)
                n1384 = property class="VI"(reference=w2066, error in=w2060) -> ("Name"=w2065:string)  [unwired: 2 out]
                n1385 = Open VI Reference(type specifier VI Refnum (for type only)=refnum<vi> refnum, vi path=w2065, options=128) -> (vi reference=w2063:refnum<vi>)  [unwired: 3 in, 1 out]
                n1386 = call-by-ref "Start Asynchronous Call"(reference=w2063, "Y(mm)"=w2056, "X(mm)"=w2059) -> ()  [unwired: 10 in, 3 out]
              }
            }
            n1387 = property on="currentNO" class="Str"("Value"="G4") -> ()  [unwired: 2 in, 2 out]
          }
          event "G5": Value Change {
            n1388 = event-data() -> ("NewVal"=w2070:bool)  [unwired: 1 in, 5 out]
            n1389 = property on="移动" class="Bool (严格)"() -> ("Value"=w2073:bool)  [unwired: 2 in, 2 out]
            n1390 = Not(x=w2073) -> (.not. x?=w2072:bool)
            n1391 = And(x=w2072, y=w2070) -> (x .and. y?=w2071:bool)
            n1392 = case shown="真" w2071 {
              frame False {
              }
              frame True {
                n1393 = property on="A1-position-X" class="DigNum (严格)"() -> (error out=w2080:errorcluster, "Value"=w2087:dbl)  [unwired: 2 in, 1 out]
                n1394 = property on="A1-position-Y" class="DigNum (严格)"(error in=w2080) -> (error out=w2079:errorcluster, "Value"=w2076:dbl)  [unwired: 1 in, 1 out]
                n1395 = Subtract(x=w2076, y=27.0) -> (x-y=w2075:dbl)
                n1396 = Subtract(x=w2087, y=18) -> (x-y=w2078:dbl)
                n1397 = vi-ref "goto.vi"() -> (w2085:refnum<vi>)
                n1398 = property class="VI"(reference=w2085, error in=w2079) -> ("Name"=w2084:string)  [unwired: 2 out]
                n1399 = Open VI Reference(type specifier VI Refnum (for type only)=refnum<vi> refnum, vi path=w2084, options=128) -> (vi reference=w2082:refnum<vi>)  [unwired: 3 in, 1 out]
                n1400 = call-by-ref "Start Asynchronous Call"(reference=w2082, "Y(mm)"=w2075, "X(mm)"=w2078) -> ()  [unwired: 10 in, 3 out]
              }
            }
            n1401 = property on="currentNO" class="Str"("Value"="G5") -> ()  [unwired: 2 in, 2 out]
          }
          event "G6": Value Change {
            n1402 = event-data() -> ("NewVal"=w2089:bool)  [unwired: 1 in, 5 out]
            n1403 = property on="移动" class="Bool (严格)"() -> ("Value"=w2092:bool)  [unwired: 2 in, 2 out]
            n1404 = Not(x=w2092) -> (.not. x?=w2091:bool)
            n1405 = And(x=w2091, y=w2089) -> (x .and. y?=w2090:bool)
            n1406 = case shown="真" w2090 {
              frame False {
              }
              frame True {
                n1407 = property on="A1-position-X" class="DigNum (严格)"() -> (error out=w2099:errorcluster, "Value"=w2106:dbl)  [unwired: 2 in, 1 out]
                n1408 = property on="A1-position-Y" class="DigNum (严格)"(error in=w2099) -> (error out=w2098:errorcluster, "Value"=w2095:dbl)  [unwired: 1 in, 1 out]
                n1409 = Subtract(x=w2095, y=27.0) -> (x-y=w2094:dbl)
                n1410 = Subtract(x=w2106, y=22.5) -> (x-y=w2097:dbl)
                n1411 = vi-ref "goto.vi"() -> (w2104:refnum<vi>)
                n1412 = property class="VI"(reference=w2104, error in=w2098) -> ("Name"=w2103:string)  [unwired: 2 out]
                n1413 = Open VI Reference(type specifier VI Refnum (for type only)=refnum<vi> refnum, vi path=w2103, options=128) -> (vi reference=w2101:refnum<vi>)  [unwired: 3 in, 1 out]
                n1414 = call-by-ref "Start Asynchronous Call"(reference=w2101, "Y(mm)"=w2094, "X(mm)"=w2097) -> ()  [unwired: 10 in, 3 out]
              }
            }
            n1415 = property on="currentNO" class="Str"("Value"="G6") -> ()  [unwired: 2 in, 2 out]
          }
          event "G7": Value Change {
            n1416 = event-data() -> ("NewVal"=w2108:bool)  [unwired: 1 in, 5 out]
            n1417 = property on="移动" class="Bool (严格)"() -> ("Value"=w2111:bool)  [unwired: 2 in, 2 out]
            n1418 = Not(x=w2111) -> (.not. x?=w2110:bool)
            n1419 = And(x=w2110, y=w2108) -> (x .and. y?=w2109:bool)
            n1420 = case shown="真" w2109 {
              frame False {
              }
              frame True {
                n1421 = property on="A1-position-X" class="DigNum (严格)"() -> (error out=w2118:errorcluster, "Value"=w2125:dbl)  [unwired: 2 in, 1 out]
                n1422 = property on="A1-position-Y" class="DigNum (严格)"(error in=w2118) -> (error out=w2117:errorcluster, "Value"=w2114:dbl)  [unwired: 1 in, 1 out]
                n1423 = Subtract(x=w2114, y=27.0) -> (x-y=w2113:dbl)
                n1424 = Subtract(x=w2125, y=27) -> (x-y=w2116:dbl)
                n1425 = vi-ref "goto.vi"() -> (w2123:refnum<vi>)
                n1426 = property class="VI"(reference=w2123, error in=w2117) -> ("Name"=w2122:string)  [unwired: 2 out]
                n1427 = Open VI Reference(type specifier VI Refnum (for type only)=refnum<vi> refnum, vi path=w2122, options=128) -> (vi reference=w2120:refnum<vi>)  [unwired: 3 in, 1 out]
                n1428 = call-by-ref "Start Asynchronous Call"(reference=w2120, "Y(mm)"=w2113, "X(mm)"=w2116) -> ()  [unwired: 10 in, 3 out]
              }
            }
            n1429 = property on="currentNO" class="Str"("Value"="G7") -> ()  [unwired: 2 in, 2 out]
          }
          event "G8": Value Change {
            n1430 = event-data() -> ("NewVal"=w2127:bool)  [unwired: 1 in, 5 out]
            n1431 = property on="移动" class="Bool (严格)"() -> ("Value"=w2130:bool)  [unwired: 2 in, 2 out]
            n1432 = Not(x=w2130) -> (.not. x?=w2129:bool)
            n1433 = And(x=w2129, y=w2127) -> (x .and. y?=w2128:bool)
            n1434 = case shown="真" w2128 {
              frame False {
              }
              frame True {
                n1435 = property on="A1-position-X" class="DigNum (严格)"() -> (error out=w2137:errorcluster, "Value"=w2144:dbl)  [unwired: 2 in, 1 out]
                n1436 = property on="A1-position-Y" class="DigNum (严格)"(error in=w2137) -> (error out=w2136:errorcluster, "Value"=w2133:dbl)  [unwired: 1 in, 1 out]
                n1437 = Subtract(x=w2133, y=27.0) -> (x-y=w2132:dbl)
                n1438 = Subtract(x=w2144, y=31.5) -> (x-y=w2135:dbl)
                n1439 = vi-ref "goto.vi"() -> (w2142:refnum<vi>)
                n1440 = property class="VI"(reference=w2142, error in=w2136) -> ("Name"=w2141:string)  [unwired: 2 out]
                n1441 = Open VI Reference(type specifier VI Refnum (for type only)=refnum<vi> refnum, vi path=w2141, options=128) -> (vi reference=w2139:refnum<vi>)  [unwired: 3 in, 1 out]
                n1442 = call-by-ref "Start Asynchronous Call"(reference=w2139, "Y(mm)"=w2132, "X(mm)"=w2135) -> ()  [unwired: 10 in, 3 out]
              }
            }
            n1443 = property on="currentNO" class="Str"("Value"="G8") -> ()  [unwired: 2 in, 2 out]
          }
          event "G9": Value Change {
            n1444 = event-data() -> ("NewVal"=w2146:bool)  [unwired: 1 in, 5 out]
            n1445 = property on="移动" class="Bool (严格)"() -> ("Value"=w2149:bool)  [unwired: 2 in, 2 out]
            n1446 = Not(x=w2149) -> (.not. x?=w2148:bool)
            n1447 = And(x=w2148, y=w2146) -> (x .and. y?=w2147:bool)
            n1448 = case shown="真" w2147 {
              frame False {
              }
              frame True {
                n1449 = property on="A1-position-X" class="DigNum (严格)"() -> (error out=w2156:errorcluster, "Value"=w2163:dbl)  [unwired: 2 in, 1 out]
                n1450 = property on="A1-position-Y" class="DigNum (严格)"(error in=w2156) -> (error out=w2155:errorcluster, "Value"=w2152:dbl)  [unwired: 1 in, 1 out]
                n1451 = Subtract(x=w2152, y=27.0) -> (x-y=w2151:dbl)
                n1452 = Subtract(x=w2163, y=36.0) -> (x-y=w2154:dbl)
                n1453 = vi-ref "goto.vi"() -> (w2161:refnum<vi>)
                n1454 = property class="VI"(reference=w2161, error in=w2155) -> ("Name"=w2160:string)  [unwired: 2 out]
                n1455 = Open VI Reference(type specifier VI Refnum (for type only)=refnum<vi> refnum, vi path=w2160, options=128) -> (vi reference=w2158:refnum<vi>)  [unwired: 3 in, 1 out]
                n1456 = call-by-ref "Start Asynchronous Call"(reference=w2158, "Y(mm)"=w2151, "X(mm)"=w2154) -> ()  [unwired: 10 in, 3 out]
              }
            }
            n1457 = property on="currentNO" class="Str"("Value"="G9") -> ()  [unwired: 2 in, 2 out]
          }
          event "G10": Value Change {
            n1458 = event-data() -> ("NewVal"=w2165:bool)  [unwired: 1 in, 5 out]
            n1459 = property on="移动" class="Bool (严格)"() -> ("Value"=w2168:bool)  [unwired: 2 in, 2 out]
            n1460 = Not(x=w2168) -> (.not. x?=w2167:bool)
            n1461 = And(x=w2167, y=w2165) -> (x .and. y?=w2166:bool)
            n1462 = case shown="真" w2166 {
              frame False {
              }
              frame True {
                n1463 = property on="A1-position-X" class="DigNum (严格)"() -> (error out=w2175:errorcluster, "Value"=w2182:dbl)  [unwired: 2 in, 1 out]
                n1464 = property on="A1-position-Y" class="DigNum (严格)"(error in=w2175) -> (error out=w2174:errorcluster, "Value"=w2171:dbl)  [unwired: 1 in, 1 out]
                n1465 = Subtract(x=w2171, y=27.0) -> (x-y=w2170:dbl)
                n1466 = Subtract(x=w2182, y=40.5) -> (x-y=w2173:dbl)
                n1467 = vi-ref "goto.vi"() -> (w2180:refnum<vi>)
                n1468 = property class="VI"(reference=w2180, error in=w2174) -> ("Name"=w2179:string)  [unwired: 2 out]
                n1469 = Open VI Reference(type specifier VI Refnum (for type only)=refnum<vi> refnum, vi path=w2179, options=128) -> (vi reference=w2177:refnum<vi>)  [unwired: 3 in, 1 out]
                n1470 = call-by-ref "Start Asynchronous Call"(reference=w2177, "Y(mm)"=w2170, "X(mm)"=w2173) -> ()  [unwired: 10 in, 3 out]
              }
            }
            n1471 = property on="currentNO" class="Str"("Value"="G10") -> ()  [unwired: 2 in, 2 out]
          }
          event "G11": Value Change {
            n1472 = event-data() -> ("NewVal"=w2184:bool)  [unwired: 1 in, 5 out]
            n1473 = property on="移动" class="Bool (严格)"() -> ("Value"=w2187:bool)  [unwired: 2 in, 2 out]
            n1474 = Not(x=w2187) -> (.not. x?=w2186:bool)
            n1475 = And(x=w2186, y=w2184) -> (x .and. y?=w2185:bool)
            n1476 = case shown="真" w2185 {
              frame False {
              }
              frame True {
                n1477 = property on="A1-position-X" class="DigNum (严格)"() -> (error out=w2194:errorcluster, "Value"=w2201:dbl)  [unwired: 2 in, 1 out]
                n1478 = property on="A1-position-Y" class="DigNum (严格)"(error in=w2194) -> (error out=w2193:errorcluster, "Value"=w2190:dbl)  [unwired: 1 in, 1 out]
                n1479 = Subtract(x=w2190, y=27.0) -> (x-y=w2189:dbl)
                n1480 = Subtract(x=w2201, y=45) -> (x-y=w2192:dbl)
                n1481 = vi-ref "goto.vi"() -> (w2199:refnum<vi>)
                n1482 = property class="VI"(reference=w2199, error in=w2193) -> ("Name"=w2198:string)  [unwired: 2 out]
                n1483 = Open VI Reference(type specifier VI Refnum (for type only)=refnum<vi> refnum, vi path=w2198, options=128) -> (vi reference=w2196:refnum<vi>)  [unwired: 3 in, 1 out]
                n1484 = call-by-ref "Start Asynchronous Call"(reference=w2196, "Y(mm)"=w2189, "X(mm)"=w2192) -> ()  [unwired: 10 in, 3 out]
              }
            }
            n1485 = property on="currentNO" class="Str"("Value"="G11") -> ()  [unwired: 2 in, 2 out]
          }
          event "G12": Value Change {
            n1486 = event-data() -> ("NewVal"=w2203:bool)  [unwired: 1 in, 5 out]
            n1487 = property on="移动" class="Bool (严格)"() -> ("Value"=w2206:bool)  [unwired: 2 in, 2 out]
            n1488 = Not(x=w2206) -> (.not. x?=w2205:bool)
            n1489 = And(x=w2205, y=w2203) -> (x .and. y?=w2204:bool)
            n1490 = case shown="真" w2204 {
              frame False {
              }
              frame True {
                n1491 = property on="A1-position-X" class="DigNum (严格)"() -> (error out=w2213:errorcluster, "Value"=w2220:dbl)  [unwired: 2 in, 1 out]
                n1492 = property on="A1-position-Y" class="DigNum (严格)"(error in=w2213) -> (error out=w2212:errorcluster, "Value"=w2209:dbl)  [unwired: 1 in, 1 out]
                n1493 = Subtract(x=w2209, y=27.0) -> (x-y=w2208:dbl)
                n1494 = Subtract(x=w2220, y=49.5) -> (x-y=w2211:dbl)
                n1495 = vi-ref "goto.vi"() -> (w2218:refnum<vi>)
                n1496 = property class="VI"(reference=w2218, error in=w2212) -> ("Name"=w2217:string)  [unwired: 2 out]
                n1497 = Open VI Reference(type specifier VI Refnum (for type only)=refnum<vi> refnum, vi path=w2217, options=128) -> (vi reference=w2215:refnum<vi>)  [unwired: 3 in, 1 out]
                n1498 = call-by-ref "Start Asynchronous Call"(reference=w2215, "Y(mm)"=w2208, "X(mm)"=w2211) -> ()  [unwired: 10 in, 3 out]
              }
            }
            n1499 = property on="currentNO" class="Str"("Value"="G12") -> ()  [unwired: 2 in, 2 out]
          }
          event "H1": Value Change {
            n1500 = event-data() -> ("NewVal"=w2222:bool)  [unwired: 1 in, 5 out]
            n1501 = property on="移动" class="Bool (严格)"() -> ("Value"=w2225:bool)  [unwired: 2 in, 2 out]
            n1502 = Not(x=w2225) -> (.not. x?=w2224:bool)
            n1503 = And(x=w2224, y=w2222) -> (x .and. y?=w2223:bool)
            n1504 = case shown="真" w2223 {
              frame False {
              }
              frame True {
                n1505 = property on="A1-position-X" class="DigNum (严格)"() -> (error out=w2232:errorcluster, "Value"=w2239:dbl)  [unwired: 2 in, 1 out]
                n1506 = property on="A1-position-Y" class="DigNum (严格)"(error in=w2232) -> (error out=w2231:errorcluster, "Value"=w2228:dbl)  [unwired: 1 in, 1 out]
                n1507 = Subtract(x=w2228, y=31.5) -> (x-y=w2227:dbl)
                n1508 = Subtract(x=w2239, y=0) -> (x-y=w2230:dbl)
                n1509 = vi-ref "goto.vi"() -> (w2237:refnum<vi>)
                n1510 = property class="VI"(reference=w2237, error in=w2231) -> ("Name"=w2236:string)  [unwired: 2 out]
                n1511 = Open VI Reference(type specifier VI Refnum (for type only)=refnum<vi> refnum, vi path=w2236, options=128) -> (vi reference=w2234:refnum<vi>)  [unwired: 3 in, 1 out]
                n1512 = call-by-ref "Start Asynchronous Call"(reference=w2234, "Y(mm)"=w2227, "X(mm)"=w2230) -> ()  [unwired: 10 in, 3 out]
              }
            }
            n1513 = property on="currentNO" class="Str"("Value"="H1") -> ()  [unwired: 2 in, 2 out]
          }
          event "H2": Value Change {
            n1514 = event-data() -> ("NewVal"=w2241:bool)  [unwired: 1 in, 5 out]
            n1515 = property on="移动" class="Bool (严格)"() -> ("Value"=w2244:bool)  [unwired: 2 in, 2 out]
            n1516 = Not(x=w2244) -> (.not. x?=w2243:bool)
            n1517 = And(x=w2243, y=w2241) -> (x .and. y?=w2242:bool)
            n1518 = case shown="真" w2242 {
              frame False {
              }
              frame True {
                n1519 = property on="A1-position-X" class="DigNum (严格)"() -> (error out=w2251:errorcluster, "Value"=w2258:dbl)  [unwired: 2 in, 1 out]
                n1520 = property on="A1-position-Y" class="DigNum (严格)"(error in=w2251) -> (error out=w2250:errorcluster, "Value"=w2247:dbl)  [unwired: 1 in, 1 out]
                n1521 = Subtract(x=w2247, y=31.5) -> (x-y=w2246:dbl)
                n1522 = Subtract(x=w2258, y=4.5) -> (x-y=w2249:dbl)
                n1523 = vi-ref "goto.vi"() -> (w2256:refnum<vi>)
                n1524 = property class="VI"(reference=w2256, error in=w2250) -> ("Name"=w2255:string)  [unwired: 2 out]
                n1525 = Open VI Reference(type specifier VI Refnum (for type only)=refnum<vi> refnum, vi path=w2255, options=128) -> (vi reference=w2253:refnum<vi>)  [unwired: 3 in, 1 out]
                n1526 = call-by-ref "Start Asynchronous Call"(reference=w2253, "Y(mm)"=w2246, "X(mm)"=w2249) -> ()  [unwired: 10 in, 3 out]
              }
            }
            n1527 = property on="currentNO" class="Str"("Value"="H2") -> ()  [unwired: 2 in, 2 out]
          }
          event "H3": Value Change {
            n1528 = event-data() -> ("NewVal"=w2260:bool)  [unwired: 1 in, 5 out]
            n1529 = property on="移动" class="Bool (严格)"() -> ("Value"=w2263:bool)  [unwired: 2 in, 2 out]
            n1530 = Not(x=w2263) -> (.not. x?=w2262:bool)
            n1531 = And(x=w2262, y=w2260) -> (x .and. y?=w2261:bool)
            n1532 = case shown="真" w2261 {
              frame False {
              }
              frame True {
                n1533 = property on="A1-position-X" class="DigNum (严格)"() -> (error out=w2270:errorcluster, "Value"=w2277:dbl)  [unwired: 2 in, 1 out]
                n1534 = property on="A1-position-Y" class="DigNum (严格)"(error in=w2270) -> (error out=w2269:errorcluster, "Value"=w2266:dbl)  [unwired: 1 in, 1 out]
                n1535 = Subtract(x=w2266, y=31.5) -> (x-y=w2265:dbl)
                n1536 = Subtract(x=w2277, y=9.0) -> (x-y=w2268:dbl)
                n1537 = vi-ref "goto.vi"() -> (w2275:refnum<vi>)
                n1538 = property class="VI"(reference=w2275, error in=w2269) -> ("Name"=w2274:string)  [unwired: 2 out]
                n1539 = Open VI Reference(type specifier VI Refnum (for type only)=refnum<vi> refnum, vi path=w2274, options=128) -> (vi reference=w2272:refnum<vi>)  [unwired: 3 in, 1 out]
                n1540 = call-by-ref "Start Asynchronous Call"(reference=w2272, "Y(mm)"=w2265, "X(mm)"=w2268) -> ()  [unwired: 10 in, 3 out]
              }
            }
            n1541 = property on="currentNO" class="Str"("Value"="H3") -> ()  [unwired: 2 in, 2 out]
          }
          event "H4": Value Change {
            n1542 = event-data() -> ("NewVal"=w2279:bool)  [unwired: 1 in, 5 out]
            n1543 = property on="移动" class="Bool (严格)"() -> ("Value"=w2282:bool)  [unwired: 2 in, 2 out]
            n1544 = Not(x=w2282) -> (.not. x?=w2281:bool)
            n1545 = And(x=w2281, y=w2279) -> (x .and. y?=w2280:bool)
            n1546 = case shown="真" w2280 {
              frame False {
              }
              frame True {
                n1547 = property on="A1-position-X" class="DigNum (严格)"() -> (error out=w2289:errorcluster, "Value"=w2296:dbl)  [unwired: 2 in, 1 out]
                n1548 = property on="A1-position-Y" class="DigNum (严格)"(error in=w2289) -> (error out=w2288:errorcluster, "Value"=w2285:dbl)  [unwired: 1 in, 1 out]
                n1549 = Subtract(x=w2285, y=31.5) -> (x-y=w2284:dbl)
                n1550 = Subtract(x=w2296, y=13.5) -> (x-y=w2287:dbl)
                n1551 = vi-ref "goto.vi"() -> (w2294:refnum<vi>)
                n1552 = property class="VI"(reference=w2294, error in=w2288) -> ("Name"=w2293:string)  [unwired: 2 out]
                n1553 = Open VI Reference(type specifier VI Refnum (for type only)=refnum<vi> refnum, vi path=w2293, options=128) -> (vi reference=w2291:refnum<vi>)  [unwired: 3 in, 1 out]
                n1554 = call-by-ref "Start Asynchronous Call"(reference=w2291, "Y(mm)"=w2284, "X(mm)"=w2287) -> ()  [unwired: 10 in, 3 out]
              }
            }
            n1555 = property on="currentNO" class="Str"("Value"="H4") -> ()  [unwired: 2 in, 2 out]
          }
          event "H5": Value Change {
            n1556 = event-data() -> ("NewVal"=w2298:bool)  [unwired: 1 in, 5 out]
            n1557 = property on="移动" class="Bool (严格)"() -> ("Value"=w2301:bool)  [unwired: 2 in, 2 out]
            n1558 = Not(x=w2301) -> (.not. x?=w2300:bool)
            n1559 = And(x=w2300, y=w2298) -> (x .and. y?=w2299:bool)
            n1560 = case shown="真" w2299 {
              frame False {
              }
              frame True {
                n1561 = property on="A1-position-X" class="DigNum (严格)"() -> (error out=w2308:errorcluster, "Value"=w2315:dbl)  [unwired: 2 in, 1 out]
                n1562 = property on="A1-position-Y" class="DigNum (严格)"(error in=w2308) -> (error out=w2307:errorcluster, "Value"=w2304:dbl)  [unwired: 1 in, 1 out]
                n1563 = Subtract(x=w2304, y=31.5) -> (x-y=w2303:dbl)
                n1564 = Subtract(x=w2315, y=18) -> (x-y=w2306:dbl)
                n1565 = vi-ref "goto.vi"() -> (w2313:refnum<vi>)
                n1566 = property class="VI"(reference=w2313, error in=w2307) -> ("Name"=w2312:string)  [unwired: 2 out]
                n1567 = Open VI Reference(type specifier VI Refnum (for type only)=refnum<vi> refnum, vi path=w2312, options=128) -> (vi reference=w2310:refnum<vi>)  [unwired: 3 in, 1 out]
                n1568 = call-by-ref "Start Asynchronous Call"(reference=w2310, "Y(mm)"=w2303, "X(mm)"=w2306) -> ()  [unwired: 10 in, 3 out]
              }
            }
            n1569 = property on="currentNO" class="Str"("Value"="H5") -> ()  [unwired: 2 in, 2 out]
          }
          event "H6": Value Change {
            n1570 = event-data() -> ("NewVal"=w2317:bool)  [unwired: 1 in, 5 out]
            n1571 = property on="移动" class="Bool (严格)"() -> ("Value"=w2320:bool)  [unwired: 2 in, 2 out]
            n1572 = Not(x=w2320) -> (.not. x?=w2319:bool)
            n1573 = And(x=w2319, y=w2317) -> (x .and. y?=w2318:bool)
            n1574 = case shown="真" w2318 {
              frame False {
              }
              frame True {
                n1575 = property on="A1-position-X" class="DigNum (严格)"() -> (error out=w2327:errorcluster, "Value"=w2334:dbl)  [unwired: 2 in, 1 out]
                n1576 = property on="A1-position-Y" class="DigNum (严格)"(error in=w2327) -> (error out=w2326:errorcluster, "Value"=w2323:dbl)  [unwired: 1 in, 1 out]
                n1577 = Subtract(x=w2323, y=31.5) -> (x-y=w2322:dbl)
                n1578 = Subtract(x=w2334, y=22.5) -> (x-y=w2325:dbl)
                n1579 = vi-ref "goto.vi"() -> (w2332:refnum<vi>)
                n1580 = property class="VI"(reference=w2332, error in=w2326) -> ("Name"=w2331:string)  [unwired: 2 out]
                n1581 = Open VI Reference(type specifier VI Refnum (for type only)=refnum<vi> refnum, vi path=w2331, options=128) -> (vi reference=w2329:refnum<vi>)  [unwired: 3 in, 1 out]
                n1582 = call-by-ref "Start Asynchronous Call"(reference=w2329, "Y(mm)"=w2322, "X(mm)"=w2325) -> ()  [unwired: 10 in, 3 out]
              }
            }
            n1583 = property on="currentNO" class="Str"("Value"="H6") -> ()  [unwired: 2 in, 2 out]
          }
          event "H7": Value Change {
            n1584 = event-data() -> ("NewVal"=w2336:bool)  [unwired: 1 in, 5 out]
            n1585 = property on="移动" class="Bool (严格)"() -> ("Value"=w2339:bool)  [unwired: 2 in, 2 out]
            n1586 = Not(x=w2339) -> (.not. x?=w2338:bool)
            n1587 = And(x=w2338, y=w2336) -> (x .and. y?=w2337:bool)
            n1588 = case shown="真" w2337 {
              frame False {
              }
              frame True {
                n1589 = property on="A1-position-X" class="DigNum (严格)"() -> (error out=w2346:errorcluster, "Value"=w2353:dbl)  [unwired: 2 in, 1 out]
                n1590 = property on="A1-position-Y" class="DigNum (严格)"(error in=w2346) -> (error out=w2345:errorcluster, "Value"=w2342:dbl)  [unwired: 1 in, 1 out]
                n1591 = Subtract(x=w2342, y=31.5) -> (x-y=w2341:dbl)
                n1592 = Subtract(x=w2353, y=27) -> (x-y=w2344:dbl)
                n1593 = vi-ref "goto.vi"() -> (w2351:refnum<vi>)
                n1594 = property class="VI"(reference=w2351, error in=w2345) -> ("Name"=w2350:string)  [unwired: 2 out]
                n1595 = Open VI Reference(type specifier VI Refnum (for type only)=refnum<vi> refnum, vi path=w2350, options=128) -> (vi reference=w2348:refnum<vi>)  [unwired: 3 in, 1 out]
                n1596 = call-by-ref "Start Asynchronous Call"(reference=w2348, "Y(mm)"=w2341, "X(mm)"=w2344) -> ()  [unwired: 10 in, 3 out]
              }
            }
            n1597 = property on="currentNO" class="Str"("Value"="H7") -> ()  [unwired: 2 in, 2 out]
          }
          event "H8": Value Change {
            n1598 = event-data() -> ("NewVal"=w2355:bool)  [unwired: 1 in, 5 out]
            n1599 = property on="移动" class="Bool (严格)"() -> ("Value"=w2358:bool)  [unwired: 2 in, 2 out]
            n1600 = Not(x=w2358) -> (.not. x?=w2357:bool)
            n1601 = And(x=w2357, y=w2355) -> (x .and. y?=w2356:bool)
            n1602 = case shown="真" w2356 {
              frame False {
              }
              frame True {
                n1603 = property on="A1-position-X" class="DigNum (严格)"() -> (error out=w2365:errorcluster, "Value"=w2372:dbl)  [unwired: 2 in, 1 out]
                n1604 = property on="A1-position-Y" class="DigNum (严格)"(error in=w2365) -> (error out=w2364:errorcluster, "Value"=w2361:dbl)  [unwired: 1 in, 1 out]
                n1605 = Subtract(x=w2361, y=31.5) -> (x-y=w2360:dbl)
                n1606 = Subtract(x=w2372, y=31.5) -> (x-y=w2363:dbl)
                n1607 = vi-ref "goto.vi"() -> (w2370:refnum<vi>)
                n1608 = property class="VI"(reference=w2370, error in=w2364) -> ("Name"=w2369:string)  [unwired: 2 out]
                n1609 = Open VI Reference(type specifier VI Refnum (for type only)=refnum<vi> refnum, vi path=w2369, options=128) -> (vi reference=w2367:refnum<vi>)  [unwired: 3 in, 1 out]
                n1610 = call-by-ref "Start Asynchronous Call"(reference=w2367, "Y(mm)"=w2360, "X(mm)"=w2363) -> ()  [unwired: 10 in, 3 out]
              }
            }
            n1611 = property on="currentNO" class="Str"("Value"="H8") -> ()  [unwired: 2 in, 2 out]
          }
          event "H9": Value Change {
            n1612 = event-data() -> ("NewVal"=w2374:bool)  [unwired: 1 in, 5 out]
            n1613 = property on="移动" class="Bool (严格)"() -> ("Value"=w2377:bool)  [unwired: 2 in, 2 out]
            n1614 = Not(x=w2377) -> (.not. x?=w2376:bool)
            n1615 = And(x=w2376, y=w2374) -> (x .and. y?=w2375:bool)
            n1616 = case shown="真" w2375 {
              frame False {
              }
              frame True {
                n1617 = property on="A1-position-X" class="DigNum (严格)"() -> (error out=w2384:errorcluster, "Value"=w2391:dbl)  [unwired: 2 in, 1 out]
                n1618 = property on="A1-position-Y" class="DigNum (严格)"(error in=w2384) -> (error out=w2383:errorcluster, "Value"=w2380:dbl)  [unwired: 1 in, 1 out]
                n1619 = Subtract(x=w2380, y=31.5) -> (x-y=w2379:dbl)
                n1620 = Subtract(x=w2391, y=36) -> (x-y=w2382:dbl)
                n1621 = vi-ref "goto.vi"() -> (w2389:refnum<vi>)
                n1622 = property class="VI"(reference=w2389, error in=w2383) -> ("Name"=w2388:string)  [unwired: 2 out]
                n1623 = Open VI Reference(type specifier VI Refnum (for type only)=refnum<vi> refnum, vi path=w2388, options=128) -> (vi reference=w2386:refnum<vi>)  [unwired: 3 in, 1 out]
                n1624 = call-by-ref "Start Asynchronous Call"(reference=w2386, "Y(mm)"=w2379, "X(mm)"=w2382) -> ()  [unwired: 10 in, 3 out]
              }
            }
            n1625 = property on="currentNO" class="Str"("Value"="H9") -> ()  [unwired: 2 in, 2 out]
          }
          event "H10": Value Change {
            n1626 = event-data() -> ("NewVal"=w2393:bool)  [unwired: 1 in, 5 out]
            n1627 = property on="移动" class="Bool (严格)"() -> ("Value"=w2396:bool)  [unwired: 2 in, 2 out]
            n1628 = Not(x=w2396) -> (.not. x?=w2395:bool)
            n1629 = And(x=w2395, y=w2393) -> (x .and. y?=w2394:bool)
            n1630 = case shown="真" w2394 {
              frame False {
              }
              frame True {
                n1631 = property on="A1-position-X" class="DigNum (严格)"() -> (error out=w2403:errorcluster, "Value"=w2410:dbl)  [unwired: 2 in, 1 out]
                n1632 = property on="A1-position-Y" class="DigNum (严格)"(error in=w2403) -> (error out=w2402:errorcluster, "Value"=w2399:dbl)  [unwired: 1 in, 1 out]
                n1633 = Subtract(x=w2399, y=31.5) -> (x-y=w2398:dbl)
                n1634 = Subtract(x=w2410, y=40.5) -> (x-y=w2401:dbl)
                n1635 = vi-ref "goto.vi"() -> (w2408:refnum<vi>)
                n1636 = property class="VI"(reference=w2408, error in=w2402) -> ("Name"=w2407:string)  [unwired: 2 out]
                n1637 = Open VI Reference(type specifier VI Refnum (for type only)=refnum<vi> refnum, vi path=w2407, options=128) -> (vi reference=w2405:refnum<vi>)  [unwired: 3 in, 1 out]
                n1638 = call-by-ref "Start Asynchronous Call"(reference=w2405, "Y(mm)"=w2398, "X(mm)"=w2401) -> ()  [unwired: 10 in, 3 out]
              }
            }
            n1639 = property on="currentNO" class="Str"("Value"="H10") -> ()  [unwired: 2 in, 2 out]
          }
          event "H11": Value Change {
            n1640 = event-data() -> ("NewVal"=w2412:bool)  [unwired: 1 in, 5 out]
            n1641 = property on="移动" class="Bool (严格)"() -> ("Value"=w2415:bool)  [unwired: 2 in, 2 out]
            n1642 = Not(x=w2415) -> (.not. x?=w2414:bool)
            n1643 = And(x=w2414, y=w2412) -> (x .and. y?=w2413:bool)
            n1644 = case shown="真" w2413 {
              frame False {
              }
              frame True {
                n1645 = property on="A1-position-X" class="DigNum (严格)"() -> (error out=w2422:errorcluster, "Value"=w2429:dbl)  [unwired: 2 in, 1 out]
                n1646 = property on="A1-position-Y" class="DigNum (严格)"(error in=w2422) -> (error out=w2421:errorcluster, "Value"=w2418:dbl)  [unwired: 1 in, 1 out]
                n1647 = Subtract(x=w2418, y=31.5) -> (x-y=w2417:dbl)
                n1648 = Subtract(x=w2429, y=45) -> (x-y=w2420:dbl)
                n1649 = vi-ref "goto.vi"() -> (w2427:refnum<vi>)
                n1650 = property class="VI"(reference=w2427, error in=w2421) -> ("Name"=w2426:string)  [unwired: 2 out]
                n1651 = Open VI Reference(type specifier VI Refnum (for type only)=refnum<vi> refnum, vi path=w2426, options=128) -> (vi reference=w2424:refnum<vi>)  [unwired: 3 in, 1 out]
                n1652 = call-by-ref "Start Asynchronous Call"(reference=w2424, "Y(mm)"=w2417, "X(mm)"=w2420) -> ()  [unwired: 10 in, 3 out]
              }
            }
            n1653 = property on="currentNO" class="Str"("Value"="H11") -> ()  [unwired: 2 in, 2 out]
          }
          event "H12": Value Change {
            n1654 = event-data() -> ("NewVal"=w2431:bool)  [unwired: 1 in, 5 out]
            n1655 = property on="移动" class="Bool (严格)"() -> ("Value"=w2434:bool)  [unwired: 2 in, 2 out]
            n1656 = Not(x=w2434) -> (.not. x?=w2433:bool)
            n1657 = And(x=w2433, y=w2431) -> (x .and. y?=w2432:bool)
            n1658 = case shown="真" w2432 {
              frame False {
              }
              frame True {
                n1659 = property on="A1-position-X" class="DigNum (严格)"() -> (error out=w2441:errorcluster, "Value"=w2448:dbl)  [unwired: 2 in, 1 out]
                n1660 = property on="A1-position-Y" class="DigNum (严格)"(error in=w2441) -> (error out=w2440:errorcluster, "Value"=w2437:dbl)  [unwired: 1 in, 1 out]
                n1661 = Subtract(x=w2437, y=31.5) -> (x-y=w2436:dbl)
                n1662 = Subtract(x=w2448, y=49.5) -> (x-y=w2439:dbl)
                n1663 = vi-ref "goto.vi"() -> (w2446:refnum<vi>)
                n1664 = property class="VI"(reference=w2446, error in=w2440) -> ("Name"=w2445:string)  [unwired: 2 out]
                n1665 = Open VI Reference(type specifier VI Refnum (for type only)=refnum<vi> refnum, vi path=w2445, options=128) -> (vi reference=w2443:refnum<vi>)  [unwired: 3 in, 1 out]
                n1666 = call-by-ref "Start Asynchronous Call"(reference=w2443, "Y(mm)"=w2436, "X(mm)"=w2439) -> ()  [unwired: 10 in, 3 out]
              }
            }
            n1667 = property on="currentNO" class="Str"("Value"="H12") -> ()  [unwired: 2 in, 2 out]
          }
          event "ShutDownSystem": Value Change {
            n1668 = event-data() -> ("NewVal"=w2450:bool)  [unwired: 1 in, 5 out]
            n1669 = case shown="真" w2450 {
              frame False {
              }
              frame True {
                n1670 = flat-sequence {
                  frame #0 {
                    n1671 = call "stop_device.vi"() -> ()  [unwired: 11 in, 1 out]
                  }
                  frame #1 {
                    n1672 = property on="stop" class="Bool (严格)"("Value"=TRUE ("stop")) -> ()  [unwired: 2 in, 2 out]
                  }
                }
              }
            }
          }
        }
        n1673 = property on="stop" class="Bool (严格)"() -> ("Value"=w176:bool)  [unwired: 2 in, 2 out]
      }
      n1674 = while {
        tunnel: w90 -> [w93]
        stop <- w92 stop-if-true
        n1675 = event shown="[2] <motor status>: 用户事件" {
          selector: w93 -> [_ _ _ _]
          dyn-events: _ -> [_ _ _ _]
          timeout: _ -> [_ _ _ _]
          event Timeout {
            n1676 = event-data() -> ()  [unwired: 1 in, 3 out]
          }
          event User Event {
            n1677 = event-data() -> ("AI"=w95:dbl[], "DI"=w94:bool[])  [unwired: 1 in, 4 out]
            n1678 = Index Array(array=w95, index=0) -> (element=w113:dbl)
            n1679 = Index Array(array=w94, index=0) -> (element=→"X0":bool)
            n1680 = Divide(x=w113, y=10.0) -> (x/y=w115:dbl)
            n1681 = Multiply(x=w115, y=2000.0) -> (x*y=w117:dbl)
            n1682 = property on="MCPHV-Real" class="DigNum (严格)"("Value"=w117) -> (error out=w96:errorcluster)  [unwired: 2 in, 1 out]
            n1683 = Index Array(array=w94, index=4) -> (element=→"Y0":bool)
            n1684 = Index Array(array=w95, index=1) -> (element=w118:dbl)
            n1685 = Divide(x=w118, y=10.0) -> (x/y=w120:dbl)
            n1686 = Multiply(x=w120, y=20000.0) -> (x*y=w122:dbl)
            n1687 = Index Array(array=w94, index=1) -> (element=→"X满":bool)
            n1688 = property on="Tar.HV-Real" class="DigNum (严格)"(error in=w96, "Value"=w122) -> (error out=w97:errorcluster)  [unwired: 1 in, 1 out]
            n1689 = Index Array(array=w95, index=2) -> (element=w123:dbl)
            n1690 = Index Array(array=w94, index=3) -> (element=→"Y标":bool)
            n1691 = Divide(x=w123, y=10.0) -> (x/y=w125:dbl)
            n1692 = Multiply(x=w125, y=2000.0) -> (x*y=w127:dbl)
            n1693 = property on="Pul.HV-Real" class="DigNum (严格)"(error in=w97, "Value"=w127) -> (error out=w98:errorcluster)  [unwired: 1 in, 1 out]
            n1694 = Index Array(array=w95, index=3) -> (element=w128:dbl)
            n1695 = Index Array(array=w94, index=2) -> (element=→"Y满":bool)
            n1696 = Divide(x=w128, y=10.0) -> (x/y=w130:dbl)
            n1697 = Multiply(x=w130, y=10000.0) -> (x*y=w132:dbl)
            n1698 = property on="LensHV-Real" class="DigNum (严格)"(error in=w98, "Value"=w132) -> (error out=w134:errorcluster)  [unwired: 1 in, 1 out]
            n1699 = Index Array(array=w95, index=19) -> (element=w136:dbl)
            n1700 = Subtract(x=w136, y=3.572) -> (x-y=w138:dbl)
            n1701 = Divide(x=w138, y=1.286) -> (x/y=w140:dbl)
            n1702 = Power Of 10(x=w140) -> (10^x=w141:dbl)
            n1703 = Index Array(array=w95, index=18) -> (element=w142:dbl)
            n1704 = Subtract(x=w142, y=8.5) -> (x-y=w144:dbl)
            n1705 = property on="Lvaccum" class="DigNum (严格)"(error in=w134, "Value"=w141) -> (error out=w146:errorcluster)  [unwired: 1 in, 1 out]
            n1706 = Power Of 10(x=w144) -> (10^x=w145:dbl)
            n1707 = property on="Hvaccum" class="DigNum (严格)"(error in=w146, "Value"=w145) -> ()  [unwired: 1 in, 2 out]
          }
          event User Event {
            n1708 = event-data() -> ("status"=w147:string)  [unwired: 1 in, 5 out]
            n1709 = case shown="\"stop\", 默认" w147 {
              frame "stop", Default {
                n1710 = property on="GO" class="Bool (严格)"("DisabledEnum"=T6."Enabled" ("Disabled")) -> (error out=w149:errorcluster)  [unwired: 2 in, 1 out]
                n1711 = property on="移动" class="Bool (严格)"(error in=w149, "Value"=FALSE ("移动")) -> ()  [unwired: 1 in, 2 out]
              }
              frame "moving" {
                n1712 = property on="GO" class="Bool (严格)"("DisabledEnum"=T6."Disabled and Grayed Out" ("Disabled")) -> (error out=w152:errorcluster)  [unwired: 2 in, 1 out]
                n1713 = property on="移动" class="Bool (严格)"(error in=w152, "Value"=TRUE ("移动")) -> ()  [unwired: 1 in, 2 out]
              }
            }
          }
          event User Event {
            n1714 = event-data() -> ("source"=w154:string, "value"=w155:dbl)  [unwired: 1 in, 4 out]
            n1715 = case shown="\"X\"" w154 {
              tunnel: w155 -> [w162 w170]
              tunnel: [w164 w171] -> w161
              frame "Y", Default {
                n1716 = property on="X当前" class="DigNum (严格)"() -> ("Value"=w166:dbl)  [unwired: 2 in, 2 out]
                n1717 = Multiply(x=w162, y=1000.0) -> (x*y=w167:dbl)
                n1718 = Divide(x=w166, y=1000.0) -> (x/y=w163:dbl)
                n1719 = Build Array "Build Array"(w163, w162) -> (w164:dbl[])
                n1720 = property on="Y当前" class="DigNum (严格)"("Value"=w167) -> ()  [unwired: 2 in, 2 out]
              }
              frame "X" {
                n1721 = property on="Y当前" class="DigNum (严格)"() -> ("Value"=w173:dbl)  [unwired: 2 in, 2 out]
                n1722 = Multiply(x=w170, y=1000.0) -> (x*y=w174:dbl)
                n1723 = Divide(x=w173, y=1000.0) -> (x/y=w169:dbl)
                n1724 = property on="X当前" class="DigNum (严格)"("Value"=w174) -> ()  [unwired: 2 in, 2 out]
                n1725 = Build Array(w170, w169) -> (w171:dbl[])
              }
            }
            n1726 = Current VI's Path() -> (path=w158:path)
            n1727 = Strip Path(path=w158) -> (stripped path=w159:path)  [unwired: 1 out]
            n1728 = Build Path(base path=w159, name or relative path="last_position") -> (appended path=w157:path)
            n1729 = call-poly <vilib>:"Write To Spreadsheet File.vi"("format (%.3f)"="%.9f", "1D data"=w161, "file path (dialog if empty)"=w157) -> ()  [unwired: 5 in, 1 out]
          }
        }
        n1730 = property on="stop" class="Bool (严格)"() -> ("Value"=w92:bool)  [unwired: 2 in, 2 out]
      }
    }
  }
  n1731 = Unbundle(w22) -> ("tasks"=w4:T9, "interface"=w3:T8, "error out"=w2:errorcluster)
  n1732 = call "USB6343_Control_v1.6.2.vi"("error in"=w2, "interface"=w3, "tasks"=w4) -> ()  [unwired: 9 in]
  n1733 = call <vilib>:"IMAQdx Enumerate Cameras.vi"() -> ("error out"=w13:errorcluster, "Camera Information Array"=w10:T14)  [unwired: 10 in]
  n1734 = Index Array(array=w10, index=0) -> (element=w12:T15)
  n1735 = Unbundle By Name(w12) -> ("InterfaceName"=w20:string)
  n1736 = call <vilib>:"IMAQdx Open Camera.vi"("error in"=w13, "Session In"=w20) -> ("error out"=w7:errorcluster, "Session Out"=w8:T16)  [unwired: 8 in]
  n1737 = property class="IMAQdx" props=["VideoMode", "Width", "Height"](reference=w8, error in=w7, "VideoMode"=u32 13) -> (reference out=w6:T16, error out=w5:errorcluster)  [unwired: 2 out]
  n1738 = call "IMAQ Create"("Image Name"=w20) -> ("New Image"=w15:T3)  [unwired: 4 in, 1 out]
  n1739 = call <vilib>:"IMAQdx Configure Grab.vi"("error in"=w5, "Session In"=w6) -> ("error out"=w19:errorcluster, "Session Out"=w14:T16)  [unwired: 8 in]
  n1740 = while {
    tunnel: w19 -> [w2458]
    tunnel: w14 -> [w2457]
    tunnel: w15 -> [w2456]
    tunnel: [w2455] -> w16
    tunnel: [w2454] -> w17
    tunnel: [w2453] -> w18
    stop <- w2452 stop-if-true
    n1741 = call <vilib>:"IMAQdx Grab.vi"("error in"=w2458, "Image In"=w2456, "Session In"=w2457) -> ("error out"=w2455:errorcluster, "Image Out"=w2453:T3, "Session Out"=w2454:T16)  [unwired: 5 in, 1 out]
    "Image" <- w2453
    n1742 = property on="stop" class="Bool (严格)"() -> ("Value"=w2452:bool)  [unwired: 2 in, 2 out]
  }
  n1743 = call "IMAQ Dispose"("Image"=w18) -> ()  [unwired: 5 in, 1 out]
  n1744 = call <vilib>:"IMAQdx Close Camera.vi"("error in"=w16, "Session In"=w17) -> ()  [unwired: 9 in, 1 out]
